vi "SqK_2017.vi"() -> ()   [LabVIEW 2014]
uses:
  <vilib>/vision/Image Controls.llb/IMAQ Image.ctl
  <vilib>/Utility/sysdir.llb/System Directory Type.ctl
  <vilib>/Utility/file.llb/Read From Spreadsheet File (string).vi
  <vilib>/Utility/file.llb/Read From Spreadsheet File (I64).vi
panel:
  out "Video 2":T1(plugin-control)
  out "Boast 13":u8(slide) scale=0.0..54.0
  out "Lob 2":u8(slide) scale=0.0..54.0
  out "Drop 13":u8(slide) scale=0.0..54.0
  out "Boast 1":u8(slide) scale=0.0..54.0
  out "Lob 1":u8(slide) scale=0.0..54.0
  out "Drop 1":u8(slide) scale=0.0..54.0
  in  "Boolean":bool
  out "Min":dbl
  out "sec":dbl
  out "milsec":dbl
  in  "Ddrive":bool
  in  "ASWdrive":bool
  in  "DSWdrive":bool
  in  "SWADrive 12":bool
  in  "SWADrive 11":bool
  in  "SWADrive 10":bool
  in  "SWADrive 9":bool
  in  "SWDDrive 12":bool
  in  "SWDDrive 11":bool
  in  "SWDDrive 10":bool
  in  "SWDDrive 9":bool
  in  "DDrive 12":bool
  in  "DDrive 11":bool
  in  "DDrive 10":bool
  in  "DDrive 9":bool
  in  "DDrive 8":bool
  in  "DDrive 7":bool
  in  "DDrive 6":bool
  in  "DDrive 5":bool
  in  "DDrive":bool
  in  "DDrive 2":bool
  in  "DDrive 3":bool
  in  "DDrive 4":bool
  in  "SWDDrive 8":bool
  in  "SWDDrive 7":bool
  in  "SWDDrive 6":bool
  in  "SWDDrive 5":bool
  in  "SWDDrive":bool
  in  "SWDDrive 2":bool
  in  "SWDDrive 3":bool
  in  "SWDDrive 4":bool
  in  "SWADrive 8":bool
  in  "SWADrive 7":bool
  in  "SWADrive 6":bool
  in  "SWADrive 5":bool
  in  "SWADrive":bool
  in  "SWADrive 2":bool
  in  "SWADrive 3":bool
  in  "SWADrive 4":bool
  out "last saved data":i64[](array[numeric])
  out "Btn 10":string
  out "Btn 9":string
  out "Btn 8":string
  out "Btn 7":string
  out "Btn 6":string
  out "Player 2 data":i64[](array[numeric])
  out "player 1 data":i64[](array[numeric])
  out "both player data":i64[](array[numeric])
  out "Edited data":i64[][](array[numeric])
  out "Event After":i64[][](array[numeric])
  out "Event before":i64[][](array[numeric])
  out "result":i32[](array[numeric])
  out "EVENTS\nTO PLAY":i32[](array[numeric])
  out "Combined data":i64[][](array[numeric])
  out "Extra":i16
  out "Score change":bool[](array[boolean])
  out "last row":i32[](array[numeric])
  out "Player 1/2":i16
  out "Service":i16
  out "Cross":i16
  out "Straight":i16
  out "position":i16
  out "Main tab 2":T2(ring)
  in  "fast rewind":bool
  in  "START":bool
  out "frames to write":i64[][](array[numeric])
  in  "Data file":path caption="Data"
  in  "playback speed":dbl(slide)=1.0 min=0.25 max=1.5 step=0.25 scale=0.25..1.5
  in  "Main tab":enum32{"Coding", "Display"}(tab)
  in  "Player 2":string
  in  "Let":bool
  in  "Nolet1":bool
  in  "Nolet2":bool
  in  "Stroke1":bool
  in  "Stroke2":bool
  in  "Expected Winner1":bool
  in  "Expected Winner2":bool
  in  "Unexpected Winner1":bool
  in  "Unexpected Winner2":bool
  in  "Forced Error1":bool
  in  "Unforced Error1":bool
  in  "Forced Error2":bool
  in  "Unforced Error2":bool
  in  "Pause lag(s)":dbl=1.0 min=0.0 max=2.0 step=0.5 format="%#.1g"
  in  "Code lag(s)":dbl=1.0 min=0.0 max=5.0 step=0.5 format="%#.1g"
  in  "Link Errors":bool
  in  "Btn 1":string
  in  "Btn 2":string
  in  "Btn 3":string
  in  "Btn 4":string
  in  "Btn 5":string
  in  "Button 1":bool
  in  "Button 2":bool
  in  "Button 3":bool
  in  "Button 4":bool
  in  "Button 5":bool
  out "P2":i32
  out "P1":i32
  out "Player1/Player2":bool[](array[boolean])
  in  "Player2":bool
  in  "Player1":bool
  in  "Auto switch":bool
  in  "S6":bool
  in  "S5":bool
  in  "S4":bool
  in  "S3":bool
  in  "S2":bool
  in  "Service1":bool
  in  "Service2":bool
  in  "S1":bool
  in  "5 4":bool
  in  "5 3":bool
  in  "5 2":bool
  in  "5 1":bool
  in  "6 4":bool
  in  "6 3":bool
  in  "6 2":bool
  in  "6 1":bool
  in  "4 4":bool
  in  "4 3":bool
  in  "4 2":bool
  in  "4 1":bool
  in  "3 4":bool
  in  "3 3":bool
  in  "3 2":bool
  in  "3 1":bool
  in  "2 4":bool
  in  "2 3":bool
  in  "2 2":bool
  in  "2 1":bool
  in  "1 4":bool
  in  "1 3":bool
  in  "1 2":bool
  in  "1 1":bool
  in  "after 2":u8(slide)=2 scale=0.0..5.0
  in  "before 2":u8(slide)=2
  in  "Pause lag on":bool
  in  "Undo":bool
  in  "Player 1":string
  in  "ADrive 2":bool
  in  "ADrive":bool
  in  "Drop 2":bool
  in  "lob 2":bool
  in  "Boast 2":bool
  in  "Drop":bool
  in  "lob 13":bool
  in  "Boast":bool
  in  "Chop 2":bool
  in  "Chop":bool
  in  "Smash 2":bool
  in  "Smash":bool
  in  "ADrive 4":bool
  in  "ADrive 3":bool
  in  "Drop 4":bool
  in  "lob 4":bool
  in  "Boast 4":bool
  in  "Drop 3":bool
  in  "lob 3":bool
  in  "Boast 3":bool
  in  "Chop 4":bool
  in  "Chop 3":bool
  in  "Smash 4":bool
  in  "Smash 3":bool
  in  "ADrive 9":bool
  in  "ADrive 10":bool
  in  "Chop 9":bool
  in  "Chop 10":bool
  in  "Drop 9":bool
  in  "lob 9":bool
  in  "Drop 10":bool
  in  "lob 10":bool
  in  "Smash 9":bool
  in  "Smash 10":bool
  in  "Boast 9":bool
  in  "Boast 10":bool
  in  "ADrive 11":bool
  in  "ADrive 12":bool
  in  "Chop 11":bool
  in  "Chop 12":bool
  in  "Drop 11":bool
  in  "lob 11":bool
  in  "Drop 12":bool
  in  "lob 12":bool
  in  "Smash 11":bool
  in  "Smash 12":bool
  in  "Boast 11":bool
  in  "Boast 12":bool
  in  "Smash 8":bool
  in  "Smash 7":bool
  in  "Chop 8":bool
  in  "Chop 7":bool
  in  "Boast 7":bool
  in  "lob 8":bool
  in  "Drop 8":bool
  in  "lob 7":bool
  in  "Drop 7":bool
  in  "Boast 8":bool
  in  "ADrive 8":bool
  in  "ADrive 7":bool
  in  "Smash 6":bool
  in  "Smash 5":bool
  in  "Chop 6":bool
  in  "Chop 5":bool
  in  "Boast 5":bool
  in  "Boast 6":bool
  in  "lob 6":bool
  in  "Drop 6":bool
  in  "lob 5":bool
  in  "Drop 5":bool
  in  "ADrive 6":bool
  in  "ADrive 5":bool
  in  "set":u16(ring) items=["Game 1", "Game 2", "Game 3", "Game 4", "Game 5"]
  in  "Tab Control":T3(tab)
  out "1 9":string
  out "1 11":string
  out "1 12":string
  out "1 13":string
  out "1 8":string
  out "1 15":string
  out "1 16":string
  out "1 17":string
  out "1 18":string
  out "1 19":string
  out "1 20":string
  out "1 21":string
  out "1 23":string
  out "1 24":string
  out "1 25":string
  out "1 26":string
  out "1 27":string
  out "1 28":string
  out "1 29":string
  out "1 30":string
  out "1 31":string
  out "1 33":string
  out "1 34":string
  out "1 35":string
  out "1 36":string
  out "1 37":string
  out "1 38":string
  out "1 39":string
  out "1 40":string
  out "1 41":string
  out "1 43":string
  out "1 44":string
  out "1 45":string
  out "1 46":string
  out "1 47":string
  out "1 48":string
  out "1 49":string
  out "1 50":string
  out "1 51":string
  out "1 52":string
  out "1 53":string
  out "1 54":string
  out "1 55":string
  out "1 56":string
  out "1 57":string
  out "1 58":string
  out "1 59":string
  out "1 60":string
  out "Volley 1":string="0"
  out "Straight 1":string="0"
  out "Bounce 1":string="0"
  out "Cross 1":string="0"
  out "B-hand 1":string="0"
  out "F-hand 1":string="0"
  out "H-volley 1":string="0"
  in  "Fh":string="Forehand"
  in  "BH 3":string="Backhand"
  in  "Cross 5":string="Cross"
  in  "bounce":string="Bounce"
  in  "Straight 5":string="Straight"
  in  "volley":string="Volley"
  in  "H-volley":string="Half volley"
  out "H-volley 3":string="0"
  out "Volley 3":string="0"
  out "Straight 3":string="0"
  out "Bounce 3":string="0"
  out "Cross 3":string="0"
  out "B-hand 2":string="0"
  out "F-hand 2":string="0"
  in  "H-volley 2":string="Half volley"
  in  "volley 2":string="Volley"
  in  "Straight 6":string="Straight"
  in  "bounce 2":string="Bounce"
  in  "Cross 6":string="Cross"
  in  "BH 4":string="Backhand"
  in  "Fh 2":string="Forehand"
  out "UF err1 num":string="0"
  out "F err1 num":string="0"
  out "UNex win1 num":string="0"
  out "ex win1 num":string="0"
  in  "UNex win1":string="Unexpected winner"
  in  "ex win1":string="Expected winner"
  out "Stroke 3":string="0"
  in  "Stroke 1":string="Stroke"
  in  "UF err1":string="Unforced error"
  in  "F err1":string="Forced error"
  out "Let 3":string="0"
  out "No Let 1":string="0"
  in  "Let 1":string="Let "
  in  "No let 1":string="No let"
  out "UF err2 num":string="0"
  out "F err2 num":string="0"
  out "UNex win2 num":string="0"
  out "ex win2 num":string="0"
  in  "UF err2":string="Unforced error"
  in  "F err2":string="Forced error"
  in  "UNex win2":string="Unexpected winner"
  in  "ex win2":string="Expected winner"
  out "Stroke 4":string="0"
  out "Let 4":string="0"
  out "No Let 2":string="0"
  in  "Stroke 2":string="Stroke"
  in  "Let  5":string="Let"
  in  "No let 2":string="No let"
  out "Volley 4":u8(slide) scale=0.0..54.0
  out "Bounce 4":u8(slide) scale=0.0..54.0
  out "Cross 4":u8(slide) scale=0.0..54.0
  out "Straight 4":u8(slide) scale=0.0..54.0
  out "BH 1":u8(slide) scale=0.0..54.0
  out "FH 1":u8(slide) scale=0.0..54.0
  out "Drive 1":u8(slide) scale=0.0..54.0
  out "Player 1 shots numbers":string[](array[string])=["0", "0", "0", "0", "", " ", "0", "0", "", "0", "0", "", "0", "0"]
  in  "Player 1 shots":string[](array[string])=["Drive", "Drop", "Chop", "Lob", "Boast 2", "Boast 3", "Kill", "", "", "", "", "", "F-hand", "B-hand", "", "Straight", "Cross", "", "Bounce", "Volley", "H-volley"]
  out "Volley 2":u8(slide) scale=0.0..54.0
  out "Bounce 2":u8(slide) scale=0.0..54.0
  out "Cross 2":u8(slide) scale=0.0..54.0
  out "Straight 2":u8(slide) scale=0.0..54.0
  out "BH 2":u8(slide) scale=0.0..54.0
  out "FH 2":u8(slide) scale=0.0..54.0
  out "Drive 2":u8(slide) scale=0.0..54.0
  out "Player 2 shots numbers":string[](array[string])=["0", "0", "0", "0", "", " ", "0", "0", "", "0", "0", "", "0", "0"]
  in  "Player 2 shots":string[](array[string])=["Drive", "Drop", "Chop", "Lob", "Boast 2", "Boast 3", "Kill", "", "", "", "", "", "F-hand", "B-hand", "", "Straight", "Cross", "", "Bounce", "Volley", "H-volley"]
  in  "before n after":i32(slide) scale=-5.0..5.0
  in  "display\nselection":string(combo)="1"
  in  "Extract data":bool
  in  "Upload edited video":bool
  in  "1 10":bool
  in  "1 7":bool
  in  "1 6":bool
  in  "1 5":bool
  in  "2 10":bool
  in  "2 7":bool
  in  "2 6":bool
  in  "2 5":bool
  in  "3 9":bool
  in  "3 7":bool
  in  "3 6":bool
  in  "3 5":bool
  in  "4 9":bool
  in  "4 7":bool
  in  "4 6":bool
  in  "4 5":bool
  in  "Boast3":bool
  in  "Boast2":bool
  in  "Drop 14":bool
  in  "Chop 13":bool
  in  "Adrive":bool
  in  "Lob":bool
  in  "Smash 13":bool
  in  "FH":bool
  in  "BH":bool
  in  "ST":bool
  in  "CR":bool
  in  "Bounce":bool
  in  "Half Volley":bool
  in  "Volley":bool
  in  "before":u8(slide)=2
  in  "after":u8(slide)=2 scale=0.0..5.0
  in  "Combine":bool
  in  "Player2 2":bool
  in  "Player1 2":bool
  in  "S6 2":bool
  in  "S5 2":bool
  in  "S4 2":bool
  in  "S1 2":bool
  in  "Service2 2":bool
  in  "Service1 2":bool
  in  "S2 2":bool
  in  "S3 2":bool
  in  "Let 2":bool
  in  "Nolet2 2":bool
  in  "Nolet1 2":bool
  in  "Stroke2 2":bool
  in  "Stroke1 2":bool
  in  "Unforced Error2 2":bool
  in  "Forced Error2 2":bool
  in  "Unforced Error1 2":bool
  in  "Forced Error1 2":bool
  in  "Unexpected Winner2 2":bool
  in  "Unexpected Winner1 2":bool
  in  "Expected Winner2 2":bool
  in  "Expected Winner1 2":bool
  out "Video files to write":string[](array[string])
  in  "Video compress":bool=TRUE
  in  "Abort":bool
  in  "Write file":bool
  in  "Delete":bool[](array[boolean])
  out "Writing":u32(slide) scale=0.0..404.0
  in  "File name":string
  in  "Add to lib":bool
  in  "Video to write":path caption="Folder"
  in  "Examine code":bool
  in  "Update":bool
  in  "Reset":bool
  in  "Code number display":i32 min=1 max=1
  in  "Next":bool
  in  "Previous":bool
  in  "6 5":bool
  in  "6 6":bool
  in  "6 7":bool
  in  "6 8":bool
  in  "5 5":bool
  in  "5 6":bool
  in  "5 7":bool
  in  "5 8":bool
  in  "Button 7":bool
  in  "Button 8":bool
  in  "Button 9":bool
  in  "Button 10":bool
  in  "Button 6":bool
  in  "playback interval on":bool
  in  "clear all":bool
  in  "G5":bool
  in  "G4":bool
  in  "G1":bool
  in  "G2":bool
  in  "G3":bool
  in  "Load video":bool
  in  "Play":bool
  out "ful video frames":i64[](array[numeric])
  out "playback speed":dbl
  out "Number of Frames":u32
  out "framesPerSecond":u32
  out "Last Edit":bool[](array[boolean])
  out "frames 2 play":i64[](array[numeric])
  in  "stop":bool
  out "Video Frame":u32
  out "edited\nevents":i64[][](array[numeric])
  out "edited to play":i64[](array[numeric])
  out "frames edited":i64[](array[numeric])
  in  "fast forward":bool
  in  "Pause":bool
  out "coding":i64[][](array[numeric])
  in  "Progress...":u32(slide) min=400 max=47374 scale=-1.1..56740.0
  in  "Video file":path caption="Video"
  out "task":i32(slide) scale=0.0..300.0
  out "Video":T1(plugin-control)
  # "© 2016 National Sports Institute of Malaysia All Rights Reserved"
  # "Position"
  # "Bounce"
  # "Volley"
  # "Half volley"
  # "Forehand"
  # "Backhand"
  # "Backhand"
  # "Forehand"
  # "Backhand"
  # "Forehand"
  # "St"
  # "Cr"
  # "St"
  # "Cr"
  # "St"
  # "Cr"
  # "St"
  # "Cr"
  # "St"
  # "Cr"
  # "St"
  # "Cr"
  # "Drop"
  # "Chop"
  # "Lob"
  # "Boast"
  # "Kill"
  # "Drive"
  # "Lead and lag settings"
  # "Game"
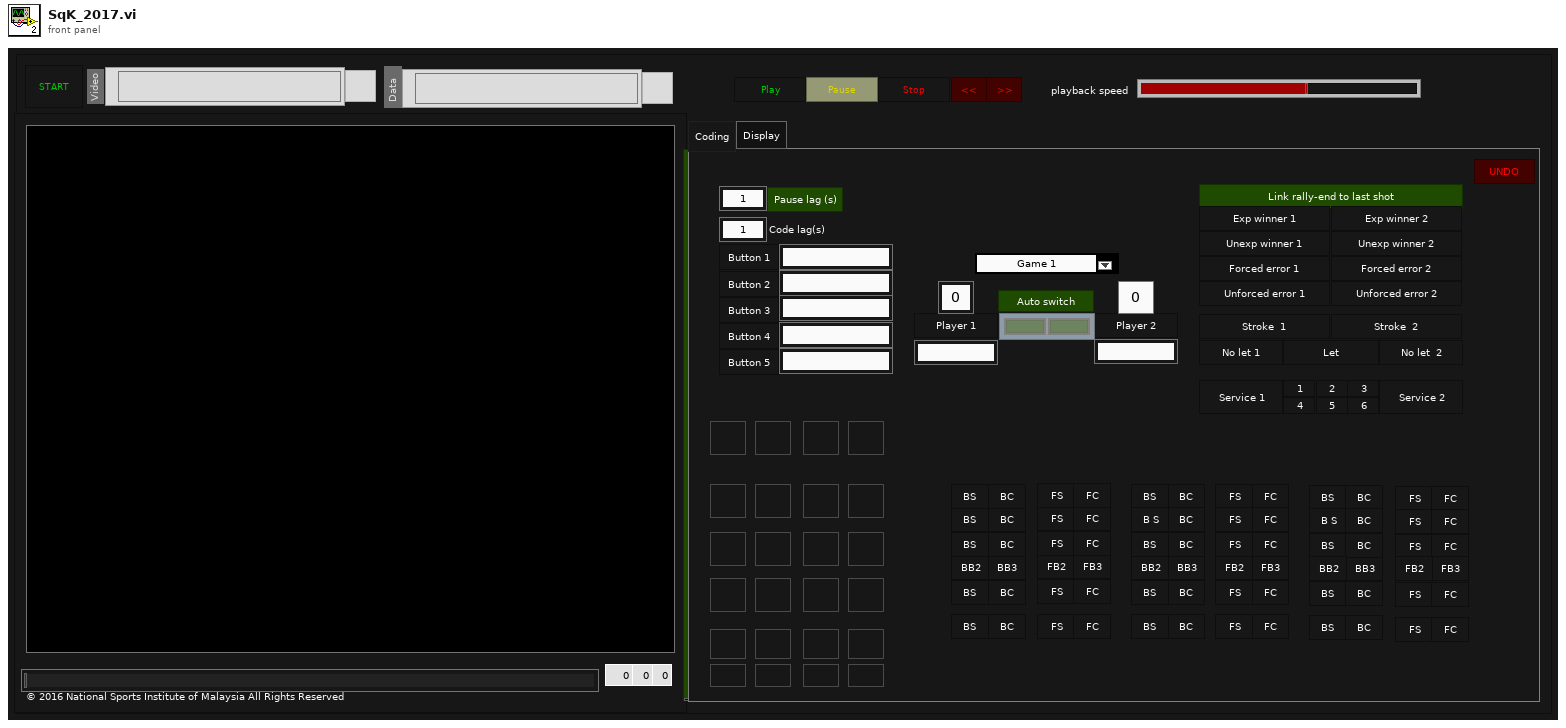
[diagram p1: front panel]
types:
  T1 = typedef "IMAQ Image.ctl" = refnum<image>
  T2 = enum32{"Coding", "Edit video", "Examine coding", "Display", "Update coding", "Edit coding"}
  T3 = enum32{"                                                                       click here to copy"}
  T4 = enum16{"open", "replace", "create", "open or create", "replace or create", "replace or create with confirmation"}
  T5 = enum8{"Enabled", "Disabled", "Disabled and Grayed Out"}
  T6 = enum32{"Coding", "Edit video", "Examine coding", "Display", "Update coding", "Edit coding", "Clear all"}
  T7 = typedef "System Directory Type.ctl" = i32
  T8 = typedef "Image Type" = u32
  T9 = typedef "AviRefnum.ctl" = refnum<k1>
  T10 = cluster{"width":u32, "height":u32, "framesPerSecond":u32, "compressionFilter":string, "hasData":bool}
  T11 = typedef "eventvkey.ctl" = enum16{"ASCII", "Enter", "Return", "Shift", "Ctrl", "Alt", "Cmd", "Opt", "Caps", "NumLock", "Clear", "Break", "Up", "Down", "Left", "Right", "Insert", "Delete", "Home", "End", "PageUp", "PageDown", "Escape", "Help", "Pause", "ScrollLock", "F1", "F2", "F3", "F4", "F5", "F6", "F7", "F8", "F9", "F10", "F11", "F12", "F13", "F14", "F15", "F16", "F17", "F18", "F19", "F20", "F21", "F22", "F23", "F24", "Play", "VolumeUp", "VolumeDown", "Mute", "Two Byte Char"}
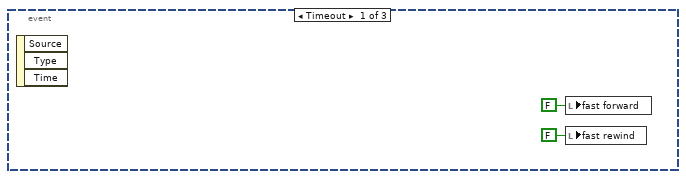
[diagram p2: hidden frame]
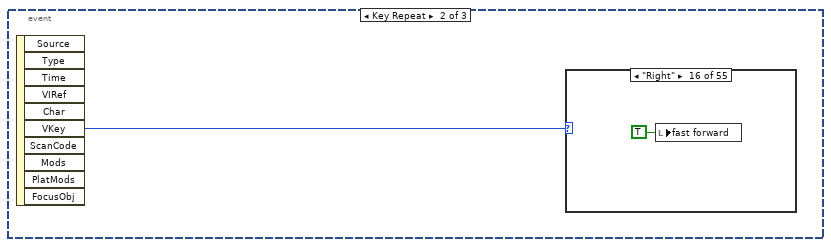
[diagram p3: hidden frame]
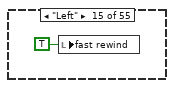
[diagram p18: hidden frame]
diagram:
  w1 = FALSE ("player2")
  n1 = while {
    stop <- FALSE stop-if-true
    n2 = flat-sequence {
      tunnel: [w43] -> w14
      tunnel: [w44] -> w15
      tunnel: w15 -> [w141]
      tunnel: w14 -> [w140]
      tunnel: [w140] -> w13
      tunnel: [w141] -> w12
      tunnel: w13 -> [w196]
      tunnel: w12 -> [w180]
      tunnel: [w169] -> w10
      tunnel: [w179] -> w9
      tunnel: [w178] -> w8
      tunnel: [w177] -> w2
      tunnel: [w176] -> w7
      frame #0 {
        w33 = T7 1 items=["User Home"=0, "User Desktop"=1, "User Documents"=2, "User Application Data"=3, "User Preferences"=4, "User Temporary"=5, "Public Documents"=6, "Public Application Data"=7, "Public Preferences"=8, "Public Cache"=13, "System Core Libraries"=9, "System Installed Libraries"=10, "Application Files"=11, "Boot Volume Root"=12] ("system directory type")
        w36 = T5."Enabled" ("Disabled")
        w38 = u32 0 ("Progress...")
        w35 = FALSE ("START")
        w34 = T5."Disabled and Grayed Out" ("Disabled")
        n3 = call <vilib>:"Get System Directory.vi"("system directory type"=w33) -> ("system directory"=w32:path)  [unwired: 10 in]
        n4 = property on="Video file" class="Path"("StartPath"=w32) -> ()  [unwired: 2 in, 2 out]
        n5 = property on="Video to write" class="Path"("StartPath"=w32) -> ()  [unwired: 2 in, 2 out]
        n6 = property on="Data file" class="Path"("StartPath"=w32) -> ()  [unwired: 2 in, 2 out]
        n7 = property on="Play" class="Bool (strict)"("DisabledEnum"=w34, "Value"=w35) -> ()  [unwired: 2 in, 2 out]
        n8 = property on="stop" class="Bool (strict)"("DisabledEnum"=w34, "Value"=w35) -> ()  [unwired: 2 in, 2 out]
        n9 = property on="Pause" class="Bool (strict)"("DisabledEnum"=w34, "Value"=w35) -> ()  [unwired: 2 in, 2 out]
        n10 = property on="fast forward" class="Bool (strict)"("DisabledEnum"=w34, "Value"=w35) -> ()  [unwired: 2 in, 2 out]
        n11 = property on="playback speed" class="Slide (strict)"("DisabledEnum"=w34, "Value"=1.0 ("playback speed")) -> ()  [unwired: 2 in, 2 out]
        n12 = property on="Main tab" class="TabCtl (strict)"("DisabledEnum"=w34, "Value"=enum32{"Coding", "Display"}."Coding" ("Main tab")) -> ()  [unwired: 2 in, 2 out]
        n13 = property on="Progress..." class="Slide (strict)"("DisabledEnum"=w34, "Value"=w38) -> ()  [unwired: 2 in, 2 out]
        n14 = property on="Video Frame" class="DigNum (strict)"("DisabledEnum"=w34, "Value"=w38) -> ()  [unwired: 2 in, 2 out]
        n15 = property on="Video" class="ImageControl"("DisabledEnum"=w34, "Value"=T1 refnum ("Video")) -> ()  [unwired: 2 in, 2 out]
        n16 = property on="START" class="Bool (strict)"("DisabledEnum"=w36, "Value"=w35) -> ()  [unwired: 2 in, 2 out]
        n17 = property on="Video file" class="Path"("DisabledEnum"=w36) -> ()  [unwired: 2 in, 2 out]
        n18 = property on="Data file" class="Path"("DisabledEnum"=w36) -> ()  [unwired: 2 in, 2 out]
        n19 = property on="fast rewind" class="Bool (strict)"("DisabledEnum"=w34, "Value"=w35) -> ()  [unwired: 2 in, 2 out]
      }
      frame #1 {
        n20 = while {
          tunnel: [w46] -> w44
          tunnel: [w45] -> w43
          stop <- w47 stop-if-true
          n21 = case shown="True" "START" {
            tunnel: [FALSE w52] -> w47
            tunnel: [w49 w55] -> w46
            tunnel: [w49 w54] -> w45
            frame False {
              w49 = path "" ("dup path")
              n22 = Wait (ms)(milliseconds to wait=u32 200) -> ()  [unwired: 1 out]
            }
            frame True {
              n23 = Path To String(path="Data file") -> (string=w64:string)
              n24 = Wait (ms)(milliseconds to wait=u32 200) -> ()  [unwired: 1 out]
              n25 = Empty String/Path?(string/path=w64) -> (empty?=w63:bool)
              n26 = case shown="False" w63 {
                tunnel: "Data file" -> [w85 w110]
                tunnel: [w84 FALSE] -> w61
                tunnel: [w83 w110] -> w54
                frame False {
                  n27 = Strip Path(path=w85) -> (stripped path=w90:path)  [unwired: 1 out]
                  n28 = Path To String(path=w90) -> (string=w89:string)
                  n29 = call <vilib>:"Get File Extension.vi"("file"=w85) -> ("filename without extension"=w92:string)  [unwired: 7 in, 3 out]
                  n30 = Concatenate Strings(w89, "\\" ("string"), w92, ".xls" ("string")) -> (w91:string)
                  n31 = String To Path(string=w91) -> (path=w86:path)
                  n32 = call <vilib>:"Check if File or Folder Exists.vi"("path"=w86) -> ("file or folder exists?"=w87:bool)  [unwired: 8 in, 2 out]
                  n33 = case shown="False" w87 {
                    selector: w87 -> [_ w109]
                    tunnel: w86 -> [w96 w108]
                    tunnel: [w95 w109] -> w84
                    tunnel: [w94 w108] -> w83
                    frame False {
                      n34 = Two Button Dialog(message="This data file does not exist.\nDo you wish to start a new project?", 1:"No" ("F button name (\"Cancel\")"), 2:"Yes" ("T button name (\"OK\")")) -> (T button?=w97:bool)
                      n35 = case shown="False" w97 {
                        selector: w97 -> [w102 w104]
                        tunnel: w96 -> [_ w103]
                        tunnel: [w102 w104] -> w95
                        tunnel: [path "" ("dup path") w103] -> w94
                        frame False {
                        }
                        frame True {
                          n36 = Open/Create/Replace File(file path (use dialog)=w103, operation (0:open)=T4."create") -> (refnum out=w105:refnum<file>, error out=w107:errorcluster)  [unwired: 4 in, 1 out]
                          n37 = Close File(refnum=w105, error in=w107) -> ()  [unwired: 2 out]
                        }
                      }
                    }
                    frame True {
                    }
                  }
                }
                frame True {
                  n38 = One Button Dialog(message="Please enter data file") -> ()  [unwired: 1 in, 1 out]
                }
              }
              n39 = Path To String(path="Video file") -> (string=w59:string)
              n40 = Empty String/Path?(string/path=w59) -> (empty?=w58:bool)
              n41 = case shown="True" w58 {
                selector: w58 -> [_ w82]
                tunnel: "Video file" -> [w69 w80]
                tunnel: [w66 w80] -> w55
                tunnel: [w65 w82] -> w56
                frame False {
                  n42 = call <vilib>:"Check if File or Folder Exists.vi"("path"=w69) -> ("file or folder exists?"=w73:bool, "dup path"=w67:path)  [unwired: 8 in, 1 out]
                  n43 = call <vilib>:"Get File Extension.vi"("file"=w69) -> ("lowercase file extension"=w70:string)  [unwired: 7 in, 3 out]
                  n44 = Not(x=w73) -> (.not. x?=w74:bool)
                  n45 = Not Equal?(x=w70, y="avi" ("lowercase file extension")) -> (x != y?=w72:bool)
                  n46 = Or(x=w74, y=w72) -> (x .or. y?=w68:bool)
                  n47 = case shown="True" w68 {
                    selector: w68 -> [w75 w77]
                    tunnel: w67 -> [w76 _]
                    tunnel: [w76 path "" ("dup path")] -> w66
                    tunnel: [w75 w77] -> w65
                    frame False {
                    }
                    frame True {
                      n48 = One Button Dialog(message="You have chosen an invalid video file for coding\n\nPossible reasons\n1)\tChosen video file format was not AVI\n2)\tChosen video file does not exist") -> ()  [unwired: 1 in, 1 out]
                    }
                  }
                }
                frame True {
                  n49 = One Button Dialog(message="Please enter video file") -> ()  [unwired: 1 in, 1 out]
                }
              }
              n50 = Not(x=w56) -> (.not. x?=w60:bool)
              n51 = local write "Video file"(w55) -> ()
              n52 = And(x=w60, y=w61) -> (x .and. y?=w52:bool)
              n53 = local write "Data file"(w54) -> ()
              n54 = local write "START"(w52) -> ()
            }
          }
        }
        n55 = local write "Boolean"(TRUE ("Boolean")) -> ()
        n56 = property on="Video 2" class="ImageControl"("Visible"=FALSE) -> ()  [unwired: 2 in, 2 out]
      }
      frame #2 {
        w120 = i64[] [] ("to write")
        w136 = 0 ("P1")
        w114 = FALSE ("4 6")
        w121 = TRUE ("4 6")
        w156 = FALSE ("4 6")
        w154 = TRUE ("Extract data")
        w122 = u8 2 ("before")
        w139 = T5."Disabled and Grayed Out" ("Disabled")
        w159 = u32 0 ("Progress...")
        w142 = FALSE ("START")
        w143 = T5."Enabled" ("Disabled")
        n57 = property on="Play" class="Bool (strict)"("DisabledEnum"=w143, "Value"=w142) -> ()  [unwired: 2 in, 2 out]
        n58 = property on="stop" class="Bool (strict)"("DisabledEnum"=w143, "Value"=w142) -> ()  [unwired: 2 in, 2 out]
        n59 = property on="Pause" class="Bool (strict)"("DisabledEnum"=w143, "Value"=w142) -> ()  [unwired: 2 in, 2 out]
        n60 = property on="fast forward" class="Bool (strict)"("DisabledEnum"=w143, "Value"=w142) -> ()  [unwired: 2 in, 2 out]
        n61 = property on="fast rewind" class="Bool (strict)"("DisabledEnum"=w143, "Value"=w142) -> ()  [unwired: 2 in, 2 out]
        n62 = property on="playback speed" class="Slide (strict)"("DisabledEnum"=w143, "Value"=1.0 ("playback speed")) -> ()  [unwired: 2 in, 2 out]
        n63 = property on="Main tab" class="TabCtl (strict)"("DisabledEnum"=w143, "Value"=enum32{"Coding", "Display"}."Coding" ("Main tab")) -> ()  [unwired: 2 in, 2 out]
        n64 = property on="Progress..." class="Slide (strict)"("DisabledEnum"=w143, "Value"=w159) -> ()  [unwired: 2 in, 2 out]
        n65 = property on="Video Frame" class="DigNum (strict)"("DisabledEnum"=w143, "Value"=w159) -> ()  [unwired: 2 in, 2 out]
        n66 = property on="Video" class="ImageControl"("DisabledEnum"=w143) -> ()  [unwired: 2 in, 2 out]
        n67 = property on="Video file" class="Path"("DisabledEnum"=w139) -> ()  [unwired: 2 in, 2 out]
        n68 = property on="Data file" class="Path"("DisabledEnum"=w139) -> ()  [unwired: 2 in, 2 out]
        n69 = property on="Code number display" class="DigNum (strict)"("DisabledEnum"=w139) -> ()  [unwired: 2 in, 2 out]
        n70 = property on="Next" class="Bool (strict)"("DisabledEnum"=w139) -> ()  [unwired: 2 in, 2 out]
        n71 = property on="Reset" class="Bool (strict)"("DisabledEnum"=w139) -> ()  [unwired: 2 in, 2 out]
        n72 = property on="Update" class="Bool (strict)"("DisabledEnum"=w139) -> ()  [unwired: 2 in, 2 out]
        n73 = property on="Previous" class="Bool (strict)"("DisabledEnum"=w139) -> ()  [unwired: 2 in, 2 out]
        n74 = local write "Pause lag(s)"(1.0 ("Pause lag(s)")) -> ()
        n75 = local write "Code lag(s)"(0.5 ("Code lag(s)")) -> ()
        n76 = local write "Link Errors"(TRUE ("Link Errors")) -> ()
        n77 = local write "Pause lag on"(w121) -> ()
        n78 = local write "playback interval on"(w121) -> ()
        n79 = local write "Auto switch"(w121) -> ()
        n80 = local write "Last Edit"(bool[] [FALSE, FALSE, FALSE, FALSE, FALSE, FALSE, FALSE, FALSE, FALSE, FALSE, FALSE, FALSE, FALSE, FALSE, FALSE, FALSE, FALSE, FALSE, FALSE, FALSE, FALSE, FALSE, FALSE, FALSE, FALSE, FALSE, FALSE, FALSE, FALSE, FALSE, FALSE, FALSE, FALSE, FALSE, FALSE, FALSE] ("Last Edit")) -> ()
        n81 = local write "File name"("" ("File name")) -> ()
        n82 = local write "Code number display"(1 ("Code number display")) -> ()
        n83 = local write "Delete"(bool[] [TRUE, TRUE, TRUE, TRUE, TRUE] ("Array 2")) -> ()
        n84 = local write "Video compress"(w154) -> ()
        n85 = local write "Extract data"(w154) -> ()
        n86 = local write "Upload edited video"(w156) -> ()
        n87 = local write "Add to lib"(w156) -> ()
        n88 = local write "Abort"(w156) -> ()
        n89 = local write "Write file"(w156) -> ()
        n90 = local write "Examine code"(w156) -> ()
        n91 = local write "Update"(w156) -> ()
        n92 = local write "Reset"(w156) -> ()
        n93 = local write "Previous"(w156) -> ()
        n94 = local write "Next"(w156) -> ()
        n95 = local write "before"(w122) -> ()
        n96 = local write "after"(w122) -> ()
        n97 = local write "before 2"(w122) -> ()
        n98 = local write "after 2"(w122) -> ()
        n99 = call-poly <vilib>:"Read From Spreadsheet File.vi"("file path (dialog if empty)"=w140) -> ("all rows"=w128:string[][])  [unwired: 6 in, 4 out]
        n100 = Index Array(array=w128, index (row)=3) -> (element=w130:string[])  [unwired: 1 in]
        n101 = Index Array(array=w130, index #1=71 ("index"), index #2=72 ("index"), index #3=73 ("index"), index #4=74 ("index"), index #5=75 ("index"), index #6=69 ("index"), index #7=70 ("index")) -> (element #1=w125:string, element #2=w126:string, element #3=w127:string, element #4=w124:string, element #5=w123:string, element #6=w116:string, element #7=w115:string)
        n102 = local write "display\nselection"("1" ("display\nselection")) -> ()
        n103 = local write "task"(300 ("task")) -> ()
        n104 = local write "Load video"(FALSE ("Pause")) -> ()
        n105 = local write "Video files to write"(string[] [] ("Video files to write")) -> ()
        n106 = local write "frames to write"(i64[][] [] ("to write")) -> ()
        n107 = local write "player 1 data"(w120) -> ()
        n108 = local write "both player data"(w120) -> ()
        n109 = local write "Player 2 data"(w120) -> ()
        n110 = local write "last saved data"(w120) -> ()
        n111 = local write "Btn 1"(w125) -> ()
        n112 = local write "Btn 2"(w126) -> ()
        n113 = local write "Btn 3"(w127) -> ()
        n114 = local write "Btn 4"(w124) -> ()
        n115 = local write "Btn 5"(w123) -> ()
        n116 = local write "Player 1"(w116) -> ()
        n117 = local write "Player 2"(w115) -> ()
        n118 = local write "P1"(w136) -> ()
        n119 = local write "P2"(w136) -> ()
        n120 = local write "Drop"(w114) -> ()
        n121 = local write "Drop 2"(w114) -> ()
        n122 = local write "Drop 3"(w114) -> ()
        n123 = local write "Drop 4"(w114) -> ()
        n124 = local write "Drop 5"(w114) -> ()
        n125 = local write "Drop 6"(w114) -> ()
        n126 = local write "Drop 7"(w114) -> ()
        n127 = local write "Drop 8"(w114) -> ()
        n128 = local write "Drop 9"(w114) -> ()
        n129 = local write "Drop 10"(w114) -> ()
        n130 = local write "Drop 11"(w114) -> ()
        n131 = local write "Drop 12"(w114) -> ()
        n132 = local write "Chop"(w114) -> ()
        n133 = local write "Chop 2"(w114) -> ()
        n134 = local write "Chop 3"(w114) -> ()
        n135 = local write "Chop 4"(w114) -> ()
        n136 = local write "Chop 5"(w114) -> ()
        n137 = local write "Chop 6"(w114) -> ()
        n138 = local write "Chop 7"(w114) -> ()
        n139 = local write "Chop 8"(w114) -> ()
        n140 = local write "Chop 9"(w114) -> ()
        n141 = local write "Chop 10"(w114) -> ()
        n142 = local write "Chop 11"(w114) -> ()
        n143 = local write "Chop 12"(w114) -> ()
        n144 = local write "Player2 2"(w114) -> ()
        n145 = local write "Player1 2"(w114) -> ()
        n146 = local write "Button 7"(w114) -> ()
        n147 = local write "Button 8"(w114) -> ()
        n148 = local write "Button 9"(w114) -> ()
        n149 = local write "Button 10"(w114) -> ()
        n150 = local write "Button 6"(w114) -> ()
        n151 = local write "S6 2"(w114) -> ()
        n152 = local write "S5 2"(w114) -> ()
        n153 = local write "S4 2"(w114) -> ()
        n154 = local write "S1 2"(w114) -> ()
        n155 = local write "Service2 2"(w114) -> ()
        n156 = local write "Service1 2"(w114) -> ()
        n157 = local write "S2 2"(w114) -> ()
        n158 = local write "S3 2"(w114) -> ()
        n159 = local write "lob 13"(w114) -> ()
        n160 = local write "lob 2"(w114) -> ()
        n161 = local write "lob 3"(w114) -> ()
        n162 = local write "lob 4"(w114) -> ()
        n163 = local write "lob 5"(w114) -> ()
        n164 = local write "lob 6"(w114) -> ()
        n165 = local write "lob 7"(w114) -> ()
        n166 = local write "lob 8"(w114) -> ()
        n167 = local write "lob 9"(w114) -> ()
        n168 = local write "lob 10"(w114) -> ()
        n169 = local write "lob 11"(w114) -> ()
        n170 = local write "lob 12"(w114) -> ()
        n171 = local write "Smash"(w114) -> ()
        n172 = local write "Smash 2"(w114) -> ()
        n173 = local write "Smash 3"(w114) -> ()
        n174 = local write "Smash 4"(w114) -> ()
        n175 = local write "Smash 5"(w114) -> ()
        n176 = local write "Smash 6"(w114) -> ()
        n177 = local write "Smash 7"(w114) -> ()
        n178 = local write "Smash 8"(w114) -> ()
        n179 = local write "Smash 9"(w114) -> ()
        n180 = local write "Smash 10"(w114) -> ()
        n181 = local write "Smash 11"(w114) -> ()
        n182 = local write "Smash 12"(w114) -> ()
        n183 = local write "4 5"(w114) -> ()
        n184 = local write "4 6"(w114) -> ()
        n185 = local write "4 7"(w114) -> ()
        n186 = local write "4 9"(w114) -> ()
        n187 = local write "3 5"(w114) -> ()
        n188 = local write "3 6"(w114) -> ()
        n189 = local write "3 7"(w114) -> ()
        n190 = local write "3 9"(w114) -> ()
        n191 = local write "2 5"(w114) -> ()
        n192 = local write "2 6"(w114) -> ()
        n193 = local write "2 7"(w114) -> ()
        n194 = local write "2 10"(w114) -> ()
        n195 = local write "1 5"(w114) -> ()
        n196 = local write "1 6"(w114) -> ()
        n197 = local write "1 7"(w114) -> ()
        n198 = local write "1 10"(w114) -> ()
        n199 = local write "6 5"(w114) -> ()
        n200 = local write "6 6"(w114) -> ()
        n201 = local write "6 7"(w114) -> ()
        n202 = local write "6 8"(w114) -> ()
        n203 = local write "5 5"(w114) -> ()
        n204 = local write "5 6"(w114) -> ()
        n205 = local write "5 7"(w114) -> ()
        n206 = local write "5 8"(w114) -> ()
        n207 = local write "Half Volley"(w114) -> ()
        n208 = local write "ADrive"(w114) -> ()
        n209 = local write "ADrive 2"(w114) -> ()
        n210 = local write "ADrive 3"(w114) -> ()
        n211 = local write "ADrive 4"(w114) -> ()
        n212 = local write "ADrive 5"(w114) -> ()
        n213 = local write "ADrive 6"(w114) -> ()
        n214 = local write "ADrive 7"(w114) -> ()
        n215 = local write "ADrive 8"(w114) -> ()
        n216 = local write "ADrive 9"(w114) -> ()
        n217 = local write "ADrive 10"(w114) -> ()
        n218 = local write "ADrive 11"(w114) -> ()
        n219 = local write "ADrive 12"(w114) -> ()
        n220 = local write "DDrive"(w114) -> ()
        n221 = local write "DDrive 2"(w114) -> ()
        n222 = local write "DDrive 3"(w114) -> ()
        n223 = local write "DDrive 4"(w114) -> ()
        n224 = local write "DDrive 5"(w114) -> ()
        n225 = local write "DDrive 6"(w114) -> ()
        n226 = local write "DDrive 7"(w114) -> ()
        n227 = local write "DDrive 8"(w114) -> ()
        n228 = local write "DDrive 9"(w114) -> ()
        n229 = local write "DDrive 10"(w114) -> ()
        n230 = local write "DDrive 11"(w114) -> ()
        n231 = local write "DDrive 12"(w114) -> ()
        n232 = local write "Smash 13"(w114) -> ()
        n233 = local write "Boast3"(w114) -> ()
        n234 = local write "DSWdrive"(w114) -> ()
        n235 = local write "Lob"(w114) -> ()
        n236 = local write "ASWdrive"(w114) -> ()
        n237 = local write "Adrive"(w114) -> ()
        n238 = local write "Ddrive"(w114) -> ()
        n239 = local write "Chop 13"(w114) -> ()
        n240 = local write "Drop 14"(w114) -> ()
        n241 = local write "Boast2"(w114) -> ()
        n242 = local write "FH"(w114) -> ()
        n243 = local write "BH"(w114) -> ()
        n244 = local write "ST"(w114) -> ()
        n245 = local write "CR"(w114) -> ()
        n246 = local write "Bounce"(w114) -> ()
        n247 = local write "Volley"(w114) -> ()
        n248 = local write "SWADrive"(w114) -> ()
        n249 = local write "SWADrive 2"(w114) -> ()
        n250 = local write "SWADrive 3"(w114) -> ()
        n251 = local write "SWADrive 4"(w114) -> ()
        n252 = local write "SWADrive 5"(w114) -> ()
        n253 = local write "SWADrive 6"(w114) -> ()
        n254 = local write "SWADrive 7"(w114) -> ()
        n255 = local write "SWADrive 8"(w114) -> ()
        n256 = local write "SWADrive 9"(w114) -> ()
        n257 = local write "SWADrive 10"(w114) -> ()
        n258 = local write "SWADrive 11"(w114) -> ()
        n259 = local write "SWADrive 12"(w114) -> ()
        n260 = local write "SWDDrive"(w114) -> ()
        n261 = local write "SWDDrive 2"(w114) -> ()
        n262 = local write "SWDDrive 3"(w114) -> ()
        n263 = local write "SWDDrive 4"(w114) -> ()
        n264 = local write "SWDDrive 5"(w114) -> ()
        n265 = local write "SWDDrive 6"(w114) -> ()
        n266 = local write "SWDDrive 7"(w114) -> ()
        n267 = local write "SWDDrive 8"(w114) -> ()
        n268 = local write "SWDDrive 9"(w114) -> ()
        n269 = local write "SWDDrive 10"(w114) -> ()
        n270 = local write "SWDDrive 11"(w114) -> ()
        n271 = local write "SWDDrive 12"(w114) -> ()
        n272 = local write "Let 2"(w114) -> ()
        n273 = local write "Nolet2 2"(w114) -> ()
        n274 = local write "Nolet1 2"(w114) -> ()
        n275 = local write "Stroke2 2"(w114) -> ()
        n276 = local write "Stroke1 2"(w114) -> ()
        n277 = local write "Unforced Error2 2"(w114) -> ()
        n278 = local write "Forced Error2 2"(w114) -> ()
        n279 = local write "Unforced Error1 2"(w114) -> ()
        n280 = local write "Forced Error1 2"(w114) -> ()
        n281 = local write "Unexpected Winner2 2"(w114) -> ()
        n282 = local write "Unexpected Winner1 2"(w114) -> ()
        n283 = local write "Expected Winner2 2"(w114) -> ()
        n284 = local write "Expected Winner1 2"(w114) -> ()
        n285 = local write "clear all"(w114) -> ()
        n286 = local write "G5"(w114) -> ()
        n287 = local write "G4"(w114) -> ()
        n288 = local write "G1"(w114) -> ()
        n289 = local write "G2"(w114) -> ()
        n290 = local write "G3"(w114) -> ()
        n291 = local write "Combine"(w114) -> ()
        n292 = local write "Undo"(w114) -> ()
        n293 = local write "Boast"(w114) -> ()
        n294 = local write "Boast 2"(w114) -> ()
        n295 = local write "Boast 3"(w114) -> ()
        n296 = local write "Boast 4"(w114) -> ()
        n297 = local write "Boast 5"(w114) -> ()
        n298 = local write "Boast 6"(w114) -> ()
        n299 = local write "Boast 7"(w114) -> ()
        n300 = local write "Boast 8"(w114) -> ()
        n301 = local write "Boast 9"(w114) -> ()
        n302 = local write "Boast 10"(w114) -> ()
        n303 = local write "Boast 11"(w114) -> ()
        n304 = local write "Boast 12"(w114) -> ()
        n305 = local write "4 4"(w114) -> ()
        n306 = local write "4 3"(w114) -> ()
        n307 = local write "4 2"(w114) -> ()
        n308 = local write "4 1"(w114) -> ()
        n309 = local write "3 4"(w114) -> ()
        n310 = local write "3 3"(w114) -> ()
        n311 = local write "3 2"(w114) -> ()
        n312 = local write "3 1"(w114) -> ()
        n313 = local write "2 4"(w114) -> ()
        n314 = local write "2 3"(w114) -> ()
        n315 = local write "2 2"(w114) -> ()
        n316 = local write "2 1"(w114) -> ()
        n317 = local write "1 4"(w114) -> ()
        n318 = local write "1 3"(w114) -> ()
        n319 = local write "1 2"(w114) -> ()
        n320 = local write "1 1"(w114) -> ()
        n321 = local write "5 4"(w114) -> ()
        n322 = local write "5 3"(w114) -> ()
        n323 = local write "5 2"(w114) -> ()
        n324 = local write "5 1"(w114) -> ()
        n325 = local write "6 4"(w114) -> ()
        n326 = local write "6 3"(w114) -> ()
        n327 = local write "6 2"(w114) -> ()
        n328 = local write "6 1"(w114) -> ()
        n329 = local write "before n after"(0 ("before n after")) -> ()
        n330 = local write "S6"(w114) -> ()
        n331 = local write "S5"(w114) -> ()
        n332 = local write "S4"(w114) -> ()
        n333 = local write "S1"(w114) -> ()
        n334 = local write "S2"(w114) -> ()
        n335 = local write "S3"(w114) -> ()
        n336 = local write "Let"(w114) -> ()
        n337 = local write "Unexpected Winner2"(w114) -> ()
        n338 = local write "Unexpected Winner1"(w114) -> ()
        n339 = local write "Expected Winner2"(w114) -> ()
        n340 = local write "Expected Winner1"(w114) -> ()
        n341 = local write "Forced Error2"(w114) -> ()
        n342 = local write "Forced Error1"(w114) -> ()
        n343 = local write "Service2"(w114) -> ()
        n344 = local write "Service1"(w114) -> ()
        n345 = local write "Nolet2"(w114) -> ()
        n346 = local write "Nolet1"(w114) -> ()
        n347 = local write "Stroke2"(w114) -> ()
        n348 = local write "Stroke1"(w114) -> ()
        n349 = local write "Unforced Error2"(w114) -> ()
        n350 = local write "Unforced Error1"(w114) -> ()
        n351 = local write "Button 5"(w114) -> ()
        n352 = local write "Button 4"(w114) -> ()
        n353 = local write "Button 3"(w114) -> ()
        n354 = local write "Button 2"(w114) -> ()
        n355 = local write "Button 1"(w114) -> ()
        "Score change" <- bool[] [FALSE, FALSE] ("Score change")
        "Player1/Player2" <- bool[] [TRUE, FALSE] ("Score change")
      }
      frame #3 {
        w182 = T8 4 items=["Grayscale (U8)", "Grayscale (I16)", "Grayscale (SGL)", "Complex (CSG)", "RGB (U32)", "HSL (U32)", "RGB (U64)"] ("Image Type")
        n356 = call-poly <vilib>:"Read From Spreadsheet File.vi"("file path (dialog if empty)"=w196) -> ("all rows"=w199:i64[][])  [unwired: 6 in, 4 out]
        n357 = Path to Array of Strings(0:w180) -> (2:w193:string[])  [unwired: 1 out]
        n358 = call "IMAQ AVI Open"("AVI Path"=w180) -> ("error out"=w184:errorcluster, "Avi Refnum"=w183:T9)  [unwired: 9 in]
        n359 = Delete From Array(array=w199, length=4, index (row)=0) -> (array with subset deleted=w169:i64[][])  [unwired: 1 in, 1 out]
        n360 = Delete From Array(array=w193) -> (array with subset deleted=w194:string[])  [unwired: 2 in, 1 out]
        n361 = call "IMAQ AVI Get Info"("error in (no error)"=w184, "Avi Refnum"=w183) -> ("error out"=w186:errorcluster, "Number of Frames"=w189:u32, "Avi Refnum (duplicate)"=w179:T9, "Frame Data"=w185:T10)  [unwired: 5 in, 1 out]
        "Number of Frames" <- w189
        n362 = Array of Strings to Path(0:w194) -> (2:w195:path)  [unwired: 1 in]
        n363 = Index Array(array=w169, index (col)=0 ("disabled index (col)")) -> (element=w201:i64[])  [unwired: 1 in]
        n364 = Decrement(x=w189) -> (x-1=w192:u32)
        n365 = local write "Video to write"(w195) -> ()
        n366 = Array Max & Min(array=w201) -> (max value=w200:i64, max index (indices)=w168:i32)  [unwired: 2 out]
        n367 = Subtract(x=w192, y=200.0) -> (x-y=w190:dbl)
        n368 = Unbundle By Name(w185) -> ("framesPerSecond"=→"framesPerSecond":u32)
        n369 = property on="Progress..." class="Slide (strict)"(error in=w186, "Scale.Maximum"=w192) -> (error out=w187:errorcluster)  [unwired: 1 in, 1 out]
        n370 = Index Array(array=w169, index (row)=w168) -> (element=w167:i64[])  [unwired: 1 in]
        n371 = local write "Progress..."(w200) -> ()
        n372 = Index Array(array=w169, index (col) #1=57 ("disabled index (col)"), index (col) #2=58 ("index (col)")) -> (element #1=w173:i64[], element #2=w172:i64[])  [unwired: 2 in]
        n373 = for {
          N: w190 -> [_]
          tunnel: [w208] -> w176 mode=indexing
          i -> [w208]
        }
        "ful video frames" <- w176
        n374 = Reverse 1D Array(array=w167) -> (reversed array=w164:i64[])
        n375 = Add Array Elements(numeric array=w173) -> (sum=w171:i64)
        n376 = Add Array Elements(numeric array=w172) -> (sum=w170:i64)
        n377 = Array Subset(array=w164, index=0, length=5) -> (w163:i64[])
        n378 = local write "P1"(w171) -> ()
        n379 = local write "P2"(w170) -> ()
        n380 = Reverse 1D Array(array=w163) -> (reversed array=w162:i64[])
        n381 = Array Max & Min(array=w162) -> (max index (indices)=w161:i32)  [unwired: 3 out]
        n382 = call "IMAQ Create"("Image Name"="Video", "Image Type"=w182, "error in (no error)"=w187) -> ("New Image"=w178:T1, "error out"=w177:errorcluster)  [unwired: 2 in]
        n383 = case shown="4" w161 {
          tunnel: [w203 w204 w205 w206 w207] -> w160
          frame 0, Default {
            w203 = u16 0 items=["Game 1", "Game 2", "Game 3", "Game 4", "Game 5"] ("set")
          }
          frame 1 {
            w204 = u16 1 items=["Game 1", "Game 2", "Game 3", "Game 4", "Game 5"] ("set")
          }
          frame 2 {
            w205 = u16 2 items=["Game 1", "Game 2", "Game 3", "Game 4", "Game 5"] ("set")
          }
          frame 3 {
            w206 = u16 3 items=["Game 1", "Game 2", "Game 3", "Game 4", "Game 5"] ("set")
          }
          frame 4 {
            w207 = u16 4 items=["Game 1", "Game 2", "Game 3", "Game 4", "Game 5"] ("set")
          }
        }
        n384 = local write "set"(w160) -> ()
      }
    }
    n385 = while {
      tunnel: w9 -> [w355]
      tunnel: w8 -> [w354]
      tunnel: w2 -> [w353]
      shift-right: [w348] -> _
      shift-left: w7 -> [w347]
      tunnel: [w332] -> w5
      stop <- w333 continue-if-true
      # "This loop is the video play loop"
      # "1000/playback speed    / frames per sec"
      n386 = while {
        stop <- w375 continue-if-true
        n387 = local read "START"() -> (w374:bool)
        n388 = And(x=w374, y="Pause") -> (x .and. y?=w375:bool)
      }
      n389 = Index Array(array=w347, index="Progress...") -> (element=w335:i64)
      n390 = Array Max & Min(array=w347) -> (max value=w351:i64, max index (indices)=w352:i32)  [unwired: 2 out]
      n391 = Increment(x=w335) -> (x+1=w336:i64)
      n392 = property on="Progress..." class="Slide (strict)"("Scale.Maximum"=w352) -> ()  [unwired: 2 in, 2 out]
      n393 = Greater Or Equal?(x=w336, y=w351) -> (x >= y?=w339:bool)
      n394 = while {
        stop <- w364 stop-if-true
        n395 = local read "START"() -> (w361:bool)
        n396 = Not(x=w361) -> (.not. x?=w360:bool)
        n397 = Compound Arithmetic op=OR(w360, "Play", "Load video", "stop") -> (w364:bool)
        n398 = case shown="False" "stop" {
          frame False {
          }
          frame True {
            w366 = FALSE ("Play")
            n399 = local write "stop"(w366) -> ()
            n400 = local write "Play"(w366) -> ()
          }
        }
      }
      n401 = Select(t=w351, s=w339, f=w335) -> (s? t:f=w316:i64)
      "Video Frame" <- w316
      n402 = call "IMAQ AVI Read Frame"("error in (no error)"=w353, "Frame Number"=w316, "Image"=w354, "Avi Refnum"=w355) -> ("Image Out"=w349:T1, "Avi Refnum (duplicate)"=w332:T9)  [unwired: 4 in, 2 out]
      n403 = case shown="False" "Boolean" {
        tunnel: w349 -> [w357 w359]
        frame False {
          n404 = property on="Video 2" class="ImageControl"("Visible"=TRUE) -> ()  [unwired: 2 in, 2 out]
          "Video 2" <- w357
        }
        frame True {
          n405 = property on="Video 2" class="ImageControl"("Visible"=FALSE) -> ()  [unwired: 2 in, 2 out]
          "Video" <- w359
        }
      }
      n406 = Or(x="fast forward", y="fast rewind") -> (x .or. y?=w330:bool)
      n407 = Increment(x="Progress...") -> (x+1=w331:u32)
      n408 = Select(t=1.0, s=w330, f="playback speed") -> (s? t:f=w342:dbl)
      n409 = Increment(x=w331) -> (x+1=w334:u32)
      n410 = local read "framesPerSecond"() -> (w317:u32)
      n411 = Select(t=w334, s="fast forward", f=w331) -> (s? t:f=w326:u32)
      n412 = Subtract(x="Progress...", y=2) -> (x-y=w327:u32)
      n413 = Divide(x=1000.0, y=w342) -> (x/y=w346:dbl)
      n414 = Divide(x=w346, y=w317) -> (x/y=w344:dbl)
      n415 = Select(t=w327, s="fast rewind", f=w326) -> (s? t:f=w325:u32)
      n416 = Round Toward -Infinity(1:w344) -> (0:w343:dbl)
      "playback speed" <- w343
      n417 = Quotient & Remainder(x=w316, y=w317) -> (x-y*floor(x/y)=w320:i64, floor(x/y)=w318:i64)
      n418 = Wait (ms)(milliseconds to wait=w343) -> ()  [unwired: 1 out]
      n419 = local read "Load video"() -> (w337:bool)
      n420 = Divide(x=w320, y=w317) -> (x/y=w321:dbl)
      n421 = Quotient & Remainder(x=w318, y=60.0) -> (x-y*floor(x/y)=→"sec":dbl, floor(x/y)=→"Min":dbl)
      n422 = Select(t="Progress...", s=w339, f=w325) -> (s? t:f=w338:u32)
      n423 = Multiply(x=100.0, y=w321) -> (x*y=→"milsec":dbl)
      n424 = case shown="False" w337 {
        tunnel: w347 -> [w367 _]
        tunnel: w338 -> [w368 _]
        tunnel: [w368 w369] -> w350
        tunnel: [w367 w372] -> w348
        frame False {
        }
        frame True {
          n425 = local read "frames 2 play"() -> (w372:i64[])
          n426 = Array Max & Min(array=w372) -> (max index (indices)=w371:i32)  [unwired: 3 out]
          n427 = property on="Progress..." class="Slide (strict)"("Scale.Maximum"=w371) -> ()  [unwired: 2 in, 2 out]
          n428 = local write "Load video"(FALSE ("Play")) -> ()
          n429 = local read "Progress..."() -> (w369:u32)
        }
      }
      n430 = local write "Progress..."(w350) -> ()
      n431 = local read "START"() -> (w333:bool)
    }
    n432 = while {
      shift-right: [w376] -> _
      shift-left: T2."Display" ("Main tab") -> [w377]
      tunnel: w9 -> [w389]
      shift-right: [w379] -> _
      shift-left: w10 -> [w392]
      tunnel: w7 -> [_]
      tunnel: w2 -> [_]
      stop <- w378 continue-if-true
      w382 = T2."Coding" ("Main tab")
      # "Moving to display tab"
      n433 = case shown="\"Display\"" w377 {
        tunnel: w392 -> [w578 w1536 w1888 w1900 w2268 w2304 w2459]
        tunnel: [w404 w1536 w1888 w1900 w2268 w2304 w2442] -> w379
        tunnel: [T2."Edit video" ("Main tab") w1515 T6."Display" ("Main tab") T2."Display" ("Main tab") T2."Edit coding" ("Main tab") w2305 T2."Edit video" ("Main tab")] -> w384
        tunnel: w389 -> [w576 _ _ _ _ _ _]
        frame "Coding", Default {
          n434 = local read "Drop"() -> (w574:bool)
          n435 = local read "Drop 2"() -> (w573:bool)
          n436 = local read "Drop 3"() -> (w572:bool)
          n437 = local read "Drop 4"() -> (w571:bool)
          n438 = local read "Drop 5"() -> (w570:bool)
          n439 = local read "Drop 6"() -> (w569:bool)
          n440 = local read "Drop 7"() -> (w568:bool)
          n441 = local read "Drop 8"() -> (w567:bool)
          n442 = local read "Drop 9"() -> (w566:bool)
          n443 = local read "Drop 10"() -> (w565:bool)
          n444 = local read "Drop 11"() -> (w564:bool)
          n445 = local read "Drop 12"() -> (w563:bool)
          n446 = local read "Chop"() -> (w562:bool)
          n447 = local read "Chop 2"() -> (w561:bool)
          n448 = local read "Chop 3"() -> (w560:bool)
          n449 = local read "Chop 4"() -> (w559:bool)
          n450 = local read "Chop 5"() -> (w558:bool)
          n451 = local read "Chop 6"() -> (w557:bool)
          n452 = local read "Chop 7"() -> (w556:bool)
          n453 = local read "Chop 8"() -> (w555:bool)
          n454 = local read "Chop 9"() -> (w554:bool)
          n455 = local read "Chop 10"() -> (w553:bool)
          n456 = local read "Chop 11"() -> (w552:bool)
          n457 = local read "Chop 12"() -> (w551:bool)
          n458 = local read "Let"() -> (w550:bool)
          n459 = local read "Unexpected Winner2"() -> (w541:bool)
          n460 = local read "Unexpected Winner1"() -> (w540:bool)
          n461 = local read "Expected Winner2"() -> (w539:bool)
          n462 = local read "Expected Winner1"() -> (w538:bool)
          n463 = local read "Forced Error2"() -> (w544:bool)
          n464 = local read "Forced Error1"() -> (w542:bool)
          n465 = local read "Nolet2"() -> (w549:bool)
          n466 = local read "Nolet1"() -> (w548:bool)
          n467 = local read "Stroke2"() -> (w547:bool)
          n468 = local read "Stroke1"() -> (w546:bool)
          n469 = local read "Unforced Error2"() -> (w545:bool)
          n470 = local read "Unforced Error1"() -> (w543:bool)
          n471 = Build Array(w574, w573, w572, w571, w570, w569, w568, w567, w566, w565, w564, w563, w562, w561, w560, w559, w558, w557, w556, w555, w554, w553, w552, w551, w550, w549, w548, w547, w546, w545, w544, w543, w542, w541, w540, w539, w538) -> (w428:bool[])
          n472 = local read "lob 13"() -> (w537:bool)
          n473 = local read "lob 2"() -> (w536:bool)
          n474 = local read "lob 3"() -> (w535:bool)
          n475 = local read "lob 4"() -> (w534:bool)
          n476 = local read "lob 5"() -> (w533:bool)
          n477 = local read "lob 6"() -> (w532:bool)
          n478 = local read "lob 7"() -> (w531:bool)
          n479 = local read "lob 8"() -> (w530:bool)
          n480 = local read "lob 9"() -> (w529:bool)
          n481 = local read "lob 10"() -> (w528:bool)
          n482 = local read "lob 11"() -> (w527:bool)
          n483 = local read "lob 12"() -> (w526:bool)
          n484 = local read "Smash"() -> (w525:bool)
          n485 = local read "Smash 2"() -> (w524:bool)
          n486 = local read "Smash 3"() -> (w523:bool)
          n487 = local read "Smash 4"() -> (w522:bool)
          n488 = local read "Smash 5"() -> (w521:bool)
          n489 = local read "Smash 6"() -> (w520:bool)
          n490 = local read "Smash 7"() -> (w519:bool)
          n491 = local read "Smash 8"() -> (w518:bool)
          n492 = local read "Smash 9"() -> (w517:bool)
          n493 = local read "Smash 10"() -> (w516:bool)
          n494 = local read "Smash 11"() -> (w515:bool)
          n495 = local read "Smash 12"() -> (w514:bool)
          n496 = local read "Boast"() -> (w513:bool)
          n497 = local read "Boast 2"() -> (w512:bool)
          n498 = local read "Boast 3"() -> (w511:bool)
          n499 = local read "Boast 4"() -> (w510:bool)
          n500 = local read "Boast 5"() -> (w509:bool)
          n501 = local read "Boast 6"() -> (w508:bool)
          n502 = local read "Boast 7"() -> (w507:bool)
          n503 = local read "Boast 8"() -> (w506:bool)
          n504 = local read "Boast 9"() -> (w505:bool)
          n505 = local read "Boast 10"() -> (w504:bool)
          n506 = local read "Boast 11"() -> (w503:bool)
          n507 = local read "Boast 12"() -> (w502:bool)
          n508 = Build Array(w537, w536, w535, w534, w533, w532, w531, w530, w529, w528, w527, w526, w525, w524, w523, w522, w521, w520, w519, w518, w517, w516, w515, w514, w513, w512, w511, w510, w509, w508, w507, w506, w505, w504, w503, w502) -> (w427:bool[])
          n509 = local read "Player2"() -> (w420:bool)
          n510 = local read "Player1"() -> (w421:bool)
          n511 = local read "Pause"() -> (w422:bool)
          n512 = local read "ADrive"() -> (w501:bool)
          n513 = local read "ADrive 2"() -> (w500:bool)
          n514 = local read "ADrive 3"() -> (w499:bool)
          n515 = local read "ADrive 4"() -> (w498:bool)
          n516 = local read "ADrive 5"() -> (w497:bool)
          n517 = local read "ADrive 6"() -> (w496:bool)
          n518 = local read "ADrive 7"() -> (w495:bool)
          n519 = local read "ADrive 8"() -> (w494:bool)
          n520 = local read "ADrive 9"() -> (w493:bool)
          n521 = local read "ADrive 10"() -> (w492:bool)
          n522 = local read "ADrive 11"() -> (w491:bool)
          n523 = local read "ADrive 12"() -> (w490:bool)
          n524 = local read "SWADrive"() -> (w489:bool)
          n525 = local read "SWADrive 2"() -> (w488:bool)
          n526 = local read "SWADrive 3"() -> (w487:bool)
          n527 = local read "SWADrive 4"() -> (w486:bool)
          n528 = local read "SWADrive 5"() -> (w485:bool)
          n529 = local read "SWADrive 6"() -> (w484:bool)
          n530 = local read "SWADrive 7"() -> (w483:bool)
          n531 = local read "SWADrive 8"() -> (w482:bool)
          n532 = local read "SWADrive 9"() -> (w481:bool)
          n533 = local read "SWADrive 10"() -> (w480:bool)
          n534 = local read "SWADrive 11"() -> (w479:bool)
          n535 = local read "SWADrive 12"() -> (w478:bool)
          n536 = local read "S6"() -> (w475:bool)
          n537 = local read "S5"() -> (w474:bool)
          n538 = local read "S4"() -> (w473:bool)
          n539 = local read "S1"() -> (w472:bool)
          n540 = local read "S2"() -> (w471:bool)
          n541 = local read "S3"() -> (w470:bool)
          n542 = local read "Service2"() -> (w477:bool)
          n543 = local read "Service1"() -> (w476:bool)
          n544 = Build Array(w501, w500, w499, w498, w497, w496, w495, w494, w493, w492, w491, w490, w489, w488, w487, w486, w485, w484, w483, w482, w481, w480, w479, w478, w477, w476, w475, w474, w473, w472, w471, w470, w422, w421, w420) -> (w426:bool[])
          n545 = local read "DDrive"() -> (w469:bool)
          n546 = local read "DDrive 2"() -> (w468:bool)
          n547 = local read "DDrive 3"() -> (w467:bool)
          n548 = local read "DDrive 4"() -> (w466:bool)
          n549 = local read "DDrive 5"() -> (w465:bool)
          n550 = local read "DDrive 6"() -> (w464:bool)
          n551 = local read "DDrive 7"() -> (w463:bool)
          n552 = local read "DDrive 8"() -> (w462:bool)
          n553 = local read "DDrive 9"() -> (w461:bool)
          n554 = local read "DDrive 10"() -> (w460:bool)
          n555 = local read "DDrive 11"() -> (w459:bool)
          n556 = local read "DDrive 12"() -> (w458:bool)
          n557 = local read "SWDDrive"() -> (w457:bool)
          n558 = local read "SWDDrive 2"() -> (w456:bool)
          n559 = local read "SWDDrive 3"() -> (w455:bool)
          n560 = local read "SWDDrive 4"() -> (w454:bool)
          n561 = local read "SWDDrive 5"() -> (w453:bool)
          n562 = local read "SWDDrive 6"() -> (w452:bool)
          n563 = local read "SWDDrive 7"() -> (w451:bool)
          n564 = local read "SWDDrive 8"() -> (w450:bool)
          n565 = local read "SWDDrive 9"() -> (w449:bool)
          n566 = local read "SWDDrive 10"() -> (w448:bool)
          n567 = local read "SWDDrive 11"() -> (w447:bool)
          n568 = local read "SWDDrive 12"() -> (w446:bool)
          n569 = local read "Button 5"() -> (w419:bool)
          n570 = local read "Button 4"() -> (w418:bool)
          n571 = local read "Button 3"() -> (w417:bool)
          n572 = local read "Button 2"() -> (w416:bool)
          n573 = local read "Button 1"() -> (w415:bool)
          n574 = Build Array(w469, w468, w467, w466, w465, w464, w463, w462, w461, w460, w459, w458, w457, w456, w455, w454, w453, w452, w451, w450, w449, w448, w447, w446) -> (w424:bool[])
          n575 = local read "4 4"() -> (w438:bool)
          n576 = local read "4 3"() -> (w439:bool)
          n577 = local read "4 2"() -> (w440:bool)
          n578 = local read "4 1"() -> (w441:bool)
          n579 = local read "3 4"() -> (w442:bool)
          n580 = local read "3 3"() -> (w443:bool)
          n581 = local read "3 2"() -> (w444:bool)
          n582 = local read "3 1"() -> (w445:bool)
          n583 = local read "2 4"() -> (w437:bool)
          n584 = local read "2 3"() -> (w436:bool)
          n585 = local read "2 2"() -> (w435:bool)
          n586 = local read "2 1"() -> (w434:bool)
          n587 = local read "1 4"() -> (w433:bool)
          n588 = local read "1 3"() -> (w432:bool)
          n589 = local read "1 2"() -> (w431:bool)
          n590 = local read "1 1"() -> (w430:bool)
          n591 = local read "5 4"() -> (w413:bool)
          n592 = local read "5 3"() -> (w412:bool)
          n593 = local read "5 2"() -> (w411:bool)
          n594 = local read "5 1"() -> (w410:bool)
          n595 = local read "6 4"() -> (w409:bool)
          n596 = local read "6 3"() -> (w408:bool)
          n597 = local read "6 2"() -> (w407:bool)
          n598 = local read "6 1"() -> (w406:bool)
          n599 = local read "Undo"() -> (w405:bool)
          n600 = Build Array(w419, w418, w417, w416, w415, w405) -> (w414:bool[])
          n601 = Build Array(w438, w439, w440, w441, w442, w443, w444, w445, w437, w436, w435, w434, w433, w432, w431, w430, w413, w412, w411, w410, w409, w408, w407, w406) -> (w425:bool[])
          n602 = local read "Video Frame"() -> (w575:u32)
          n603 = Build Array(w414, w424, w425, w426, w427, w428) -> (w429:bool[][])
          n604 = Or Array Elements(Boolean array=w429) -> (logical OR=w423:bool)
          n605 = case shown="True" w423 {
            tunnel: w575 -> [_ w758]
            tunnel: w578 -> [w579 w759]
            tunnel: [w579 w616] -> w404
            tunnel: w576 -> [_ w755]
            frame False {
            }
            frame True {
              w614 = "\r"
              w633 = 0 ("index")
              w586 = "\t"
              # "extra code buttons\n\nundo button / error button\n\nlink all (extra buttons) to linkshots logic"
              n606 = stacked-sequence {
                tunnel: w759 -> [w783 _ _ _ _ _ _ _ _ _ _ _ _ _ w1480 _]
                tunnel: [w783 _ _ _ _ _ _ _ _ _ _ _ _ _ _ _] -> w637
                tunnel: w758 -> [w789 _ _ _ _ _ _ _ _ _ _ _ _ _ _ _]
                tunnel: [w789 _ _ _ _ _ _ _ _ _ _ _ _ _ _ _] -> w640
                tunnel: w755 -> [w788 _ _ _ _ _ _ _ _ _ _ _ _ _ _ _]
                tunnel: [w785 _ _ _ _ _ _ _ _ _ _ _ _ _ _ _] -> w754
                tunnel: [_ _ "before 2" _ _ _ _ _ _ _ _ _ _ _ _ _] -> w753
                tunnel: [_ _ "after 2" _ _ _ _ _ _ _ _ _ _ _ _ _] -> w752
                tunnel: [_ _ w870 _ _ _ _ _ _ _ _ _ _ _ _ _] -> w751
                tunnel: [_ _ w869 _ _ _ _ _ _ _ _ _ _ _ _ _] -> w750
                tunnel: [_ _ w868 _ _ _ _ _ _ _ _ _ _ _ _ _] -> w749
                tunnel: [_ _ w867 _ _ _ _ _ _ _ _ _ _ _ _ _] -> w748
                tunnel: [_ _ w866 _ _ _ _ _ _ _ _ _ _ _ _ _] -> w747
                tunnel: [_ _ w865 _ _ _ _ _ _ _ _ _ _ _ _ _] -> w746
                tunnel: [_ _ w864 _ _ _ _ _ _ _ _ _ _ _ _ _] -> w745
                tunnel: [_ _ w863 _ _ _ _ _ _ _ _ _ _ _ _ _] -> w744
                tunnel: [_ _ w862 _ _ _ _ _ _ _ _ _ _ _ _ _] -> w743
                tunnel: [_ _ w861 _ _ _ _ _ _ _ _ _ _ _ _ _] -> w742
                tunnel: [_ _ w860 _ _ _ _ _ _ _ _ _ _ _ _ _] -> w741
                tunnel: [_ _ w859 _ _ _ _ _ _ _ _ _ _ _ _ _] -> w740
                tunnel: [_ _ w858 _ _ _ _ _ _ _ _ _ _ _ _ _] -> w739
                tunnel: [_ _ w857 _ _ _ _ _ _ _ _ _ _ _ _ _] -> w738
                tunnel: [_ _ w856 _ _ _ _ _ _ _ _ _ _ _ _ _] -> w737
                tunnel: [_ _ w855 _ _ _ _ _ _ _ _ _ _ _ _ _] -> w736
                tunnel: [_ _ w854 _ _ _ _ _ _ _ _ _ _ _ _ _] -> w735
                tunnel: [_ _ w853 _ _ _ _ _ _ _ _ _ _ _ _ _] -> w734
                tunnel: [_ _ w852 _ _ _ _ _ _ _ _ _ _ _ _ _] -> w733
                tunnel: [_ _ w851 _ _ _ _ _ _ _ _ _ _ _ _ _] -> w732
                tunnel: [_ _ w850 _ _ _ _ _ _ _ _ _ _ _ _ _] -> w731
                tunnel: [_ _ w849 _ _ _ _ _ _ _ _ _ _ _ _ _] -> w730
                tunnel: [_ _ w848 _ _ _ _ _ _ _ _ _ _ _ _ _] -> w729
                tunnel: [_ _ w847 _ _ _ _ _ _ _ _ _ _ _ _ _] -> w728
                tunnel: [_ _ _ w918 _ _ _ _ _ _ _ _ _ _ _ _] -> w727
                tunnel: [_ _ _ w917 _ _ _ _ _ _ _ _ _ _ _ _] -> w726
                tunnel: [_ _ _ w916 _ _ _ _ _ _ _ _ _ _ _ _] -> w725
                tunnel: [_ _ _ w915 _ _ _ _ _ _ _ _ _ _ _ _] -> w724
                tunnel: [_ _ _ _ w998 _ _ _ _ _ _ _ _ _ _ _] -> w723
                tunnel: [_ _ _ _ w997 _ _ _ _ _ _ _ _ _ _ _] -> w722
                tunnel: [_ _ _ _ w996 _ _ _ _ _ _ _ _ _ _ _] -> w721
                tunnel: [_ _ _ _ _ w1040 _ _ _ _ _ _ _ _ _ _] -> w720
                tunnel: [_ _ _ _ _ w1039 _ _ _ _ _ _ _ _ _ _] -> w719
                tunnel: [_ _ _ _ _ w1038 _ _ _ _ _ _ _ _ _ _] -> w718
                tunnel: [_ _ _ _ _ _ w1068 _ _ _ _ _ _ _ _ _] -> w717
                tunnel: [_ _ _ _ _ _ _ w1126 _ _ _ _ _ _ _ _] -> w716
                tunnel: [_ _ _ _ _ _ _ _ w1184 _ _ _ _ _ _ _] -> w715
                tunnel: [_ _ _ _ _ _ _ _ _ w1236 _ _ _ _ _ _] -> w714
                tunnel: [_ _ _ _ _ _ _ _ _ _ w1300 _ _ _ _ _] -> w713
                tunnel: [_ _ _ _ _ _ _ _ _ _ _ w1340 _ _ _ _] -> w712
                tunnel: [_ _ _ _ _ _ _ _ _ _ _ _ w1380 _ _ _] -> w711
                tunnel: [_ _ _ _ _ _ _ _ _ _ _ _ _ _ w1443 _] -> w710
                tunnel: [_ _ _ _ _ _ _ _ _ _ _ _ _ _ w1444 _] -> w709
                tunnel: [_ _ _ _ _ _ _ _ _ _ _ _ _ _ w1445 _] -> w708
                tunnel: [_ _ _ _ _ _ _ _ _ _ _ _ _ _ w1450 _] -> w707
                tunnel: [_ _ _ _ _ _ _ _ _ _ _ _ _ _ w1451 _] -> w706
                tunnel: [_ _ _ _ _ _ _ _ _ _ _ _ _ _ w1452 _] -> w705
                tunnel: [_ _ _ _ _ _ _ _ _ _ _ _ _ _ w1453 _] -> w704
                tunnel: [_ _ _ _ _ _ _ _ _ _ _ _ _ _ w1454 _] -> w703
                tunnel: [_ _ _ _ _ _ _ _ _ _ _ _ _ _ w1455 _] -> w702
                tunnel: [_ _ _ _ _ _ _ _ _ _ _ _ _ _ w1456 _] -> w701
                tunnel: [_ _ _ _ _ _ _ _ _ _ _ _ _ _ w1457 _] -> w700
                tunnel: [_ _ _ _ _ _ _ _ _ _ _ _ _ _ w1458 _] -> w699
                tunnel: [_ _ _ _ _ _ _ _ _ _ _ _ _ _ w1458 _] -> w698
                tunnel: [_ _ _ _ _ _ _ _ _ _ _ _ _ _ w1446 _] -> w697
                tunnel: [_ _ _ _ _ _ _ _ _ _ _ _ _ _ w1447 _] -> w696
                tunnel: [_ _ _ _ _ _ _ _ _ _ _ _ _ _ w1448 _] -> w695
                tunnel: [_ _ _ _ _ _ _ _ _ _ _ _ _ _ w1449 _] -> w694
                tunnel: [_ _ _ _ _ _ _ _ _ _ _ _ _ _ _ w1499] -> w669
                tunnel: [_ _ _ _ _ _ _ _ _ _ _ _ _ w1429 _ _] -> w664
                tunnel: [_ _ _ _ _ _ _ _ _ _ _ _ _ w1428 _ _] -> w663
                tunnel: [_ _ _ _ _ _ _ _ _ _ _ _ _ w1427 _ _] -> w662
                tunnel: [_ _ _ _ _ _ _ _ _ _ _ _ _ w1426 _ _] -> w661
                tunnel: [_ _ _ _ _ _ _ _ _ _ _ _ _ w1425 _ _] -> w660
                tunnel: [_ _ w834 _ _ _ _ _ _ _ _ _ _ _ _ _] -> w652
                tunnel: [_ _ _ _ _ _ _ _ _ _ _ _ _ w1424 _ _] -> w651
                tunnel: [_ _ _ _ _ _ _ _ _ _ _ _ _ w1423 _ _] -> w650
                tunnel: [_ _ _ _ _ _ _ _ _ _ _ _ _ w1422 _ _] -> w649
                tunnel: [_ _ _ _ _ _ _ _ _ _ _ _ _ w1421 _ _] -> w648
                tunnel: [_ _ _ _ _ _ _ _ _ _ _ _ _ w1420 _ _] -> w647
                tunnel: [_ _ w838 _ _ _ _ _ _ _ _ _ _ _ _ _] -> w646
                tunnel: [_ _ w837 _ _ _ _ _ _ _ _ _ _ _ _ _] -> w645
                tunnel: [_ _ w836 _ _ _ _ _ _ _ _ _ _ _ _ _] -> w644
                tunnel: [_ _ w835 _ _ _ _ _ _ _ _ _ _ _ _ _] -> w643
                tunnel: [_ _ _ w913 _ _ _ _ _ _ _ _ _ _ _ _] -> w584
                tunnel: [_ _ _ w912 _ _ _ _ _ _ _ _ _ _ _ _] -> w583
                tunnel: [_ _ _ w911 _ _ _ _ _ _ _ _ _ _ _ _] -> w582
                tunnel: [_ _ _ w910 _ _ _ _ _ _ _ _ _ _ _ _] -> w581
                tunnel: [_ _ _ w909 _ _ _ _ _ _ _ _ _ _ _ _] -> w580
                frame #0 {
                  n607 = local read "Pause"() -> (w784:bool)
                  n608 = And(x=w784, y="Pause lag on") -> (x .and. y?=w787:bool)
                  n609 = case shown="False" w784 {
                    frame False {
                      n610 = Tick Count (ms)() -> (millisecond timer value=w790:u32)
                      n611 = while {
                        tunnel: w790 -> [w802]
                        i -> [w793]
                        stop <- w800 stop-if-true
                        w796 = u32 25 ("milliseconds to wait")
                        n612 = Tick Count (ms)() -> (millisecond timer value=w803:u32)
                        n613 = Subtract(x=w803, y=w802) -> (x-y=w801:u32)
                        n614 = Multiply(x="Code lag(s)", y=1000) -> (x*y=w797:dbl)
                        n615 = Greater Or Equal?(x=w801, y=w797) -> (x >= y?=w800:bool)
                        n616 = Divide(x=w797, y=w796) -> (x/y=w795:dbl)
                        n617 = Divide(x=300.0, y=w795) -> (x/y=w792:dbl)
                        n618 = Multiply(x=w793, y=w792) -> (x*y=→"task":dbl)
                        n619 = Wait (ms)(milliseconds to wait=w796) -> ()  [unwired: 1 out]
                      }
                    }
                    frame True {
                    }
                  }
                  n620 = case shown="True" w787 {
                    tunnel: w789 -> [_ w807]
                    tunnel: w788 -> [_ w809]
                    tunnel: ["pauselag" ("Image Name") w805] -> w785
                    frame False {
                    }
                    frame True {
                      w810 = T8 4 items=["Grayscale (U8)", "Grayscale (I16)", "Grayscale (SGL)", "Complex (CSG)", "RGB (U32)", "HSL (U32)", "RGB (U64)"] ("Image Type")
                      n621 = local read "framesPerSecond"() -> (w816:u32)
                      n622 = local read "Number of Frames"() -> (w806:u32)
                      n623 = Increment(x=w807) -> (x+1=w808:u32)
                      n624 = Multiply(x="Pause lag(s)", y=w816) -> (x*y=w814:dbl)
                      n625 = call "IMAQ Create"("Image Name"="pauselag", "Image Type"=w810) -> ("New Image"=w805:T1, "error out"=w811:errorcluster)  [unwired: 3 in]
                      n626 = Round Toward +Infinity(x=w814) -> (ceil(x): smallest int >= x=w813:dbl)
                      n627 = for {
                        N: w813 -> [_]
                        tunnel: w808 -> [w823]
                        tunnel: w811 -> [w826]
                        tunnel: w805 -> [w825]
                        tunnel: w809 -> [w822]
                        tunnel: w806 -> [w820]
                        i -> [w824]
                        n628 = Add(x=w824, y=w823) -> (x+y=w819:u32)
                        n629 = local read "playback speed"() -> (w817:dbl)
                        n630 = Less Or Equal?(x=w820, y=w819) -> (x <= y?=w821:bool)
                        n631 = Select(t=w820, s=w821, f=w819) -> (s? t:f=w818:u32)
                        n632 = call "IMAQ AVI Read Frame"("error in (no error)"=w826, "Frame Number"=w818, "Image"=w825, "Avi Refnum"=w822) -> ("Image Out"=w827:T1)  [unwired: 4 in, 3 out]
                        n633 = local write "Video"(w827) -> ()
                        n634 = Wait (ms)(milliseconds to wait=w817) -> ()  [unwired: 1 out]
                      }
                    }
                  }
                }
                frame #1 {
                  w828 = i16 0 ("Service")
                  n635 = while {
                    stop <- w829 continue-if-true
                    n636 = local read "START"() -> (w830:bool)
                    n637 = local read "Pause"() -> (w831:bool)
                    n638 = And(x=w830, y=w831) -> (x .and. y?=w829:bool)
                  }
                  n639 = local write "Service"(w828) -> ()
                  n640 = local write "Cross"(w828) -> ()
                  n641 = local write "Straight"(w828) -> ()
                  n642 = local write "position"(w828) -> ()
                  n643 = local write "Player 1/2"(w828) -> ()
                  n644 = local write "Extra"(w828) -> ()
                }
                frame #2 {
                  n645 = local read "Service1"() -> (w878:bool)
                  n646 = local read "Service2"() -> (w880:bool)
                  n647 = Compound Arithmetic op=OR(w878, "Player1", w880, "Player2") -> (w877:bool)
                  n648 = Or(x="Player1", y="Player2") -> (x .or. y?=w883:bool)
                  n649 = case shown="True" w877 {
                    tunnel: w878 -> [_ w906]
                    tunnel: w880 -> [_ w905]
                    tunnel: "Player1" -> [_ w904]
                    tunnel: "Player2" -> [_ w903]
                    frame False {
                    }
                    frame True {
                      n650 = Or(x=w906, y=w904) -> (x .or. y?=w908:bool)
                      n651 = Or(x=w905, y=w903) -> (x .or. y?=w907:bool)
                      n652 = Build Array(w908, w907) -> (w902:bool[])
                      n653 = local write "Player1/Player2"(w902) -> ()
                    }
                  }
                  n654 = Boolean To (0,1)(Boolean=w883) -> (0, 1=→"Player 1/2":i16)
                  n655 = Boolean To (0,1)(Boolean="1 1") -> (0, 1=w870:i16)
                  n656 = Boolean To (0,1)(Boolean="1 2") -> (0, 1=w869:i16)
                  n657 = Boolean To (0,1)(Boolean="1 3") -> (0, 1=w868:i16)
                  n658 = Boolean To (0,1)(Boolean="1 4") -> (0, 1=w867:i16)
                  n659 = Boolean To (0,1)(Boolean="2 1") -> (0, 1=w866:i16)
                  n660 = Boolean To (0,1)(Boolean="2 2") -> (0, 1=w865:i16)
                  n661 = Boolean To (0,1)(Boolean="2 3") -> (0, 1=w864:i16)
                  n662 = Boolean To (0,1)(Boolean="2 4") -> (0, 1=w863:i16)
                  n663 = Boolean To (0,1)(Boolean="3 1") -> (0, 1=w862:i16)
                  n664 = Boolean To (0,1)(Boolean="3 2") -> (0, 1=w861:i16)
                  n665 = Boolean To (0,1)(Boolean="3 3") -> (0, 1=w860:i16)
                  n666 = Boolean To (0,1)(Boolean="3 4") -> (0, 1=w859:i16)
                  n667 = Boolean To (0,1)(Boolean="4 1") -> (0, 1=w858:i16)
                  n668 = Boolean To (0,1)(Boolean="4 2") -> (0, 1=w857:i16)
                  n669 = Boolean To (0,1)(Boolean="4 3") -> (0, 1=w856:i16)
                  n670 = Boolean To (0,1)(Boolean="4 4") -> (0, 1=w855:i16)
                  n671 = Boolean To (0,1)(Boolean="5 1") -> (0, 1=w854:i16)
                  n672 = Boolean To (0,1)(Boolean="5 2") -> (0, 1=w853:i16)
                  n673 = Boolean To (0,1)(Boolean="5 3") -> (0, 1=w852:i16)
                  n674 = Boolean To (0,1)(Boolean="5 4") -> (0, 1=w851:i16)
                  n675 = Boolean To (0,1)(Boolean="6 1") -> (0, 1=w850:i16)
                  n676 = Boolean To (0,1)(Boolean="6 2") -> (0, 1=w849:i16)
                  n677 = Boolean To (0,1)(Boolean="6 3") -> (0, 1=w848:i16)
                  n678 = Boolean To (0,1)(Boolean="6 4") -> (0, 1=w847:i16)
                  n679 = Compound Arithmetic op=OR("1 1", "1 2", "1 3", "1 4", "2 1", "2 2", "2 3", "2 4", "3 1", "3 2", "3 3", "3 4", "4 1", "4 2", "4 3", "4 4", "5 1", "5 2", "5 3", "5 4", "6 1", "6 2", "6 3", "6 4") -> (w901:bool)
                  n680 = Boolean To (0,1)(Boolean=w901) -> (0, 1=→"position":i16)
                  n681 = Boolean To (0,1)(Boolean="Button 1") -> (0, 1=w838:i16)
                  n682 = Boolean To (0,1)(Boolean="Button 2") -> (0, 1=w837:i16)
                  n683 = Boolean To (0,1)(Boolean="Button 3") -> (0, 1=w836:i16)
                  n684 = Boolean To (0,1)(Boolean="Button 4") -> (0, 1=w835:i16)
                  n685 = Boolean To (0,1)(Boolean="Button 5") -> (0, 1=w834:i16)
                  n686 = Compound Arithmetic op=OR(w838, w837, w836, w835, w834) -> (→"Extra":i16)
                }
                frame #3 {
                  n687 = Compound Arithmetic op=OR("ADrive", "ADrive 2", "ADrive 3", "ADrive 4", "ADrive 5", "ADrive 6", "ADrive 7", "ADrive 8", "ADrive 9", "ADrive 10", "ADrive 11", "ADrive 12") -> (w970:bool)
                  n688 = Compound Arithmetic op=OR("SWADrive", "SWADrive 2", "SWADrive 3", "SWADrive 4", "SWADrive 5", "SWADrive 6", "SWADrive 7", "SWADrive 8", "SWADrive 9", "SWADrive 10", "SWADrive 11", "SWADrive 12") -> (w931:bool)
                  n689 = Boolean To (0,1)(Boolean=w970) -> (0, 1=w918:i16)
                  n690 = Boolean To (0,1)(Boolean=w931) -> (0, 1=w916:i16)
                  n691 = Compound Arithmetic op=OR("DDrive", "DDrive 2", "DDrive 3", "DDrive 4", "DDrive 5", "DDrive 6", "DDrive 7", "DDrive 8", "DDrive 9", "DDrive 10", "DDrive 11", "DDrive 12") -> (w957:bool)
                  n692 = Compound Arithmetic op=OR("SWDDrive", "SWDDrive 2", "SWDDrive 3", "SWDDrive 4", "SWDDrive 5", "SWDDrive 6", "SWDDrive 7", "SWDDrive 8", "SWDDrive 9", "SWDDrive 10", "SWDDrive 11", "SWDDrive 12") -> (w944:bool)
                  n693 = Boolean To (0,1)(Boolean=w957) -> (0, 1=w917:i16)
                  n694 = Boolean To (0,1)(Boolean=w944) -> (0, 1=w915:i16)
                  n695 = case shown="4" "set" {
                    tunnel: [i16 1 ("Service") i16 0 ("Service") i16 0 ("Service") i16 0 ("Service") i16 0 ("Service")] -> w913
                    tunnel: [i16 0 ("Service") i16 1 ("Service") i16 0 ("Service") i16 0 ("Service") i16 0 ("Service")] -> w912
                    tunnel: [i16 0 ("Service") i16 0 ("Service") i16 1 ("Service") i16 0 ("Service") i16 0 ("Service")] -> w911
                    tunnel: [i16 0 ("Service") i16 0 ("Service") i16 0 ("Service") i16 1 ("Service") i16 0 ("Service")] -> w910
                    tunnel: [i16 0 ("Service") i16 0 ("Service") i16 0 ("Service") i16 0 ("Service") i16 1 ("Service")] -> w909
                    frame 0, Default {
                    }
                    frame 1 {
                    }
                    frame 2 {
                    }
                    frame 3 {
                    }
                    frame 4 {
                    }
                  }
                }
                frame #4 {
                  n696 = Compound Arithmetic op=OR("Chop", "Chop 2", "Chop 3", "Chop 4", "Chop 5", "Chop 6", "Chop 7", "Chop 8", "Chop 9", "Chop 10", "Chop 11", "Chop 12") -> (w1035:bool)
                  n697 = Boolean To (0,1)(Boolean=w1035) -> (0, 1=w997:i16)
                  n698 = Compound Arithmetic op=OR("lob 13", "lob 2", "lob 3", "lob 4", "lob 5", "lob 6", "lob 7", "lob 8", "lob 9", "lob 10", "lob 11", "lob 12") -> (w1036:bool)
                  n699 = Compound Arithmetic op=OR("Drop", "Drop 2", "Drop 3", "Drop 4", "Drop 5", "Drop 6", "Drop 7", "Drop 8", "Drop 9", "Drop 10", "Drop 11", "Drop 12") -> (w1037:bool)
                  n700 = Boolean To (0,1)(Boolean=w1037) -> (0, 1=w998:i16)
                  n701 = Boolean To (0,1)(Boolean=w1036) -> (0, 1=w996:i16)
                }
                frame #5 {
                  n702 = Compound Arithmetic op=OR("Boast 2", "Boast 4", "Boast 6", "Boast 8", "Boast 10", "Boast 12") -> (w1059:bool)
                  n703 = Boolean To (0,1)(Boolean=w1059) -> (0, 1=w1039:i16)
                  n704 = Compound Arithmetic op=OR("Smash", "Smash 2", "Smash 3", "Smash 4", "Smash 5", "Smash 6", "Smash 7", "Smash 8", "Smash 9", "Smash 10", "Smash 11", "Smash 12") -> (w1066:bool)
                  n705 = Compound Arithmetic op=OR("Boast", "Boast 3", "Boast 5", "Boast 7", "Boast 9", "Boast 11") -> (w1067:bool)
                  n706 = Boolean To (0,1)(Boolean=w1067) -> (0, 1=w1040:i16)
                  n707 = Boolean To (0,1)(Boolean=w1066) -> (0, 1=w1038:i16)
                }
                frame #6 {
                  # "forehand"
                  n708 = local read "Smash 10"() -> (w1102:bool)
                  n709 = local read "Chop 10"() -> (w1114:bool)
                  n710 = local read "Smash 2"() -> (w1106:bool)
                  n711 = local read "Smash 5"() -> (w1105:bool)
                  n712 = local read "Smash 6"() -> (w1104:bool)
                  n713 = local read "Smash 9"() -> (w1103:bool)
                  n714 = local read "Boast 10"() -> (w1096:bool)
                  n715 = local read "Drop 10"() -> (w1120:bool)
                  n716 = local read "Chop 2"() -> (w1118:bool)
                  n717 = local read "Chop 5"() -> (w1117:bool)
                  n718 = local read "Chop 6"() -> (w1116:bool)
                  n719 = local read "Chop 9"() -> (w1115:bool)
                  n720 = local read "Boast 2"() -> (w1100:bool)
                  n721 = local read "Boast 5"() -> (w1099:bool)
                  n722 = local read "Boast 6"() -> (w1098:bool)
                  n723 = local read "Boast 9"() -> (w1097:bool)
                  n724 = local read "Drop 2"() -> (w1124:bool)
                  n725 = local read "Drop 5"() -> (w1123:bool)
                  n726 = local read "Drop 6"() -> (w1122:bool)
                  n727 = local read "Drop 9"() -> (w1121:bool)
                  n728 = local read "Smash"() -> (w1107:bool)
                  n729 = local read "lob 10"() -> (w1108:bool)
                  n730 = local read "Chop"() -> (w1119:bool)
                  n731 = local read "Boast"() -> (w1101:bool)
                  n732 = local read "Drop"() -> (w1125:bool)
                  n733 = local read "lob 2"() -> (w1112:bool)
                  n734 = local read "lob 5"() -> (w1111:bool)
                  n735 = local read "lob 6"() -> (w1110:bool)
                  n736 = local read "lob 9"() -> (w1109:bool)
                  n737 = local read "lob 13"() -> (w1113:bool)
                  n738 = Compound Arithmetic op=OR(w1125, w1124, w1123, w1122, w1121, w1120, w1119, w1118, w1117, w1116, w1115, w1114, w1113, w1112, w1111, w1110, w1109, w1108, w1107, w1106, w1105, w1104, w1103, w1102, w1101, w1100, w1099, w1098, w1097, w1096) -> (w1069:bool)
                  n739 = local read "SWADrive 10"() -> (w1089:bool)
                  n740 = local read "SWDDrive 10"() -> (w1095:bool)
                  n741 = local read "SWADrive 2"() -> (w1085:bool)
                  n742 = local read "SWADrive 5"() -> (w1086:bool)
                  n743 = local read "SWADrive 6"() -> (w1087:bool)
                  n744 = local read "SWADrive 9"() -> (w1088:bool)
                  n745 = local read "SWDDrive 2"() -> (w1091:bool)
                  n746 = local read "SWDDrive 5"() -> (w1092:bool)
                  n747 = local read "SWDDrive 6"() -> (w1093:bool)
                  n748 = local read "SWDDrive 9"() -> (w1094:bool)
                  n749 = local read "SWADrive"() -> (w1084:bool)
                  n750 = local read "SWDDrive"() -> (w1090:bool)
                  n751 = local read "ADrive 10"() -> (w1077:bool)
                  n752 = local read "DDrive 10"() -> (w1083:bool)
                  n753 = local read "ADrive 2"() -> (w1073:bool)
                  n754 = local read "ADrive 5"() -> (w1074:bool)
                  n755 = local read "ADrive 6"() -> (w1075:bool)
                  n756 = local read "ADrive 9"() -> (w1076:bool)
                  n757 = local read "DDrive 2"() -> (w1079:bool)
                  n758 = local read "DDrive 5"() -> (w1080:bool)
                  n759 = local read "DDrive 6"() -> (w1081:bool)
                  n760 = local read "DDrive 9"() -> (w1082:bool)
                  n761 = local read "ADrive"() -> (w1072:bool)
                  n762 = local read "DDrive"() -> (w1078:bool)
                  n763 = Compound Arithmetic op=OR(w1072, w1073, w1074, w1075, w1076, w1077, w1078, w1079, w1080, w1081, w1082, w1083, w1084, w1085, w1086, w1087, w1088, w1089, w1090, w1091, w1092, w1093, w1094, w1095) -> (w1070:bool)
                  n764 = Or(x=w1069, y=w1070) -> (x .or. y?=w1071:bool)
                  n765 = Boolean To (0,1)(Boolean=w1071) -> (0, 1=w1068:i16)
                }
                frame #7 {
                  # "backhand"
                  n766 = local read "Smash 11"() -> (w1158:bool)
                  n767 = local read "Smash 12"() -> (w1157:bool)
                  n768 = local read "Chop 11"() -> (w1170:bool)
                  n769 = local read "Chop 12"() -> (w1169:bool)
                  n770 = local read "Smash 3"() -> (w1162:bool)
                  n771 = local read "Smash 4"() -> (w1161:bool)
                  n772 = local read "Smash 7"() -> (w1160:bool)
                  n773 = local read "Smash 8"() -> (w1159:bool)
                  n774 = local read "Boast 11"() -> (w1152:bool)
                  n775 = local read "Boast 12"() -> (w1151:bool)
                  n776 = local read "Drop 11"() -> (w1176:bool)
                  n777 = local read "Drop 12"() -> (w1175:bool)
                  n778 = local read "Chop 3"() -> (w1174:bool)
                  n779 = local read "Chop 4"() -> (w1173:bool)
                  n780 = local read "Chop 7"() -> (w1172:bool)
                  n781 = local read "Chop 8"() -> (w1171:bool)
                  n782 = local read "Boast 3"() -> (w1156:bool)
                  n783 = local read "Boast 4"() -> (w1155:bool)
                  n784 = local read "Boast 7"() -> (w1154:bool)
                  n785 = local read "Boast 8"() -> (w1153:bool)
                  n786 = local read "Drop 3"() -> (w1180:bool)
                  n787 = local read "Drop 4"() -> (w1179:bool)
                  n788 = local read "Drop 7"() -> (w1178:bool)
                  n789 = local read "Drop 8"() -> (w1177:bool)
                  n790 = local read "lob 11"() -> (w1164:bool)
                  n791 = local read "lob 12"() -> (w1163:bool)
                  n792 = local read "lob 3"() -> (w1168:bool)
                  n793 = local read "lob 4"() -> (w1167:bool)
                  n794 = local read "lob 7"() -> (w1166:bool)
                  n795 = local read "lob 8"() -> (w1165:bool)
                  n796 = Compound Arithmetic op=OR(w1180, w1179, w1178, w1177, w1176, w1175, w1174, w1173, w1172, w1171, w1170, w1169, w1168, w1167, w1166, w1165, w1164, w1163, w1162, w1161, w1160, w1159, w1158, w1157, w1156, w1155, w1154, w1153, w1152, w1151) -> (w1181:bool)
                  n797 = local read "SWADrive 11"() -> (w1134:bool)
                  n798 = local read "SWADrive 12"() -> (w1133:bool)
                  n799 = local read "SWDDrive 11"() -> (w1128:bool)
                  n800 = local read "SWDDrive 12"() -> (w1127:bool)
                  n801 = local read "SWADrive 3"() -> (w1138:bool)
                  n802 = local read "SWADrive 4"() -> (w1137:bool)
                  n803 = local read "SWADrive 7"() -> (w1136:bool)
                  n804 = local read "SWADrive 8"() -> (w1135:bool)
                  n805 = local read "SWDDrive 3"() -> (w1132:bool)
                  n806 = local read "SWDDrive 4"() -> (w1131:bool)
                  n807 = local read "SWDDrive 7"() -> (w1130:bool)
                  n808 = local read "SWDDrive 8"() -> (w1129:bool)
                  n809 = local read "ADrive 11"() -> (w1146:bool)
                  n810 = local read "ADrive 12"() -> (w1145:bool)
                  n811 = local read "DDrive 11"() -> (w1140:bool)
                  n812 = local read "DDrive 12"() -> (w1139:bool)
                  n813 = local read "ADrive 3"() -> (w1150:bool)
                  n814 = local read "ADrive 4"() -> (w1149:bool)
                  n815 = local read "ADrive 7"() -> (w1148:bool)
                  n816 = local read "ADrive 8"() -> (w1147:bool)
                  n817 = local read "DDrive 3"() -> (w1144:bool)
                  n818 = local read "DDrive 4"() -> (w1143:bool)
                  n819 = local read "DDrive 7"() -> (w1142:bool)
                  n820 = local read "DDrive 8"() -> (w1141:bool)
                  n821 = Compound Arithmetic op=OR(w1150, w1149, w1148, w1147, w1146, w1145, w1144, w1143, w1142, w1141, w1140, w1139, w1138, w1137, w1136, w1135, w1134, w1133, w1132, w1131, w1130, w1129, w1128, w1127) -> (w1182:bool)
                  n822 = Or(x=w1181, y=w1182) -> (x .or. y?=w1183:bool)
                  n823 = Boolean To (0,1)(Boolean=w1183) -> (0, 1=w1126:i16)
                }
                frame #8 {
                  # "straight"
                  n824 = local read "Smash 11"() -> (w1209:bool)
                  n825 = local read "Chop 11"() -> (w1221:bool)
                  n826 = local read "Smash 3"() -> (w1213:bool)
                  n827 = local read "Smash 5"() -> (w1212:bool)
                  n828 = local read "Smash 7"() -> (w1211:bool)
                  n829 = local read "Smash 9"() -> (w1210:bool)
                  n830 = local read "Drop 11"() -> (w1227:bool)
                  n831 = local read "Chop 3"() -> (w1225:bool)
                  n832 = local read "Chop 5"() -> (w1224:bool)
                  n833 = local read "Chop 7"() -> (w1223:bool)
                  n834 = local read "Chop 9"() -> (w1222:bool)
                  n835 = local read "Drop 3"() -> (w1231:bool)
                  n836 = local read "Drop 5"() -> (w1230:bool)
                  n837 = local read "Drop 7"() -> (w1229:bool)
                  n838 = local read "Drop 9"() -> (w1228:bool)
                  n839 = local read "Smash"() -> (w1214:bool)
                  n840 = local read "lob 11"() -> (w1215:bool)
                  n841 = local read "Chop"() -> (w1226:bool)
                  n842 = local read "Drop"() -> (w1232:bool)
                  n843 = local read "lob 3"() -> (w1219:bool)
                  n844 = local read "lob 5"() -> (w1218:bool)
                  n845 = local read "lob 7"() -> (w1217:bool)
                  n846 = local read "lob 9"() -> (w1216:bool)
                  n847 = local read "lob 13"() -> (w1220:bool)
                  n848 = Compound Arithmetic op=OR(w1232, w1231, w1230, w1229, w1228, w1227, w1226, w1225, w1224, w1223, w1222, w1221, w1220, w1219, w1218, w1217, w1216, w1215, w1214, w1213, w1212, w1211, w1210, w1209) -> (w1233:bool)
                  n849 = local read "SWADrive 11"() -> (w1191:bool)
                  n850 = local read "SWDDrive 11"() -> (w1185:bool)
                  n851 = local read "SWADrive 3"() -> (w1195:bool)
                  n852 = local read "SWADrive 5"() -> (w1194:bool)
                  n853 = local read "SWADrive 7"() -> (w1193:bool)
                  n854 = local read "SWADrive 9"() -> (w1192:bool)
                  n855 = local read "SWDDrive 3"() -> (w1189:bool)
                  n856 = local read "SWDDrive 5"() -> (w1188:bool)
                  n857 = local read "SWDDrive 7"() -> (w1187:bool)
                  n858 = local read "SWDDrive 9"() -> (w1186:bool)
                  n859 = local read "SWADrive"() -> (w1196:bool)
                  n860 = local read "SWDDrive"() -> (w1190:bool)
                  n861 = local read "ADrive 11"() -> (w1203:bool)
                  n862 = local read "DDrive 11"() -> (w1197:bool)
                  n863 = local read "ADrive 3"() -> (w1207:bool)
                  n864 = local read "ADrive 5"() -> (w1206:bool)
                  n865 = local read "ADrive 7"() -> (w1205:bool)
                  n866 = local read "ADrive 9"() -> (w1204:bool)
                  n867 = local read "DDrive 3"() -> (w1201:bool)
                  n868 = local read "DDrive 5"() -> (w1200:bool)
                  n869 = local read "DDrive 7"() -> (w1199:bool)
                  n870 = local read "DDrive 9"() -> (w1198:bool)
                  n871 = local read "ADrive"() -> (w1208:bool)
                  n872 = local read "DDrive"() -> (w1202:bool)
                  n873 = Compound Arithmetic op=OR(w1208, w1207, w1206, w1205, w1204, w1203, w1202, w1201, w1200, w1199, w1198, w1197, w1196, w1195, w1194, w1193, w1192, w1191, w1190, w1189, w1188, w1187, w1186, w1185) -> (w1234:bool)
                  n874 = Or(x=w1233, y=w1234) -> (x .or. y?=w1235:bool)
                  n875 = Boolean To (0,1)(Boolean=w1235) -> (0, 1=w1184:i16)
                  "Straight" <- w1184
                }
                frame #9 {
                  # "cross"
                  n876 = local read "Smash 10"() -> (w1275:bool)
                  n877 = local read "Smash 12"() -> (w1274:bool)
                  n878 = local read "Chop 10"() -> (w1287:bool)
                  n879 = local read "Chop 12"() -> (w1286:bool)
                  n880 = local read "Smash 2"() -> (w1279:bool)
                  n881 = local read "Smash 4"() -> (w1278:bool)
                  n882 = local read "Smash 6"() -> (w1277:bool)
                  n883 = local read "Smash 8"() -> (w1276:bool)
                  n884 = local read "Boast 10"() -> (w1264:bool)
                  n885 = local read "Boast 11"() -> (w1263:bool)
                  n886 = local read "Boast 12"() -> (w1262:bool)
                  n887 = local read "Drop 10"() -> (w1293:bool)
                  n888 = local read "Drop 12"() -> (w1292:bool)
                  n889 = local read "Chop 2"() -> (w1291:bool)
                  n890 = local read "Chop 4"() -> (w1290:bool)
                  n891 = local read "Chop 6"() -> (w1289:bool)
                  n892 = local read "Chop 8"() -> (w1288:bool)
                  n893 = local read "Boast 2"() -> (w1272:bool)
                  n894 = local read "Boast 3"() -> (w1271:bool)
                  n895 = local read "Boast 4"() -> (w1270:bool)
                  n896 = local read "Boast 5"() -> (w1269:bool)
                  n897 = local read "Boast 6"() -> (w1268:bool)
                  n898 = local read "Boast 7"() -> (w1267:bool)
                  n899 = local read "Boast 8"() -> (w1266:bool)
                  n900 = local read "Boast 9"() -> (w1265:bool)
                  n901 = local read "Drop 2"() -> (w1297:bool)
                  n902 = local read "Drop 4"() -> (w1296:bool)
                  n903 = local read "Drop 6"() -> (w1295:bool)
                  n904 = local read "Drop 8"() -> (w1294:bool)
                  n905 = local read "lob 10"() -> (w1281:bool)
                  n906 = local read "lob 12"() -> (w1280:bool)
                  n907 = local read "Boast"() -> (w1273:bool)
                  n908 = local read "lob 2"() -> (w1285:bool)
                  n909 = local read "lob 4"() -> (w1284:bool)
                  n910 = local read "lob 6"() -> (w1283:bool)
                  n911 = local read "lob 8"() -> (w1282:bool)
                  n912 = Compound Arithmetic op=OR(w1297, w1296, w1295, w1294, w1293, w1292, w1291, w1290, w1289, w1288, w1287, w1286, w1285, w1284, w1283, w1282, w1281, w1280, w1279, w1278, w1277, w1276, w1275, w1274, w1273, w1272, w1271, w1270, w1269, w1268, w1267, w1266, w1265, w1264, w1263, w1262) -> (w1237:bool)
                  n913 = local read "SWADrive 10"() -> (w1245:bool)
                  n914 = local read "SWADrive 12"() -> (w1244:bool)
                  n915 = local read "SWDDrive 10"() -> (w1239:bool)
                  n916 = local read "SWDDrive 12"() -> (w1238:bool)
                  n917 = local read "SWADrive 2"() -> (w1249:bool)
                  n918 = local read "SWADrive 4"() -> (w1248:bool)
                  n919 = local read "SWADrive 6"() -> (w1247:bool)
                  n920 = local read "SWADrive 8"() -> (w1246:bool)
                  n921 = local read "SWDDrive 2"() -> (w1243:bool)
                  n922 = local read "SWDDrive 4"() -> (w1242:bool)
                  n923 = local read "SWDDrive 6"() -> (w1241:bool)
                  n924 = local read "SWDDrive 8"() -> (w1240:bool)
                  n925 = local read "ADrive 10"() -> (w1257:bool)
                  n926 = local read "ADrive 12"() -> (w1256:bool)
                  n927 = local read "DDrive 10"() -> (w1251:bool)
                  n928 = local read "DDrive 12"() -> (w1250:bool)
                  n929 = local read "ADrive 2"() -> (w1261:bool)
                  n930 = local read "ADrive 4"() -> (w1260:bool)
                  n931 = local read "ADrive 6"() -> (w1259:bool)
                  n932 = local read "ADrive 8"() -> (w1258:bool)
                  n933 = local read "DDrive 2"() -> (w1255:bool)
                  n934 = local read "DDrive 4"() -> (w1254:bool)
                  n935 = local read "DDrive 6"() -> (w1253:bool)
                  n936 = local read "DDrive 8"() -> (w1252:bool)
                  n937 = Compound Arithmetic op=OR(w1261, w1260, w1259, w1258, w1257, w1256, w1255, w1254, w1253, w1252, w1251, w1250, w1249, w1248, w1247, w1246, w1245, w1244, w1243, w1242, w1241, w1240, w1239, w1238) -> (w1298:bool)
                  n938 = Or(x=w1237, y=w1298) -> (x .or. y?=w1299:bool)
                  n939 = Boolean To (0,1)(Boolean=w1299) -> (0, 1=w1236:i16)
                  "Cross" <- w1236
                }
                frame #10 {
                  # "bounce"
                  n940 = local read "Smash 2"() -> (w1307:bool)
                  n941 = local read "Smash 3"() -> (w1306:bool)
                  n942 = local read "Smash 4"() -> (w1305:bool)
                  n943 = local read "Chop 2"() -> (w1331:bool)
                  n944 = local read "Chop 3"() -> (w1330:bool)
                  n945 = local read "Chop 4"() -> (w1329:bool)
                  n946 = local read "Boast 2"() -> (w1303:bool)
                  n947 = local read "Boast 3"() -> (w1302:bool)
                  n948 = local read "Boast 4"() -> (w1301:bool)
                  n949 = local read "Drop 2"() -> (w1335:bool)
                  n950 = local read "Drop 3"() -> (w1334:bool)
                  n951 = local read "Drop 4"() -> (w1333:bool)
                  n952 = local read "Smash"() -> (w1308:bool)
                  n953 = local read "Chop"() -> (w1332:bool)
                  n954 = local read "Boast"() -> (w1304:bool)
                  n955 = local read "Drop"() -> (w1336:bool)
                  n956 = local read "lob 2"() -> (w1310:bool)
                  n957 = local read "lob 3"() -> (w1311:bool)
                  n958 = local read "lob 4"() -> (w1309:bool)
                  n959 = local read "lob 13"() -> (w1312:bool)
                  n960 = Compound Arithmetic op=OR(w1336, w1335, w1334, w1333, w1332, w1331, w1330, w1329, w1312, w1310, w1311, w1309, w1308, w1307, w1306, w1305, w1304, w1303, w1302, w1301) -> (w1337:bool)
                  n961 = local read "SWADrive 2"() -> (w1319:bool)
                  n962 = local read "SWADrive 3"() -> (w1318:bool)
                  n963 = local read "SWADrive 4"() -> (w1317:bool)
                  n964 = local read "SWDDrive 2"() -> (w1315:bool)
                  n965 = local read "SWDDrive 3"() -> (w1314:bool)
                  n966 = local read "SWDDrive 4"() -> (w1313:bool)
                  n967 = local read "SWADrive"() -> (w1320:bool)
                  n968 = local read "SWDDrive"() -> (w1316:bool)
                  n969 = local read "ADrive 2"() -> (w1327:bool)
                  n970 = local read "ADrive 3"() -> (w1326:bool)
                  n971 = local read "ADrive 4"() -> (w1325:bool)
                  n972 = local read "DDrive 2"() -> (w1323:bool)
                  n973 = local read "DDrive 3"() -> (w1322:bool)
                  n974 = local read "DDrive 4"() -> (w1321:bool)
                  n975 = local read "ADrive"() -> (w1328:bool)
                  n976 = local read "DDrive"() -> (w1324:bool)
                  n977 = Compound Arithmetic op=OR(w1328, w1327, w1326, w1325, w1324, w1323, w1322, w1321, w1320, w1319, w1318, w1317, w1316, w1315, w1314, w1313) -> (w1338:bool)
                  n978 = Or(x=w1337, y=w1338) -> (x .or. y?=w1339:bool)
                  n979 = Boolean To (0,1)(Boolean=w1339) -> (0, 1=w1300:i16)
                }
                frame #11 {
                  # "volley"
                  n980 = local read "Smash 5"() -> (w1364:bool)
                  n981 = local read "Smash 6"() -> (w1363:bool)
                  n982 = local read "Smash 7"() -> (w1362:bool)
                  n983 = local read "Smash 8"() -> (w1361:bool)
                  n984 = local read "Chop 5"() -> (w1372:bool)
                  n985 = local read "Chop 6"() -> (w1371:bool)
                  n986 = local read "Chop 7"() -> (w1370:bool)
                  n987 = local read "Chop 8"() -> (w1369:bool)
                  n988 = local read "Boast 5"() -> (w1360:bool)
                  n989 = local read "Boast 6"() -> (w1359:bool)
                  n990 = local read "Boast 7"() -> (w1358:bool)
                  n991 = local read "Boast 8"() -> (w1357:bool)
                  n992 = local read "Drop 5"() -> (w1376:bool)
                  n993 = local read "Drop 6"() -> (w1375:bool)
                  n994 = local read "Drop 7"() -> (w1374:bool)
                  n995 = local read "Drop 8"() -> (w1373:bool)
                  n996 = local read "lob 5"() -> (w1368:bool)
                  n997 = local read "lob 6"() -> (w1367:bool)
                  n998 = local read "lob 7"() -> (w1366:bool)
                  n999 = local read "lob 8"() -> (w1365:bool)
                  n1000 = Compound Arithmetic op=OR(w1376, w1375, w1374, w1373, w1372, w1371, w1370, w1369, w1368, w1367, w1366, w1365, w1364, w1363, w1362, w1361, w1360, w1359, w1358, w1357) -> (w1377:bool)
                  n1001 = local read "SWADrive 5"() -> (w1348:bool)
                  n1002 = local read "SWADrive 6"() -> (w1347:bool)
                  n1003 = local read "SWADrive 7"() -> (w1346:bool)
                  n1004 = local read "SWADrive 8"() -> (w1345:bool)
                  n1005 = local read "SWDDrive 5"() -> (w1344:bool)
                  n1006 = local read "SWDDrive 6"() -> (w1343:bool)
                  n1007 = local read "SWDDrive 7"() -> (w1342:bool)
                  n1008 = local read "SWDDrive 8"() -> (w1341:bool)
                  n1009 = local read "ADrive 5"() -> (w1356:bool)
                  n1010 = local read "ADrive 6"() -> (w1355:bool)
                  n1011 = local read "ADrive 7"() -> (w1354:bool)
                  n1012 = local read "ADrive 8"() -> (w1353:bool)
                  n1013 = local read "DDrive 5"() -> (w1352:bool)
                  n1014 = local read "DDrive 6"() -> (w1351:bool)
                  n1015 = local read "DDrive 7"() -> (w1350:bool)
                  n1016 = local read "DDrive 8"() -> (w1349:bool)
                  n1017 = Compound Arithmetic op=OR(w1356, w1355, w1354, w1353, w1352, w1351, w1350, w1349, w1348, w1347, w1346, w1345, w1344, w1343, w1342, w1341) -> (w1378:bool)
                  n1018 = Or(x=w1377, y=w1378) -> (x .or. y?=w1379:bool)
                  n1019 = Boolean To (0,1)(Boolean=w1379) -> (0, 1=w1340:i16)
                }
                frame #12 {
                  # "half volley"
                  n1020 = local read "Smash 10"() -> (w1403:bool)
                  n1021 = local read "Smash 11"() -> (w1402:bool)
                  n1022 = local read "Smash 12"() -> (w1401:bool)
                  n1023 = local read "Chop 10"() -> (w1411:bool)
                  n1024 = local read "Chop 11"() -> (w1410:bool)
                  n1025 = local read "Chop 12"() -> (w1409:bool)
                  n1026 = local read "Smash 9"() -> (w1404:bool)
                  n1027 = local read "Boast 10"() -> (w1399:bool)
                  n1028 = local read "Boast 11"() -> (w1398:bool)
                  n1029 = local read "Boast 12"() -> (w1397:bool)
                  n1030 = local read "Drop 10"() -> (w1415:bool)
                  n1031 = local read "Drop 11"() -> (w1414:bool)
                  n1032 = local read "Drop 12"() -> (w1413:bool)
                  n1033 = local read "Chop 9"() -> (w1412:bool)
                  n1034 = local read "Boast 9"() -> (w1400:bool)
                  n1035 = local read "Drop 9"() -> (w1416:bool)
                  n1036 = local read "lob 10"() -> (w1407:bool)
                  n1037 = local read "lob 11"() -> (w1406:bool)
                  n1038 = local read "lob 12"() -> (w1405:bool)
                  n1039 = local read "lob 9"() -> (w1408:bool)
                  n1040 = Compound Arithmetic op=OR(w1416, w1415, w1414, w1413, w1412, w1411, w1410, w1409, w1408, w1407, w1406, w1405, w1404, w1403, w1402, w1401, w1400, w1399, w1398, w1397) -> (w1417:bool)
                  n1041 = local read "SWADrive 10"() -> (w1387:bool)
                  n1042 = local read "SWADrive 11"() -> (w1386:bool)
                  n1043 = local read "SWADrive 12"() -> (w1385:bool)
                  n1044 = local read "SWDDrive 10"() -> (w1383:bool)
                  n1045 = local read "SWDDrive 11"() -> (w1382:bool)
                  n1046 = local read "SWDDrive 12"() -> (w1381:bool)
                  n1047 = local read "SWADrive 9"() -> (w1388:bool)
                  n1048 = local read "SWDDrive 9"() -> (w1384:bool)
                  n1049 = local read "ADrive 10"() -> (w1395:bool)
                  n1050 = local read "ADrive 11"() -> (w1394:bool)
                  n1051 = local read "ADrive 12"() -> (w1393:bool)
                  n1052 = local read "DDrive 10"() -> (w1391:bool)
                  n1053 = local read "DDrive 11"() -> (w1390:bool)
                  n1054 = local read "DDrive 12"() -> (w1389:bool)
                  n1055 = local read "ADrive 9"() -> (w1396:bool)
                  n1056 = local read "DDrive 9"() -> (w1392:bool)
                  n1057 = Compound Arithmetic op=OR(w1396, w1395, w1394, w1393, w1392, w1391, w1390, w1389, w1388, w1387, w1386, w1385, w1384, w1383, w1382, w1381) -> (w1418:bool)
                  n1058 = Or(x=w1417, y=w1418) -> (x .or. y?=w1419:bool)
                  n1059 = Boolean To (0,1)(Boolean=w1419) -> (0, 1=w1380:i16)
                }
                frame #13 {
                  n1060 = local read "Player1/Player2"() -> (w1430:bool[])
                  n1061 = Index Array(array=w1430) -> (element #1=w1431:bool, element #2=w1432:bool)  [unwired: 2 in]
                  n1062 = Boolean To (0,1)(Boolean=w1432) -> (0, 1=w1420:i16)
                  n1063 = Boolean To (0,1)(Boolean=w1431) -> (0, 1=w1421:i16)
                  n1064 = Compound Arithmetic op=OR("Service1", "Service2", "S1", "S2", "S3", "S4", "S5", "S6") -> (w1442:bool)
                  n1065 = Boolean To (0,1)(Boolean=w1442) -> (0, 1=→"Service":i16)
                  n1066 = Boolean To (0,1)(Boolean="Service1") -> (0, 1=w1429:i16)
                  n1067 = Boolean To (0,1)(Boolean="Service2") -> (0, 1=w1428:i16)
                  n1068 = Boolean To (0,1)(Boolean="S1") -> (0, 1=w1427:i16)
                  n1069 = Boolean To (0,1)(Boolean="S2") -> (0, 1=w1426:i16)
                  n1070 = Boolean To (0,1)(Boolean="S3") -> (0, 1=w1425:i16)
                  n1071 = Boolean To (0,1)(Boolean="S4") -> (0, 1=w1424:i16)
                  n1072 = Boolean To (0,1)(Boolean="S5") -> (0, 1=w1423:i16)
                  n1073 = Boolean To (0,1)(Boolean="S6") -> (0, 1=w1422:i16)
                }
                frame #14 {
                  w1458 = 0 ("disabled index (col)")
                  n1074 = Index Array(array=w1480, index (col) #1=51 ("disabled index (col)"), index (col) #2=52 ("index (col)"), index (col) #3=0 ("index (col)")) -> (element #1=w1469:i64[], element #2=w1468:i64[], element #3=w1471:i64[])  [unwired: 3 in]
                  n1075 = Or(x=w1469, y=w1468) -> (x .or. y?=w1476:i64[])
                  n1076 = Reverse 1D Array(array=w1476) -> (reversed array=w1475:i64[])
                  n1077 = Reverse 1D Array(array=w1471) -> (reversed array=w1473:i64[])
                  n1078 = Compound Arithmetic op=OR("Expected Winner1", "Unexpected Winner1", "Stroke1", "Forced Error2", "Unforced Error2", "Nolet2") -> (w1490:bool)
                  n1079 = Search 1D Array(1D array=w1475, element=i64 1) -> (index of element=w1472:i32)  [unwired: 1 in]
                  n1080 = Boolean To (0,1)(Boolean=w1490) -> (0, 1=w1456:i16)
                  n1081 = Compound Arithmetic op=OR("Expected Winner2", "Unexpected Winner2", "Stroke2", "Forced Error1", "Unforced Error1", "Nolet1") -> (w1489:bool)
                  n1082 = Boolean To (0,1)(Boolean="Expected Winner1") -> (0, 1=w1443:i16)
                  n1083 = Boolean To (0,1)(Boolean="Expected Winner2") -> (0, 1=w1444:i16)
                  n1084 = Boolean To (0,1)(Boolean="Unexpected Winner1") -> (0, 1=w1445:i16)
                  n1085 = Boolean To (0,1)(Boolean="Unexpected Winner2") -> (0, 1=w1446:i16)
                  n1086 = Boolean To (0,1)(Boolean="Stroke1") -> (0, 1=w1447:i16)
                  n1087 = Boolean To (0,1)(Boolean="Stroke2") -> (0, 1=w1448:i16)
                  n1088 = Boolean To (0,1)(Boolean="Forced Error1") -> (0, 1=w1449:i16)
                  n1089 = Boolean To (0,1)(Boolean="Forced Error2") -> (0, 1=w1450:i16)
                  n1090 = Boolean To (0,1)(Boolean="Unforced Error1") -> (0, 1=w1451:i16)
                  n1091 = Boolean To (0,1)(Boolean="Unforced Error2") -> (0, 1=w1452:i16)
                  n1092 = Boolean To (0,1)(Boolean="Nolet1") -> (0, 1=w1453:i16)
                  n1093 = Boolean To (0,1)(Boolean="Nolet2") -> (0, 1=w1454:i16)
                  n1094 = Boolean To (0,1)(Boolean="Let") -> (0, 1=w1455:i16)
                  n1095 = Index Array(array=w1473, index=w1472) -> (element=w1470:i64)
                  n1096 = Boolean To (0,1)(Boolean=w1489) -> (0, 1=w1457:i16)
                  n1097 = Search 1D Array(1D array=w1471, element=w1470) -> (index of element=w1467:i32)  [unwired: 1 in]
                  n1098 = Not Equal To 0?(x=w1456) -> (x != 0?=w1482:bool)
                  n1099 = Not Equal To 0?(x=w1457) -> (x != 0?=w1481:bool)
                  n1100 = Build Array(w1482, w1481) -> (w1459:bool[])
                  n1101 = Index Array(array=w1468, index=w1467) -> (element=w1463:i64)
                  n1102 = Index Array(array=w1469, index=w1467) -> (element=w1464:i64)
                  n1103 = Not Equal To 0?(x=w1464) -> (x != 0?=w1465:bool)
                  n1104 = Not Equal To 0?(x=w1463) -> (x != 0?=w1466:bool)
                  n1105 = Build Array(w1465, w1466) -> (w1460:bool[])
                  n1106 = Select(t=w1460, s="Let", f=w1459) -> (s? t:f=w1462:bool[])
                  n1107 = local write "Score change"(w1462) -> ()
                }
                frame #15 {
                  w1497 = FALSE ("4 6")
                  n1108 = local read "Service"() -> (w1506:i16)
                  n1109 = local read "Cross"() -> (w1505:i16)
                  n1110 = local read "Straight"() -> (w1504:i16)
                  n1111 = local read "position"() -> (w1503:i16)
                  n1112 = local read "Player 1/2"() -> (w1502:i16)
                  n1113 = local read "Extra"() -> (w1501:i16)
                  n1114 = local write "Drop"(w1497) -> ()
                  n1115 = local write "Drop 2"(w1497) -> ()
                  n1116 = local write "Drop 3"(w1497) -> ()
                  n1117 = local write "Drop 4"(w1497) -> ()
                  n1118 = local write "Drop 5"(w1497) -> ()
                  n1119 = local write "Drop 6"(w1497) -> ()
                  n1120 = local write "Drop 7"(w1497) -> ()
                  n1121 = local write "Drop 8"(w1497) -> ()
                  n1122 = local write "Drop 9"(w1497) -> ()
                  n1123 = local write "Drop 10"(w1497) -> ()
                  n1124 = local write "Drop 11"(w1497) -> ()
                  n1125 = local write "Drop 12"(w1497) -> ()
                  n1126 = local write "Chop"(w1497) -> ()
                  n1127 = local write "Chop 2"(w1497) -> ()
                  n1128 = local write "Chop 3"(w1497) -> ()
                  n1129 = local write "Chop 4"(w1497) -> ()
                  n1130 = local write "Chop 5"(w1497) -> ()
                  n1131 = local write "Chop 6"(w1497) -> ()
                  n1132 = local write "Chop 7"(w1497) -> ()
                  n1133 = local write "Chop 8"(w1497) -> ()
                  n1134 = local write "Chop 9"(w1497) -> ()
                  n1135 = local write "Chop 10"(w1497) -> ()
                  n1136 = local write "Chop 11"(w1497) -> ()
                  n1137 = local write "Chop 12"(w1497) -> ()
                  n1138 = Compound Arithmetic op=ADD(w1506, w1505, w1504, w1503, w1502, w1501) -> (w1500:i16)
                  n1139 = Equal To 0?(x=w1500) -> (x = 0?=w1499:bool)
                  n1140 = local write "lob 13"(w1497) -> ()
                  n1141 = local write "lob 2"(w1497) -> ()
                  n1142 = local write "lob 3"(w1497) -> ()
                  n1143 = local write "lob 4"(w1497) -> ()
                  n1144 = local write "lob 5"(w1497) -> ()
                  n1145 = local write "lob 6"(w1497) -> ()
                  n1146 = local write "lob 7"(w1497) -> ()
                  n1147 = local write "lob 8"(w1497) -> ()
                  n1148 = local write "lob 9"(w1497) -> ()
                  n1149 = local write "lob 10"(w1497) -> ()
                  n1150 = local write "lob 11"(w1497) -> ()
                  n1151 = local write "lob 12"(w1497) -> ()
                  n1152 = local write "Smash"(w1497) -> ()
                  n1153 = local write "Smash 2"(w1497) -> ()
                  n1154 = local write "Smash 3"(w1497) -> ()
                  n1155 = local write "Smash 4"(w1497) -> ()
                  n1156 = local write "Smash 5"(w1497) -> ()
                  n1157 = local write "Smash 6"(w1497) -> ()
                  n1158 = local write "Smash 7"(w1497) -> ()
                  n1159 = local write "Smash 8"(w1497) -> ()
                  n1160 = local write "Smash 9"(w1497) -> ()
                  n1161 = local write "Smash 10"(w1497) -> ()
                  n1162 = local write "Smash 11"(w1497) -> ()
                  n1163 = local write "Smash 12"(w1497) -> ()
                  n1164 = case shown="True" "Auto switch" {
                    tunnel: w1499 -> [_ w1507]
                    frame False {
                    }
                    frame True {
                      n1165 = local read "Player1/Player2"() -> (w1513:bool[])
                      n1166 = local read "Player1/Player2"() -> (w1514:bool[])
                      n1167 = Reverse 1D Array(array=w1513) -> (reversed array=w1512:bool[])
                      n1168 = Select(t=w1514, s=w1507, f=w1512) -> (s? t:f=w1508:bool[])
                      n1169 = local read "Score change"() -> (w1510:bool[])
                      n1170 = Or Array Elements(Boolean array=w1510) -> (logical OR=w1511:bool)
                      n1171 = Select(t=w1510, s=w1511, f=w1508) -> (s? t:f=w1509:bool[])
                      n1172 = local write "Player1/Player2"(w1509) -> ()
                    }
                  }
                  n1173 = local write "ADrive"(w1497) -> ()
                  n1174 = local write "ADrive 2"(w1497) -> ()
                  n1175 = local write "ADrive 3"(w1497) -> ()
                  n1176 = local write "ADrive 4"(w1497) -> ()
                  n1177 = local write "ADrive 5"(w1497) -> ()
                  n1178 = local write "ADrive 6"(w1497) -> ()
                  n1179 = local write "ADrive 7"(w1497) -> ()
                  n1180 = local write "ADrive 8"(w1497) -> ()
                  n1181 = local write "ADrive 9"(w1497) -> ()
                  n1182 = local write "ADrive 10"(w1497) -> ()
                  n1183 = local write "ADrive 11"(w1497) -> ()
                  n1184 = local write "ADrive 12"(w1497) -> ()
                  n1185 = local write "DDrive"(w1497) -> ()
                  n1186 = local write "DDrive 2"(w1497) -> ()
                  n1187 = local write "DDrive 3"(w1497) -> ()
                  n1188 = local write "DDrive 4"(w1497) -> ()
                  n1189 = local write "DDrive 5"(w1497) -> ()
                  n1190 = local write "DDrive 6"(w1497) -> ()
                  n1191 = local write "DDrive 7"(w1497) -> ()
                  n1192 = local write "DDrive 8"(w1497) -> ()
                  n1193 = local write "DDrive 9"(w1497) -> ()
                  n1194 = local write "DDrive 10"(w1497) -> ()
                  n1195 = local write "DDrive 11"(w1497) -> ()
                  n1196 = local write "DDrive 12"(w1497) -> ()
                  n1197 = local write "SWADrive"(w1497) -> ()
                  n1198 = local write "SWADrive 2"(w1497) -> ()
                  n1199 = local write "SWADrive 3"(w1497) -> ()
                  n1200 = local write "SWADrive 4"(w1497) -> ()
                  n1201 = local write "SWADrive 5"(w1497) -> ()
                  n1202 = local write "SWADrive 6"(w1497) -> ()
                  n1203 = local write "SWADrive 7"(w1497) -> ()
                  n1204 = local write "SWADrive 8"(w1497) -> ()
                  n1205 = local write "SWADrive 9"(w1497) -> ()
                  n1206 = local write "SWADrive 10"(w1497) -> ()
                  n1207 = local write "SWADrive 11"(w1497) -> ()
                  n1208 = local write "SWADrive 12"(w1497) -> ()
                  n1209 = local write "SWDDrive"(w1497) -> ()
                  n1210 = local write "SWDDrive 2"(w1497) -> ()
                  n1211 = local write "SWDDrive 3"(w1497) -> ()
                  n1212 = local write "SWDDrive 4"(w1497) -> ()
                  n1213 = local write "SWDDrive 5"(w1497) -> ()
                  n1214 = local write "SWDDrive 6"(w1497) -> ()
                  n1215 = local write "SWDDrive 7"(w1497) -> ()
                  n1216 = local write "SWDDrive 8"(w1497) -> ()
                  n1217 = local write "SWDDrive 9"(w1497) -> ()
                  n1218 = local write "SWDDrive 10"(w1497) -> ()
                  n1219 = local write "SWDDrive 11"(w1497) -> ()
                  n1220 = local write "SWDDrive 12"(w1497) -> ()
                  n1221 = local write "Boast"(w1497) -> ()
                  n1222 = local write "Boast 2"(w1497) -> ()
                  n1223 = local write "Boast 3"(w1497) -> ()
                  n1224 = local write "Boast 4"(w1497) -> ()
                  n1225 = local write "Boast 5"(w1497) -> ()
                  n1226 = local write "Boast 6"(w1497) -> ()
                  n1227 = local write "Boast 7"(w1497) -> ()
                  n1228 = local write "Boast 8"(w1497) -> ()
                  n1229 = local write "Boast 9"(w1497) -> ()
                  n1230 = local write "Boast 10"(w1497) -> ()
                  n1231 = local write "Boast 11"(w1497) -> ()
                  n1232 = local write "Boast 12"(w1497) -> ()
                  n1233 = local write "4 4"(w1497) -> ()
                  n1234 = local write "4 3"(w1497) -> ()
                  n1235 = local write "4 2"(w1497) -> ()
                  n1236 = local write "4 1"(w1497) -> ()
                  n1237 = local write "3 4"(w1497) -> ()
                  n1238 = local write "3 3"(w1497) -> ()
                  n1239 = local write "3 2"(w1497) -> ()
                  n1240 = local write "3 1"(w1497) -> ()
                  n1241 = local write "2 4"(w1497) -> ()
                  n1242 = local write "2 3"(w1497) -> ()
                  n1243 = local write "2 2"(w1497) -> ()
                  n1244 = local write "2 1"(w1497) -> ()
                  n1245 = local write "1 4"(w1497) -> ()
                  n1246 = local write "1 3"(w1497) -> ()
                  n1247 = local write "1 2"(w1497) -> ()
                  n1248 = local write "1 1"(w1497) -> ()
                  n1249 = local write "5 4"(w1497) -> ()
                  n1250 = local write "5 3"(w1497) -> ()
                  n1251 = local write "5 2"(w1497) -> ()
                  n1252 = local write "5 1"(w1497) -> ()
                  n1253 = local write "6 4"(w1497) -> ()
                  n1254 = local write "6 3"(w1497) -> ()
                  n1255 = local write "6 2"(w1497) -> ()
                  n1256 = local write "6 1"(w1497) -> ()
                  n1257 = local write "S6"(w1497) -> ()
                  n1258 = local write "S5"(w1497) -> ()
                  n1259 = local write "S4"(w1497) -> ()
                  n1260 = local write "S1"(w1497) -> ()
                  n1261 = local write "S2"(w1497) -> ()
                  n1262 = local write "S3"(w1497) -> ()
                  n1263 = local write "Let"(w1497) -> ()
                  n1264 = local write "Unexpected Winner2"(w1497) -> ()
                  n1265 = local write "Unexpected Winner1"(w1497) -> ()
                  n1266 = local write "Expected Winner2"(w1497) -> ()
                  n1267 = local write "Expected Winner1"(w1497) -> ()
                  n1268 = local write "Forced Error2"(w1497) -> ()
                  n1269 = local write "Forced Error1"(w1497) -> ()
                  n1270 = local write "Service2"(w1497) -> ()
                  n1271 = local write "Service1"(w1497) -> ()
                  n1272 = local write "Nolet2"(w1497) -> ()
                  n1273 = local write "Nolet1"(w1497) -> ()
                  n1274 = local write "Stroke2"(w1497) -> ()
                  n1275 = local write "Stroke1"(w1497) -> ()
                  n1276 = local write "Unforced Error2"(w1497) -> ()
                  n1277 = local write "Unforced Error1"(w1497) -> ()
                  n1278 = local write "Player1"(w1497) -> ()
                  n1279 = local write "Player2"(w1497) -> ()
                  n1280 = local write "Button 5"(w1497) -> ()
                  n1281 = local write "Button 4"(w1497) -> ()
                  n1282 = local write "Button 3"(w1497) -> ()
                  n1283 = local write "Button 2"(w1497) -> ()
                  n1284 = local write "Button 1"(w1497) -> ()
                }
              }
              n1285 = Build Array(w640, w753, w752, w751, w750, w749, w748, w747, w746, w745, w744, w743, w742, w741, w740, w739, w738, w737, w736, w735, w734, w733, w732, w731, w730, w729, w728, w727, w726, w725, w724, w723, w722, w721, w720, w719, w718, w717, w716, w715, w714, w713, w712, w711, w710, w709, w708, w697, w696, w695, w694, w707, w706, w705, w704, w703, w702, w701, w700, w699, w698, w664, w663, w662, w661, w660, w651, w650, w649, w648, w647, w646, w645, w644, w643, w652, w584, w583, w582, w581, w580) -> (w635:u32[])
              n1286 = call "IMAQ Dispose"("Image"=w754) -> ()  [unwired: 5 in, 1 out]
              n1287 = Index Array(array=w637, index (col)=0 ("disabled index (col)")) -> (element=w762:i64[])  [unwired: 1 in]
              n1288 = Delete From Array(array=w635, index=0) -> (array with subset deleted=w682:u32[])  [unwired: 1 in, 1 out]
              n1289 = for {
                tunnel: w762 -> [w780] mode=indexing
                tunnel: w640 -> [w781]
                tunnel: [w780] -> w760 mode=indexing if=w782
                stop <- w782 continue-if-true
                n1290 = Less Or Equal?(x=w780, y=w781) -> (x <= y?=w782:bool)
              }
              n1291 = Delete From Array(array=w682, length=2, index=68) -> (array with subset deleted=w623:u32[])  [unwired: 1 out]
              n1292 = Array Size(array=w760) -> (size(s)=w636:i32)
              n1293 = Delete From Array(array=w623, length=17, index=43) -> (deleted portion=w676:u32[], array with subset deleted=w680:u32[])
              n1294 = Delete From Array(array=w623, length=2, index=0) -> (array with subset deleted=w620:u32[])  [unwired: 1 out]
              n1295 = Decrement(x=w636) -> (x-1=w674:i32)
              n1296 = Array Max & Min(array=w680) -> (max value=w681:u32)  [unwired: 3 out]
              n1297 = Array Max & Min(array=w676) -> (max value=w683:u32)  [unwired: 3 out]
              n1298 = Equal To 0?(x=w681) -> ()  [unwired: 1 out]
              n1299 = Not Equal To 0?(x=w683) -> (x != 0?=w679:bool)
              n1300 = Index Array(array=w637, index (row)=w674) -> (element=w677:i64[])  [unwired: 1 in]
              n1301 = Array Max & Min(array=w620) -> (max value=w756:u32)  [unwired: 3 out]
              n1302 = Compound Arithmetic op=AND(w669, w679, "Link Errors") -> (w638:bool)
              n1303 = Decrement(x=w636) -> (x-1=w670:i32)
              n1304 = Replace Array Subset(array=w677, new element=w676, index=44) -> (w634:i64[])
              n1305 = Equal To 0?(x=w756) -> (x = 0?=w626:bool)
              n1306 = Index Array(array=w634, index=w633) -> (element=w632:i64)
              n1307 = Replace Array Subset(array=w637, new element=w634, index (row)=w670) -> (w673:i64[][])  [unwired: 1 in]
              n1308 = Insert Into Array(array=w637, index (row)=w636, new element=w635) -> (w672:i64[][])  [unwired: 1 in]
              n1309 = Index Array(array=w635, index=w633) -> (element=w631:u32)
              n1310 = local read "last saved data"() -> (w629:i64[])
              n1311 = Select(t=w673, s=w638, f=w672) -> (s? t:f=w671:i64[][])
              n1312 = Select(t=w632, s=w638, f=w631) -> (s? t:f=w624:i64)
              n1313 = Select(t=w637, s=w626, f=w671) -> (s? t:f=w639:i64[][])
              n1314 = Search 1D Array(1D array=w629, element=w624) -> (index of element=w628:i32)  [unwired: 1 in]
              n1315 = Greater Than 0?(x=w628) -> (x > 0?=w627:bool)
              n1316 = Insert Into Array(array=w629, new element=w624) -> (w630:i64[])  [unwired: 1 in]
              n1317 = Or(x=w627, y=w626) -> (x .or. y?=w625:bool)
              n1318 = Select(t=w629, s=w625, f=w630) -> (s? t:f=w618:i64[])
              n1319 = case shown="False" "Undo" {
                tunnel: w639 -> [w764 w766]
                tunnel: [w764 w765] -> w616
                tunnel: w618 -> [w763 w775]
                tunnel: [w763 w768] -> w619
                frame False {
                }
                frame True {
                  n1320 = Reverse 1D Array(array=w775) -> (reversed array=w774:i64[])
                  n1321 = Delete From Array(array=w774, index=0) -> (deleted portion=w770:i64, array with subset deleted=w769:i64[])  [unwired: 1 in]
                  n1322 = Reverse 1D Array(array=w769) -> (reversed array=w768:i64[])
                  n1323 = Index Array(array=w766, index (col)=0 ("disabled index (col)")) -> (element=w771:i64[])  [unwired: 1 in]
                  n1324 = Search 1D Array(1D array=w771, element=w770) -> (index of element=w767:i32)  [unwired: 1 in]
                  n1325 = local write "Undo"(FALSE ("Undo")) -> ()
                  n1326 = Delete From Array(array=w766, index (row)=w767) -> (array with subset deleted=w765:i64[][])  [unwired: 2 in, 1 out]
                }
              }
              "last saved data" <- w619
              n1327 = call <vilib>:"Trim Whitespace.vi"("string"="Player 1") -> ("trimmed string"=w598:string)  [unwired: 1 in]
              n1328 = call <vilib>:"Trim Whitespace.vi"("string"="Player 2") -> ("trimmed string"=w595:string)  [unwired: 1 in]
              n1329 = Empty String/Path?(string/path=w598) -> (empty?=w599:bool)
              n1330 = Empty String/Path?(string/path=w595) -> (empty?=w594:bool)
              n1331 = Select(t="Player 1", s=w599, f=w598) -> (s? t:f=w592:string)
              n1332 = Select(t="Player 2", s=w594, f=w595) -> (s? t:f=w591:string)
              n1333 = Concatenate Strings(w592, w586, w591, w586, "Btn 1", w586, "Btn 2", w586, "Btn 3", w586, "Btn 4", w586, "Btn 5", w586, "Game1" ("t"), w586, "Game2" ("t"), w586, "Game3" ("t"), w586, "Game4" ("t"), w586, "Game5" ("t")) -> (w654:string)
              n1334 = for {
                tunnel: string[] ["frame number", "Lead", "Lag", "position 1", "position 2", "position 3", "position 4", "position 5", "position 6", "position 7", "position 8", "position 9", "position 10", "position 11", "position 12", "position 13", "position 14", "position 15", "position 16", "position 17", "position 18", "position 19", "position 20", "position 21", "position 22", "position 23", "position 24", "Drive A", "Drive D", "SW Drive A", "SW Drive D", "drop", "chop", "lob", "boast 2", "boast 3", "kill", "Forehand", "Backhand", "Straight", "Cross", "Bounce", "Half Volley", "Volley", "Expected winner 1", "Expected winner 2", "Unexpected winner 1", "Unexpected winner 2", "Stroke 1", "Stroke 2", "Forced error 1", "Forced error 2", "Unforced error 1", "Unforced error 2", "No let 1", "No let 2", "Let", "point1", "point2", "score1", "score2", "service1", "service2", "s1", "s2", "s3", "s4", "s5", "s6"] ("all rows") -> [w779] mode=indexing
                tunnel: [w777] -> w641 mode=indexing
                n1335 = Concatenate Strings(w779, "\t") -> (w777:string)
              }
              n1336 = local read "Video file"() -> (w611:path)
              n1337 = Index Array(array=w616, index (col)=0 ("disabled index (col)")) -> (element=w691:i64[])  [unwired: 1 in]
              n1338 = Index Array(array=w616, index (col) #1=57 ("disabled index (col)"), index (col) #2=58 ("index (col)")) -> (element #1=w603:i64[], element #2=w602:i64[])  [unwired: 2 in]
              n1339 = local read "Data file"() -> (w607:path)
              n1340 = Array Max & Min(array=w691) -> (max index (indices)=w692:i32)  [unwired: 3 out]
              n1341 = Add Array Elements(numeric array=w603) -> (sum=→"P1":i64)
              n1342 = Add Array Elements(numeric array=w602) -> (sum=→"P2":i64)
              n1343 = call <vilib>:"Get File Extension.vi"("file"=w611) -> ("filename without extension"=w613:string)  [unwired: 7 in, 3 out]
              n1344 = Open/Create/Replace File(file path (use dialog)=w607, operation (0:open)=T4."replace") -> (refnum out=w609:refnum<file>, error out=w608:errorcluster)  [unwired: 4 in, 1 out]
              n1345 = Index Array(array=w616, index (row)=w692) -> (element=→"last row":i64[])  [unwired: 1 in]
              n1346 = Concatenate Strings(w641, w654, "\r") -> (w665:string)
              n1347 = Array To Spreadsheet String(delimiter (Tab)="\t" ("delimiter (\\t)"), array=w616, 3:"%.3f" ("format (%.3f)")) -> (spreadsheet string=w668:string)
              n1348 = Concatenate Strings("avi file" ("string"), w614, w613, w614, w614, w665, w668) -> (w615:string)
              n1349 = Write to Text File(file (use dialog)=w609, text=w615, error in=w608) -> (refnum out=w606:refnum<file>, error out=w605:errorcluster)  [unwired: 1 in, 1 out]
              n1350 = Close File(refnum=w606, error in=w605) -> ()  [unwired: 2 out]
            }
          }
          "coding" <- w404
        }
        frame "Display" {
          n1351 = flat-sequence {
            tunnel: [w1573] -> w1539
            tunnel: w1536 -> [w1574]
            tunnel: w1539 -> [w1594]
            tunnel: [w1593] -> w1535
            tunnel: [w1592] -> w1533
            tunnel: [w1591] -> w1532
            tunnel: w1535 -> [w1689]
            tunnel: [w1689] -> w1534
            tunnel: w1533 -> [w1687]
            tunnel: w1532 -> [w1688]
            tunnel: [w1688] -> w1531
            tunnel: [w1687] -> w1530
            tunnel: [w1713] -> w1538
            tunnel: w1534 -> [w1714]
            tunnel: w1531 -> [w1713]
            tunnel: w1530 -> [w1712]
            tunnel: [w1712] -> w1529
            tunnel: [w1712] -> w1528
            tunnel: w1538 -> [w1768]
            tunnel: [w1768] -> w1537
            tunnel: w1529 -> [_]
            tunnel: w1528 -> [w1757]
            tunnel: [w1757] -> w1527
            tunnel: w1537 -> [w1781]
            tunnel: w1527 -> [w1778]
            frame #0 {
              n1352 = case shown="\"2\"" "display\nselection" {
                tunnel: [w1575 w1577] -> w1573
                tunnel: w1574 -> [w1575 _]
                tunnel: [w1575 w1576] -> _
                frame "1", Default {
                }
                frame "2" {
                  n1353 = local read "EVENTS\nTO PLAY"() -> (w1578:i32[])
                  n1354 = local read "Combined data"() -> (w1580:i64[][])
                  n1355 = for {
                    tunnel: w1580 -> [w1585]
                    tunnel: w1578 -> [w1586] mode=indexing
                    shift-right: [w1587] -> w1577
                    shift-left: i64[][] [] ("Combined data") -> [w1588]
                    i -> [w1582]
                    n1356 = Add(x=w1582, y="before n after") -> (x+y=w1581:i32)
                    n1357 = Index Array(array=w1585, index (row)=w1581) -> (element=w1590:i64[])  [unwired: 1 in]
                    n1358 = Not Equal To 0?(x=w1586) -> (x != 0?=w1584:bool)
                    n1359 = Insert Into Array(array=w1588, new element=w1590) -> (w1589:i64[][])  [unwired: 2 in]
                    n1360 = Select(t=w1589, s=w1584, f=w1588) -> (s? t:f=w1587:i64[][])
                  }
                  n1361 = local read "Edited data"() -> (w1576:i64[][])
                }
              }
            }
            frame #1 {
              w1603 = 64
              # "disreagard player on display option to be set here"
              # "ADD elements on one column to get the data"
              # "extract seperate data sets for player 1 and player 2"
              n1362 = Index Array(array=w1594, index (col)=69 ("index")) -> (element=w1596:i64[])  [unwired: 1 in]
              n1363 = Index Array(array=w1594, index (col)=70 ("index")) -> (element=w1599:i64[])  [unwired: 1 in]
              n1364 = for {
                tunnel: w1594 -> [w1632]
                tunnel: w1596 -> [w1634] mode=indexing
                shift-right: [w1627] -> w1601
                shift-left: i64[][] [] ("Combined data") -> [w1628]
                i -> [w1631]
                n1365 = Index Array(array=w1632, index (row)=w1631) -> (element=w1630:i64[])  [unwired: 1 in]
                n1366 = Not Equal To 0?(x=w1634) -> (x != 0?=w1633:bool)
                n1367 = Insert Into Array(array=w1628, new element=w1630) -> (w1629:i64[][])  [unwired: 2 in]
                n1368 = Select(t=w1629, s=w1633, f=w1628) -> (s? t:f=w1627:i64[][])
              }
              n1369 = for {
                tunnel: w1594 -> [w1624]
                tunnel: w1599 -> [w1626] mode=indexing
                shift-right: [w1619] -> w1602
                shift-left: i64[][] [] ("Combined data") -> [w1620]
                i -> [w1623]
                n1370 = Index Array(array=w1624, index (row)=w1623) -> (element=w1622:i64[])  [unwired: 1 in]
                n1371 = Not Equal To 0?(x=w1626) -> (x != 0?=w1625:bool)
                n1372 = Insert Into Array(array=w1620, new element=w1622) -> (w1621:i64[][])  [unwired: 2 in]
                n1373 = Select(t=w1621, s=w1625, f=w1620) -> (s? t:f=w1619:i64[][])
              }
              n1374 = for {
                N: w1603 -> [_]
                tunnel: w1602 -> [w1612]
                tunnel: [w1609] -> w1592 mode=indexing
                i -> [w1613]
                n1375 = Increment(x=w1613) -> (x+1=w1611:i32)
                n1376 = Index Array(array=w1612, index (col)=w1611) -> (element=w1610:i64[])  [unwired: 1 in]
                n1377 = Add Array Elements(numeric array=w1610) -> (sum=w1609:i64)
              }
              "Player 2 data" <- w1592
              n1378 = for {
                N: w1603 -> [_]
                tunnel: w1601 -> [w1617]
                tunnel: [w1614] -> w1591 mode=indexing
                i -> [w1618]
                n1379 = Increment(x=w1618) -> (x+1=w1616:i32)
                n1380 = Index Array(array=w1617, index (col)=w1616) -> (element=w1615:i64[])  [unwired: 1 in]
                n1381 = Add Array Elements(numeric array=w1615) -> (sum=w1614:i64)
              }
              "player 1 data" <- w1591
              n1382 = for {
                N: w1603 -> [_]
                tunnel: w1594 -> [w1607]
                tunnel: [w1604] -> w1593 mode=indexing
                i -> [w1608]
                n1383 = Increment(x=w1608) -> (x+1=w1606:i32)
                n1384 = Index Array(array=w1607, index (col)=w1606) -> (element=w1605:i64[])  [unwired: 1 in]
                n1385 = Add Array Elements(numeric array=w1605) -> (sum=w1604:i64)
              }
              "both player data" <- w1593
            }
            frame #2 {
              # "Position numbers"
              n1386 = Array Subset(array=w1688, index=2, length=26) -> (w1686:i64[])
              n1387 = for {
                tunnel: w1686 -> [w1703] mode=indexing
                tunnel: [w1699] -> w1685 mode=indexing
                n1388 = Equal To 0?(x=w1703) -> (x = 0?=w1701:bool)
                n1389 = Number To Decimal String(number=w1703) -> (decimal integer string=w1702:string)  [unwired: 1 in]
                n1390 = Select(t="", s=w1701, f=w1702) -> (s? t:f=w1699:string)
              }
              n1391 = Index Array(array=w1685) -> (element #1=→"1 60":string, element #2=→"1 59":string, element #3=→"1 58":string, element #4=→"1 57":string, element #5=→"1 56":string, element #6=→"1 55":string, element #7=→"1 54":string, element #8=→"1 53":string, element #9=→"1 52":string, element #10=→"1 51":string, element #11=→"1 50":string, element #12=→"1 49":string, element #13=→"1 48":string, element #14=→"1 47":string, element #15=→"1 46":string, element #16=→"1 45":string, element #17=→"1 44":string, element #18=→"1 43":string, element #19=→"1 41":string, element #20=→"1 40":string, element #21=→"1 39":string, element #22=→"1 38":string, element #23=→"1 37":string, element #24=→"1 36":string)  [unwired: 24 in]
              n1392 = Array Subset(array=w1687, index=2, length=26) -> (w1660:i64[])
              n1393 = for {
                tunnel: w1660 -> [w1698] mode=indexing
                tunnel: [w1694] -> w1659 mode=indexing
                n1394 = Equal To 0?(x=w1698) -> (x = 0?=w1696:bool)
                n1395 = Number To Decimal String(number=w1698) -> (decimal integer string=w1697:string)  [unwired: 1 in]
                n1396 = Select(t="", s=w1696, f=w1697) -> (s? t:f=w1694:string)
              }
              n1397 = Index Array(array=w1659) -> (element #1=→"1 9":string, element #2=→"1 11":string, element #3=→"1 12":string, element #4=→"1 13":string, element #5=→"1 8":string, element #6=→"1 15":string, element #7=→"1 16":string, element #8=→"1 17":string, element #9=→"1 18":string, element #10=→"1 19":string, element #11=→"1 20":string, element #12=→"1 21":string, element #13=→"1 23":string, element #14=→"1 24":string, element #15=→"1 25":string, element #16=→"1 26":string, element #17=→"1 27":string, element #18=→"1 28":string, element #19=→"1 29":string, element #20=→"1 30":string, element #21=→"1 31":string, element #22=→"1 33":string, element #23=→"1 34":string, element #24=→"1 35":string)  [unwired: 24 in]
            }
            frame #3 {
              # "winner error numbers"
              # "Shot numbers"
              n1398 = Array Subset(array=w1712, index=26, length=10) -> (w1731:i64[])
              n1399 = Index Array(array=w1712, index=55) -> (element=w1721:i64)
              n1400 = Index Array(array=w1713, index=55) -> (element=w1718:i64)
              n1401 = Array Subset(array=w1713, index=26, length=10) -> (w1732:i64[])
              n1402 = Number To Fractional String(number=w1731, precision (6)=i16 0) -> (F-format string=w1705:string[])  [unwired: 2 in]
              n1403 = Array Subset(array=w1714, index=43, length=12) -> (w1738:i64[])
              n1404 = Number To Fractional String(number=w1721, precision (6)=i16 0) -> (F-format string=→"Let 4":string)  [unwired: 2 in]
              n1405 = Number To Fractional String(number=w1732, precision (6)=i16 0) -> (F-format string=w1711:string[])  [unwired: 2 in]
              n1406 = Number To Fractional String(number=w1718, precision (6)=i16 0) -> (F-format string=→"Let 3":string)  [unwired: 2 in]
              n1407 = Number To Fractional String(number=w1738, precision (6)=i16 0) -> (F-format string=w1737:string[])  [unwired: 2 in]
              n1408 = Delete From Array(array=w1705, length=3, index=1) -> (array with subset deleted=→"Player 2 shots numbers":string[])  [unwired: 1 out]
              n1409 = Delete From Array(array=w1711, length=3, index=1) -> (array with subset deleted=→"Player 1 shots numbers":string[])  [unwired: 1 out]
              n1410 = Index Array(array=w1737) -> (element #1=→"ex win1 num":string, element #2=→"ex win2 num":string, element #3=→"UNex win1 num":string, element #4=→"UNex win2 num":string, element #5=→"Stroke 3":string, element #6=→"Stroke 4":string, element #7=→"F err1 num":string, element #8=→"F err2 num":string, element #9=→"UF err1 num":string, element #10=→"UF err2 num":string, element #11=→"No Let 1":string, element #12=→"No Let 2":string)  [unwired: 12 in]
            }
            frame #4 {
              n1411 = Array Subset(array=w1768, index=36, length=7) -> (w1770:i64[])
              n1412 = Array Subset(array=w1757, index=36, length=7) -> (w1761:i64[])
              n1413 = Number To Fractional String(number=w1770, precision (6)=i16 0) -> (F-format string=w1769:string[])  [unwired: 2 in]
              n1414 = Number To Fractional String(number=w1761, precision (6)=i16 0) -> (F-format string=w1762:string[])  [unwired: 2 in]
              n1415 = Index Array(array=w1769) -> (element #1=→"F-hand 1":string, element #2=→"B-hand 1":string, element #3=→"Straight 1":string, element #4=→"Cross 1":string, element #5=→"Bounce 1":string, element #6=→"H-volley 1":string, element #7=→"Volley 1":string)  [unwired: 7 in]
              n1416 = Index Array(array=w1762) -> (element #1=→"F-hand 2":string, element #2=→"B-hand 2":string, element #3=→"Straight 3":string, element #4=→"Cross 3":string, element #5=→"Bounce 3":string, element #6=→"H-volley 3":string, element #7=→"Volley 3":string)  [unwired: 7 in]
            }
            frame #5 {
              # "slider sclaes for graphical display"
              n1417 = Array Subset(array=w1781, index=26, length=10) -> (w1777:i64[])
              n1418 = Array Subset(array=w1778, index=26, length=10) -> (w1776:i64[])
              n1419 = Insert Into Array(array=w1777, new element=w1776) -> (w1775:i64[])  [unwired: 1 in]
              n1420 = Array Max & Min(array=w1776) -> (max value=w1785:i64)  [unwired: 3 out]
              n1421 = Equal To 0?(x=w1785) -> (x = 0?=w1784:bool)
              n1422 = Array Max & Min(array=w1775) -> (max value=w1789:i64)  [unwired: 3 out]
              n1423 = Select(t=1.0, s=w1784, f=w1785) -> ()  [unwired: 1 out]
              n1424 = Equal To 0?(x=w1789) -> (x = 0?=w1788:bool)
              n1425 = Select(t=1.0, s=w1788, f=w1789) -> (s? t:f=w1774:dbl)
              n1426 = property on="FH 2" class="Slide (strict)"("Scale.Maximum"=w1774) -> ()  [unwired: 2 in, 2 out]
              n1427 = property on="BH 2" class="Slide (strict)"("Scale.Maximum"=w1774) -> ()  [unwired: 2 in, 2 out]
              n1428 = property on="Straight 2" class="Slide (strict)"("Scale.Maximum"=w1774) -> ()  [unwired: 2 in, 2 out]
              n1429 = property on="Cross 2" class="Slide (strict)"("Scale.Maximum"=w1774) -> ()  [unwired: 2 in, 2 out]
              n1430 = property on="Bounce 2" class="Slide (strict)"("Scale.Maximum"=w1774) -> ()  [unwired: 2 in, 2 out]
              n1431 = property on="Volley 2" class="Slide (strict)"("Scale.Maximum"=w1774) -> ()  [unwired: 2 in, 2 out]
              n1432 = property on="Drive 2" class="Slide (strict)"("Scale.Maximum"=w1774) -> ()  [unwired: 2 in, 2 out]
              n1433 = property on="Drop 13" class="Slide (strict)"("Scale.Maximum"=w1774) -> ()  [unwired: 2 in, 2 out]
              n1434 = property on="Lob 2" class="Slide (strict)"("Scale.Maximum"=w1774) -> ()  [unwired: 2 in, 2 out]
              n1435 = property on="Boast 13" class="Slide (strict)"("Scale.Maximum"=w1774) -> ()  [unwired: 2 in, 2 out]
              n1436 = property on="Drive 1" class="Slide (strict)"("Scale.Maximum"=w1774) -> ()  [unwired: 2 in, 2 out]
              n1437 = property on="Drop 1" class="Slide (strict)"("Scale.Maximum"=w1774) -> ()  [unwired: 2 in, 2 out]
              n1438 = property on="Lob 1" class="Slide (strict)"("Scale.Maximum"=w1774) -> ()  [unwired: 2 in, 2 out]
              n1439 = property on="Boast 1" class="Slide (strict)"("Scale.Maximum"=w1774) -> ()  [unwired: 2 in, 2 out]
              n1440 = property on="FH 1" class="Slide (strict)"("Scale.Maximum"=w1774) -> ()  [unwired: 2 in, 2 out]
              n1441 = property on="BH 1" class="Slide (strict)"("Scale.Maximum"=w1774) -> ()  [unwired: 2 in, 2 out]
              n1442 = property on="Straight 4" class="Slide (strict)"("Scale.Maximum"=w1774) -> ()  [unwired: 2 in, 2 out]
              n1443 = property on="Cross 4" class="Slide (strict)"("Scale.Maximum"=w1774) -> ()  [unwired: 2 in, 2 out]
              n1444 = property on="Bounce 4" class="Slide (strict)"("Scale.Maximum"=w1774) -> ()  [unwired: 2 in, 2 out]
              n1445 = property on="Volley 4" class="Slide (strict)"("Scale.Maximum"=w1774) -> ()  [unwired: 2 in, 2 out]
              n1446 = Index Array(array=w1776) -> (element #1=→"Drive 2":i64, element #2=→"Drop 13":i64, element #3=→"Lob 2":i64, element #4=→"Boast 13":i64, element #5=→"FH 2":i64, element #6=→"BH 2":i64, element #7=→"Straight 2":i64, element #8=→"Cross 2":i64, element #9=→"Bounce 2":i64, element #10=→"Volley 2":i64)  [unwired: 10 in]
              n1447 = Index Array(array=w1777) -> (element #1=→"Drive 1":i64, element #2=→"Drop 1":i64, element #3=→"Lob 1":i64, element #4=→"Boast 1":i64, element #5=→"FH 1":i64, element #6=→"BH 1":i64, element #7=→"Straight 4":i64, element #8=→"Cross 4":i64, element #9=→"Bounce 4":i64, element #10=→"Volley 4":i64)  [unwired: 10 in]
            }
          }
          n1448 = property on="Video files to write" class="Arr (strict)"() -> ("Index Values"=w1522:u32[])  [unwired: 2 in, 2 out]
          n1449 = Index Array(array=w1522) -> (element=w1519:u32)  [unwired: 1 in]
          n1450 = And Array Elements(Boolean array="Delete") -> (logical AND=w1521:bool)
          n1451 = local read "Video files to write"() -> (w1523:string[])
          n1452 = local read "frames to write"() -> (w1524:i64[][])
          n1453 = case shown="False" w1521 {
            tunnel: "Delete" -> [w1555 _]
            tunnel: w1519 -> [w1553 _]
            frame False {
              n1454 = for {
                tunnel: w1555 -> [w1558] mode=indexing
                tunnel: [w1556] -> w1554
                i -> [w1556]
                stop <- w1557 stop-if-true
                n1455 = Not(x=w1558) -> (.not. x?=w1557:bool)
              }
              n1456 = local write "Delete"(bool[] [TRUE, TRUE, TRUE, TRUE, TRUE] ("Array 2")) -> ()
              n1457 = local read "Video files to write"() -> (w1550:string[])
              n1458 = local read "frames to write"() -> (w1548:i64[][])
              n1459 = Add(x=w1554, y=w1553) -> (x+y=w1547:u32)
              n1460 = Delete From Array(array=w1550, index=w1547) -> (array with subset deleted=w1552:string[])  [unwired: 1 in, 1 out]
              n1461 = Delete From Array(array=w1548, index (row)=w1547) -> (array with subset deleted=w1549:i64[][])  [unwired: 2 in, 1 out]
              n1462 = local write "frames to write"(w1549) -> ()
              n1463 = local write "Video files to write"(w1552) -> ()
            }
            frame True {
            }
          }
          n1464 = case shown="True" "Upload edited video" {
            frame False {
            }
            frame True {
              n1465 = flat-sequence {
                frame #0 {
                  n1466 = local read "frames edited"() -> (w1568:i64[])
                  n1467 = local write "Progress..."(u32 0 ("Progress...")) -> ()
                  n1468 = local write "frames 2 play"(w1568) -> ()
                }
                frame #1 {
                  w1570 = FALSE ("stop")
                  w1571 = TRUE ("Play")
                  n1469 = local write "Load video"(w1571) -> ()
                  n1470 = local write "Play"(w1571) -> ()
                  n1471 = local write "stop"(w1570) -> ()
                  n1472 = local write "Upload edited video"(w1570) -> ()
                  n1473 = local write "Pause"(w1570) -> ()
                }
              }
            }
          }
          n1474 = case shown="True" "Add to lib" {
            tunnel: w1524 -> [_ w1563]
            tunnel: w1523 -> [_ w1560]
            frame False {
            }
            frame True {
              n1475 = local read "frames edited"() -> (w1559:i64[])
              n1476 = local write "Add to lib"(FALSE ("Add to lib")) -> ()
              n1477 = Build Array("File name") -> (w1561:string[])
              n1478 = Build Array(w1559) -> (w1564:i64[][])
              n1479 = Insert Into Array(array=w1564, new element=w1563) -> (→"frames to write":i64[][])  [unwired: 2 in]
              n1480 = Insert Into Array(array=w1561, new element=w1560) -> (→"Video files to write":string[])  [unwired: 1 in]
            }
          }
          n1481 = Select(t=T2."Edit video" ("Main tab"), s="Extract data", f=T2."Display" ("Main tab")) -> (s? t:f=w1546:T2)
          n1482 = local write "Code number display"(1 ("Code number")) -> ()
          n1483 = Select(t=T2."Examine coding" ("Main tab"), s="Examine code", f=w1546) -> (s? t:f=w1516:T2)
          n1484 = Select(t=T6."Clear all" ("Main tab"), s="clear all", f=w1516) -> (s? t:f=w1515:T6)
        }
        frame "Clear all" {
          w1810 = FALSE ("player2")
          w1885 = bool[] [FALSE, FALSE, FALSE, FALSE, FALSE, FALSE, FALSE, FALSE, FALSE, FALSE, FALSE, FALSE, FALSE, FALSE, FALSE, FALSE, FALSE, FALSE, FALSE, FALSE, FALSE, FALSE, FALSE, FALSE, FALSE, FALSE, FALSE, FALSE, FALSE, FALSE, FALSE, FALSE, FALSE, FALSE, FALSE, FALSE, FALSE, FALSE, FALSE, FALSE, FALSE, FALSE, FALSE, FALSE, FALSE, FALSE, FALSE, FALSE, FALSE, FALSE, FALSE, FALSE, FALSE, FALSE, FALSE, FALSE, FALSE, FALSE, FALSE, FALSE, FALSE, FALSE, FALSE, FALSE, FALSE, FALSE, FALSE, FALSE, FALSE]  # Last Edit 2
          n1485 = Split 1D Array(array=w1885, index=24) -> (first subarray=w1835:bool[], second subarray=w1836:bool[])
          n1486 = Index Array(array=w1835) -> (element #1=w1834:bool, element #2=w1833:bool, element #3=w1832:bool, element #4=w1831:bool, element #5=w1830:bool, element #6=w1829:bool, element #7=w1828:bool, element #8=w1827:bool, element #9=w1826:bool, element #10=w1825:bool, element #11=w1824:bool, element #12=w1823:bool, element #13=w1822:bool, element #14=w1821:bool, element #15=w1820:bool, element #16=w1819:bool, element #17=w1818:bool, element #18=w1817:bool, element #19=w1816:bool, element #20=w1815:bool, element #21=w1814:bool, element #22=w1813:bool, element #23=w1812:bool, element #24=w1811:bool)  [unwired: 30 in, 6 out]
          n1487 = Split 1D Array(array=w1836, index=30) -> (first subarray=w1837:bool[], second subarray=w1838:bool[])
          n1488 = local write "1 10"(w1834) -> ()
          n1489 = local write "1 7"(w1833) -> ()
          n1490 = local write "1 6"(w1832) -> ()
          n1491 = local write "1 5"(w1831) -> ()
          n1492 = local write "2 10"(w1830) -> ()
          n1493 = local write "2 7"(w1829) -> ()
          n1494 = local write "2 6"(w1828) -> ()
          n1495 = local write "2 5"(w1827) -> ()
          n1496 = local write "3 9"(w1826) -> ()
          n1497 = local write "3 7"(w1825) -> ()
          n1498 = local write "3 6"(w1824) -> ()
          n1499 = local write "3 5"(w1823) -> ()
          n1500 = local write "4 9"(w1822) -> ()
          n1501 = local write "4 7"(w1821) -> ()
          n1502 = local write "4 6"(w1820) -> ()
          n1503 = local write "4 5"(w1819) -> ()
          n1504 = local write "5 8"(w1818) -> ()
          n1505 = local write "5 7"(w1817) -> ()
          n1506 = local write "5 6"(w1816) -> ()
          n1507 = local write "5 5"(w1815) -> ()
          n1508 = local write "6 8"(w1814) -> ()
          n1509 = local write "6 7"(w1813) -> ()
          n1510 = local write "6 6"(w1812) -> ()
          n1511 = local write "6 5"(w1811) -> ()
          n1512 = Index Array(array=w1837) -> (element #1=w1884:bool, element #2=w1883:bool, element #3=w1882:bool, element #4=w1881:bool, element #5=w1880:bool, element #6=w1879:bool, element #7=w1878:bool, element #8=w1877:bool, element #9=w1876:bool, element #10=w1875:bool, element #11=w1874:bool, element #12=w1873:bool, element #13=w1872:bool, element #14=w1871:bool, element #15=w1870:bool, element #16=w1869:bool, element #17=w1868:bool, element #18=w1867:bool, element #19=w1866:bool, element #20=w1865:bool, element #21=w1864:bool, element #22=w1863:bool, element #23=w1862:bool, element #24=w1861:bool, element #25=w1860:bool, element #26=w1859:bool, element #27=w1858:bool, element #28=w1857:bool, element #29=w1856:bool, element #30=w1855:bool)  [unwired: 30 in]
          n1513 = local write "Adrive"(w1884) -> ()
          n1514 = local write "Ddrive"(w1883) -> ()
          n1515 = local write "ASWdrive"(w1882) -> ()
          n1516 = local write "DSWdrive"(w1881) -> ()
          n1517 = local write "Drop 14"(w1880) -> ()
          n1518 = local write "Chop 13"(w1879) -> ()
          n1519 = local write "Lob"(w1878) -> ()
          n1520 = local write "Boast2"(w1877) -> ()
          n1521 = local write "Boast3"(w1876) -> ()
          n1522 = local write "Smash 13"(w1875) -> ()
          n1523 = local write "FH"(w1874) -> ()
          n1524 = local write "BH"(w1873) -> ()
          n1525 = local write "ST"(w1872) -> ()
          n1526 = local write "CR"(w1871) -> ()
          n1527 = local write "Bounce"(w1870) -> ()
          n1528 = local write "Half Volley"(w1869) -> ()
          n1529 = local write "Volley"(w1868) -> ()
          n1530 = local write "Expected Winner1 2"(w1867) -> ()
          n1531 = local write "Expected Winner2 2"(w1866) -> ()
          n1532 = local write "Unexpected Winner1 2"(w1865) -> ()
          n1533 = local write "Unexpected Winner2 2"(w1864) -> ()
          n1534 = local write "Stroke1 2"(w1863) -> ()
          n1535 = local write "Stroke2 2"(w1862) -> ()
          n1536 = local write "Forced Error1 2"(w1861) -> ()
          n1537 = local write "Forced Error2 2"(w1860) -> ()
          n1538 = local write "Unforced Error1 2"(w1859) -> ()
          n1539 = local write "Unforced Error2 2"(w1858) -> ()
          n1540 = local write "Nolet1 2"(w1857) -> ()
          n1541 = local write "Nolet2 2"(w1856) -> ()
          n1542 = local write "Let 2"(w1855) -> ()
          n1543 = local write "clear all"(FALSE ("clear all")) -> ()
          n1544 = Index Array(array=w1838) -> (element #1=w1854:bool, element #2=w1853:bool, element #3=w1852:bool, element #4=w1851:bool, element #5=w1850:bool, element #6=w1849:bool, element #7=w1848:bool, element #8=w1847:bool, element #9=w1846:bool, element #10=w1845:bool, element #11=w1844:bool, element #12=w1843:bool, element #13=w1842:bool, element #14=w1841:bool, element #15=w1840:bool)  [unwired: 15 in]
          n1545 = local write "Service1 2"(w1854) -> ()
          n1546 = local write "Service2 2"(w1853) -> ()
          n1547 = local write "S1 2"(w1852) -> ()
          n1548 = local write "S2 2"(w1851) -> ()
          n1549 = local write "S3 2"(w1850) -> ()
          n1550 = local write "S4 2"(w1849) -> ()
          n1551 = local write "S5 2"(w1848) -> ()
          n1552 = local write "S6 2"(w1847) -> ()
          n1553 = local write "Player1 2"(w1846) -> ()
          n1554 = local write "Player2 2"(w1845) -> ()
          n1555 = local write "Button 6"(w1844) -> ()
          n1556 = local write "Button 7"(w1843) -> ()
          n1557 = local write "Button 8"(w1842) -> ()
          n1558 = local write "Button 9"(w1841) -> ()
          n1559 = local write "Button 10"(w1840) -> ()
          n1560 = local write "G5"(w1810) -> ()
          n1561 = local write "G4"(w1810) -> ()
          n1562 = local write "G1"(w1810) -> ()
          n1563 = local write "G2"(w1810) -> ()
          n1564 = local write "G3"(w1810) -> ()
        }
        frame "Edit video" {
          w1913 = T5."Disabled and Grayed Out" ("Disabled")
          n1565 = local read "Btn 5"() -> (w1896:string)
          "Btn 10" <- w1896
          n1566 = local read "Btn 4"() -> (w1895:string)
          "Btn 9" <- w1895
          n1567 = local read "Btn 3"() -> (w1894:string)
          "Btn 8" <- w1894
          n1568 = local read "Btn 2"() -> (w1893:string)
          "Btn 7" <- w1893
          n1569 = local read "Btn 1"() -> (w1892:string)
          "Btn 6" <- w1892
          n1570 = local write "before n after"(0 ("before n after")) -> ()
          n1571 = property on="Button 10" class="Bool (strict)"("BoolText.Text"=w1896) -> ()  [unwired: 2 in, 2 out]
          n1572 = property on="Button 9" class="Bool (strict)"("BoolText.Text"=w1895) -> ()  [unwired: 2 in, 2 out]
          n1573 = property on="Button 8" class="Bool (strict)"("BoolText.Text"=w1894) -> ()  [unwired: 2 in, 2 out]
          n1574 = property on="Button 7" class="Bool (strict)"("BoolText.Text"=w1893) -> ()  [unwired: 2 in, 2 out]
          n1575 = property on="Button 6" class="Bool (strict)"("BoolText.Text"=w1892) -> ()  [unwired: 2 in, 2 out]
          n1576 = Array Size(array=w1900) -> (size(s)=w1901:i32[])
          n1577 = Index Array(array=w1901) -> (element #2=w1899:i32)  [unwired: 2 in, 1 out]
          n1578 = Initialize Array(i64 0 ("element"), w1899) -> (w1898:i64[])
          n1579 = local write "Extract data"(FALSE ("edit video")) -> ()
          n1580 = Build Array(w1898) -> (w1897:i64[][])
          n1581 = property on="Code number display" class="DigNum (strict)"("DisabledEnum"=w1913) -> ()  [unwired: 2 in, 2 out]
          n1582 = property on="Next" class="Bool (strict)"("DisabledEnum"=w1913) -> ()  [unwired: 2 in, 2 out]
          n1583 = property on="Reset" class="Bool (strict)"("DisabledEnum"=w1913) -> ()  [unwired: 2 in, 2 out]
          n1584 = property on="Update" class="Bool (strict)"("DisabledEnum"=w1913) -> ()  [unwired: 2 in, 2 out]
          n1585 = property on="Previous" class="Bool (strict)"("DisabledEnum"=w1913) -> ()  [unwired: 2 in, 2 out]
          n1586 = flat-sequence {
            tunnel: [w1934] -> w1903
            tunnel: [w1933] -> w1904
            tunnel: [w1932] -> w1905
            tunnel: [w1931] -> w1906
            tunnel: [w1930] -> w1907
            tunnel: [w1929] -> w1908
            tunnel: [w1928] -> w1909
            tunnel: [w1927] -> w1910
            tunnel: [w1918] -> w1911
            tunnel: [w1923] -> w1912
            tunnel: w1900 -> [w1922]
            tunnel: w1897 -> [w1921]
            tunnel: [w1916] -> w1891
            tunnel: w1912 -> [w1957]
            tunnel: w1911 -> [w2021]
            tunnel: w1910 -> [w2022]
            tunnel: w1909 -> [w1958]
            tunnel: w1908 -> [w2030]
            tunnel: w1907 -> [w2039]
            tunnel: w1906 -> [w2040]
            tunnel: w1905 -> [w2041]
            tunnel: w1904 -> [w2049]
            tunnel: w1903 -> [w2073]
            tunnel: w1891 -> [w1953]
            frame #0 {
              # "seperate sections of data"
              n1587 = Insert Into Array(array=w1921, new element=w1922) -> (w1917:i64[][])  [unwired: 2 in]
              "Combined data" <- w1917
              n1588 = Array Size(array=w1917) -> (size(s)=w1926:i32[])
              n1589 = Index Array(array=w1926) -> (element=w1925:i32)  [unwired: 1 in]
              n1590 = Initialize Array(i64 0 ("element"), w1925) -> (w1923:i64[])
              n1591 = Array Subset(array=w1917, index (col)=3 ("index"), length (col)=24 ("length")) -> (w1934:i64[][])  [unwired: 2 in]
              n1592 = Array Subset(array=w1917, index (col)=27 ("index"), length (col)=10 ("length")) -> (w1933:i64[][])  [unwired: 2 in]
              n1593 = Array Subset(array=w1917, index (col)=37 ("index"), length (col)=2 ("length")) -> (w1932:i64[][])  [unwired: 2 in]
              n1594 = Array Subset(array=w1917, index (col)=39 ("index"), length (col)=2 ("length")) -> (w1931:i64[][])  [unwired: 2 in]
              n1595 = Array Subset(array=w1917, index (col)=41 ("index"), length (col)=3 ("length")) -> (w1930:i64[][])  [unwired: 2 in]
              n1596 = Array Subset(array=w1917, index (col)=44 ("index"), length (col)=13 ("length")) -> (w1929:i64[][])  [unwired: 2 in]
              n1597 = Array Subset(array=w1917, index (col)=61 ("index"), length (col)=8 ("length")) -> (w1928:i64[][])  [unwired: 2 in]
              n1598 = Array Subset(array=w1917, index (col)=69 ("index"), length (col)=2 ("length")) -> (w1927:i64[][])  [unwired: 2 in]
              n1599 = Array Subset(array=w1917, index (col)=71 ("index"), length (col)=5 ("length")) -> (w1918:i64[][])  [unwired: 2 in]
              n1600 = Array Subset(array=w1917, index (col)=76 ("index"), length (col)=5 ("length")) -> (w1916:i64[][])  [unwired: 2 in]
            }
            frame #1 {
              w2103 = i64[][] [] ("Combined data")
              # "AND different sections of data"
              # "extract select events ONLY from full data"
              # "delete negative frames\nand frames past last frame of video"
              n1601 = Build Array("Adrive", "Ddrive", "ASWdrive", "DSWdrive", "Drop 14", "Chop 13", "Lob", "Boast2", "Boast3", "Smash 13") -> (w2001:bool[])
              n1602 = Build Array("1 10", "1 7", "1 6", "1 5", "2 10", "2 7", "2 6", "2 5", "3 9", "3 7", "3 6", "3 5", "4 9", "4 7", "4 6", "4 5", "5 8", "5 7", "5 6", "5 5", "6 8", "6 7", "6 6", "6 5") -> (w2002:bool[])
              n1603 = call "or multiple inputs.vi"("zero array in"=w1957, "input array in"=w2001, "file data in"=w2049) -> ("array out"=w2018:dbl[], "no input?"=w2003:bool)
              n1604 = call "or multiple inputs.vi"("zero array in"=w1957, "input array in"=w2002, "file data in"=w2073) -> ("array out"=w2016:dbl[], "no input?"=w2005:bool)
              n1605 = Build Array("Expected Winner1 2", "Expected Winner2 2", "Unexpected Winner1 2", "Unexpected Winner2 2", "Stroke1 2", "Stroke2 2", "Forced Error1 2", "Forced Error2 2", "Unforced Error1 2", "Unforced Error2 2", "Nolet1 2", "Nolet2 2", "Let 2") -> (w1997:bool[])
              n1606 = call "or multiple inputs.vi"("zero array in"=w1957, "input array in"=w1997, "file data in"=w2030) -> ("array out"=w2017:dbl[], "no input?"=w2004:bool)
              n1607 = Build Array("G1", "G2", "G3", "G4", "G5") -> (w1954:bool[])
              n1608 = Build Array("FH", "BH") -> (w2000:bool[])
              n1609 = Build Array("ST", "CR") -> (w1999:bool[])
              n1610 = Build Array("Bounce", "Half Volley", "Volley") -> (w1998:bool[])
              n1611 = Build Array("Player1 2", "Player2 2") -> (w1995:bool[])
              n1612 = Build Array("Button 6", "Button 7", "Button 8", "Button 9", "Button 10") -> (w1994:bool[])
              n1613 = Build Array("Service1 2", "Service2 2", "S1 2", "S2 2", "S3 2", "S4 2", "S5 2", "S6 2") -> (w1996:bool[])
              n1614 = call "or multiple inputs.vi"("zero array in"=w1957, "input array in"=w2000, "file data in"=w2041) -> ("array out"=w2020:dbl[], "no input?"=w2011:bool)
              n1615 = call "or multiple inputs.vi"("zero array in"=w1957, "input array in"=w1999, "file data in"=w2040) -> ("array out"=w2019:dbl[], "no input?"=w2010:bool)
              n1616 = call "or multiple inputs.vi"("zero array in"=w1957, "input array in"=w1998, "file data in"=w2039) -> ("array out"=w2012:dbl[], "no input?"=w2009:bool)
              n1617 = call "or multiple inputs.vi"("zero array in"=w1957, "input array in"=w1995, "file data in"=w2022) -> ("array out"=w2013:dbl[], "no input?"=w2008:bool)
              n1618 = call "or multiple inputs.vi"("zero array in"=w1957, "input array in"=w1994, "file data in"=w2021) -> ("array out"=w2014:dbl[], "no input?"=w2007:bool)
              n1619 = call "or multiple inputs.vi"("zero array in"=w1957, "input array in"=w1996, "file data in"=w1958) -> ("array out"=w2015:dbl[], "no input?"=w2006:bool)
              n1620 = call "or multiple inputs.vi"("zero array in"=w1957, "input array in"=w1954, "file data in"=w1953) -> ("array out"=w1955:dbl[], "no input?"=w1956:bool)
              n1621 = Compound Arithmetic op=AND(w2020, w2019, w2012, w2013, w2014, w2015, w2016, w2017, w2018, w1955) -> (w2092:i32[])
              "result" <- w2092
              n1622 = Compound Arithmetic op=AND(w2011, w2010, w2009, w2008, w2007, w2006, w2005, w2004, w2003, w1956) -> (w2090:bool)
              n1623 = Select(t=i32[] [] ("result"), s=w2090, f=w2092) -> (s? t:f=w2105:i32[])
              "EVENTS\nTO PLAY" <- w2105
              n1624 = local read "Combined data"() -> (w1985:i64[][])
              n1625 = Insert Into Array(array=w2002, new element #1=w2001, new element #2=w2000, new element #3=w1999, new element #4=w1998, new element #5=w1997, new element #6=w1996, new element #7=w1995, new element #8=w1994, new element #9=w1954) -> (w1993:bool[])  [unwired: 1 in]
              "Last Edit" <- w1993
              n1626 = for {
                tunnel: w1985 -> [w2134]
                tunnel: w2105 -> [w2143] mode=indexing
                shift-right: [w2144] -> w2102
                shift-left: w2103 -> [w2145]
                shift-right: [w2138] -> w2101
                shift-left: w2103 -> [w2139]
                shift-right: [w2131] -> w2100
                shift-left: w2103 -> [w2132]
                i -> [w2136]
                n1627 = Not Equal To 0?(x=w2143) -> (x != 0?=w2130:bool)
                n1628 = Increment(x=w2136) -> (x+1=w2135:i32)
                n1629 = Decrement(x=w2136) -> (x-1=w2142:i32)
                n1630 = Index Array(array=w2134, index (row)=w2136) -> (element=w2147:i64[])  [unwired: 1 in]
                n1631 = Index Array(array=w2134, index (row)=w2135) -> (element=w2137:i64[])  [unwired: 1 in]
                n1632 = Index Array(array=w2134, index (row)=w2142) -> (element=w2141:i64[])  [unwired: 1 in]
                n1633 = Insert Into Array(array=w2132, new element=w2137) -> (w2133:i64[][])  [unwired: 2 in]
                n1634 = Insert Into Array(array=w2145, new element=w2147) -> (w2146:i64[][])  [unwired: 2 in]
                n1635 = Insert Into Array(array=w2139, new element=w2141) -> (w2140:i64[][])  [unwired: 2 in]
                n1636 = Select(t=w2140, s=w2130, f=w2139) -> (s? t:f=w2138:i64[][])
                n1637 = Select(t=w2133, s=w2130, f=w2132) -> (s? t:f=w2131:i64[][])
                n1638 = Select(t=w2146, s=w2130, f=w2145) -> (s? t:f=w2144:i64[][])
              }
              "Edited data" <- w2102
              "Event After" <- w2100
              "Event before" <- w2101
              n1639 = Or Array Elements(Boolean array=w1993) -> (logical OR=w1984:bool)
              n1640 = Index Array(array=w2102, index (col) #1=0 ("disabled index (col)"), index (col) #2=1 ("disabled index (row)"), index (col) #3=2 ("disabled index (col)")) -> (element #1=w2111:i64[], element #2=w1969:i64[], element #3=w1968:i64[])  [unwired: 3 in]
              n1641 = local read "framesPerSecond"() -> (w1967:u32)
              n1642 = Empty Array?(array=w2111) -> (empty?=w1991:bool)
              n1643 = Build Array(w2111) -> (w2099:i64[][])
              n1644 = Array Size(array=w2111) -> (size(s)=w2112:i32)
              n1645 = Transpose 2D Array(2D array=w2099) -> (transposed array=→"edited\nevents":i64[][])
              n1646 = property on="Code number display" class="DigNum (strict)"("Maximum"=w2112, "Minimum"=1.0 ("Data Entry Limits:Minimum")) -> ()  [unwired: 2 in, 2 out]
              n1647 = And(x=w1991, y=w1984) -> (x .and. y?=w1992:bool)
              n1648 = for {
                tunnel: "after" -> [w2150]
                tunnel: w2111 -> [w2169] mode=indexing
                shift-right: [w2163] -> w1983
                shift-left: u32[] [] -> [w2165]
                tunnel: w1969 -> [w2153] mode=indexing
                tunnel: [w2149] -> _ mode=indexing
                tunnel: w1968 -> [w2149] mode=indexing
                tunnel: w1967 -> [w2155]
                tunnel: "before" -> [w2154]
                tunnel: "playback interval on" -> [w2148]
                n1649 = Select(t=w2154, s=w2148, f=w2153) -> (s? t:f=w2152:i64)
                n1650 = Select(t=w2150, s=w2148, f=w2149) -> (s? t:f=w2151:i64)
                n1651 = Multiply(x=w2155, y=w2152) -> (x*y=w2157:i64)
                n1652 = Multiply(x=w2155, y=w2151) -> (x*y=w2156:i64)
                n1653 = Array Max & Min(array=w2165) -> (max value=w2168:u32, max index (indices)=w2164:i32)  [unwired: 2 out]
                n1654 = Subtract(x=w2169, y=w2157) -> (x-y=w2167:i64)
                n1655 = Add(x=w2156, y=w2169) -> (x+y=w2166:i64)
                n1656 = Greater Or Equal?(x=w2168, y=w2167) -> (x >= y?=w2160:bool)
                n1657 = Build Array(w2167, w2166) -> (w2158:i64[])
                n1658 = Build Array(w2166) -> (w2162:i64[])
                n1659 = And(x="Combine", y=w2160) -> (x .and. y?=w2161:bool)
                n1660 = case shown="True" w2161 {
                  tunnel: w2165 -> [w2172 w2176]
                  tunnel: w2164 -> [_ w2175]
                  tunnel: w2162 -> [_ w2174]
                  tunnel: [w2171 w2173] -> w2163
                  tunnel: w2158 -> [w2170 _]
                  frame False {
                    n1661 = Insert Into Array(array=w2172, new element=w2170) -> (w2171:u32[])  [unwired: 1 in]
                  }
                  frame True {
                    n1662 = Replace Array Subset(array=w2176, new element=w2174, index=w2175) -> (w2173:u32[])
                  }
                }
              }
              n1663 = case shown="True" w1992 {
                frame False {
                  n1664 = for {
                    N: 300 -> [_]
                    i -> [w2179]
                    n1665 = Increment(x=w2179) -> (x+1=w2178:i32)
                    n1666 = local write "task"(w2178) -> ()
                    n1667 = Wait (ms)(milliseconds to wait=u32 1) -> ()  [unwired: 1 out]
                  }
                }
                frame True {
                  n1668 = One Button Dialog(message="INVALID EVENTS\n\nSelected event(s) or combination of events does not exist") -> ()  [unwired: 1 in, 1 out]
                }
              }
              n1669 = Delete From Array(array=w1985, length=1, index (col)=0 ("disabled index (col)")) -> (deleted portion=w1990:i64[][])  [unwired: 1 in, 1 out]
              n1670 = Array Max & Min(array=w1990) -> (max value=w1989:i64, min value=w1988:i64)  [unwired: 2 out]
              n1671 = Build Array(w1988, w1989) -> (w1981:i64[])
              n1672 = Select(t=w1983, s=w1984, f=w1981) -> (s? t:f=w1982:i64[])
              "edited to play" <- w1982
              n1673 = Array Size(array=w1982) -> (size(s)=w2094:i32)
              n1674 = Divide(x=w2094, y=2) -> (x/y=w2095:dbl)
              n1675 = for {
                N: w2095 -> [_]
                shift-right: [w2120] -> _
                shift-left: w1982 -> [w2122]
                shift-right: [w2115] -> w2093
                shift-left: i64[] [] ("edited\nto play 3") -> [w2116]
                n1676 = Split 1D Array(array=w2122, index=2) -> (first subarray=w2121:i64[], second subarray=w2120:i64[])
                n1677 = Index Array(array=w2121, index #1=1 ("index"), index #2=0 ("index")) -> (element #1=w2126:i64, element #2=w2119:i64)
                n1678 = Subtract(x=w2126, y=w2119) -> (x-y=w2118:i64)
                n1679 = Increment(x=w2118) -> (x+1=w2117:i64)
                n1680 = for {
                  N: w2117 -> [_]
                  tunnel: w2119 -> [w2129]
                  tunnel: [w2127] -> w2114 mode=indexing
                  tunnel: [w2127] -> _
                  i -> [w2128]
                  n1681 = Add(x=w2129, y=w2128) -> (x+y=w2127:i64)
                }
                n1682 = Insert Into Array(array=w2116, new element=w2114) -> (w2115:i64[])  [unwired: 1 in]
              }
              n1683 = local read "Number of Frames"() -> (w2108:u32)
              n1684 = Subtract(x=w2108, y=u32 2) -> (x-y=w2110:u32)
              n1685 = In Range and Coerce(upper limit=0, x=w2093, lower limit=w2110) -> (coerced(x)=→"frames edited" →"frames 2 play":i64[])  [unwired: 1 out]
            }
          }
        }
        frame "Examine coding" {
          w2264 = T5."Enabled" ("Disabled")
          n1686 = property on="Code number display" class="DigNum (strict)"("DisabledEnum"=w2264) -> ()  [unwired: 2 in, 2 out]
          n1687 = property on="Next" class="Bool (strict)"("DisabledEnum"=w2264) -> ()  [unwired: 2 in, 2 out]
          n1688 = property on="Reset" class="Bool (strict)"("DisabledEnum"=w2264) -> ()  [unwired: 2 in, 2 out]
          n1689 = property on="Update" class="Bool (strict)"("DisabledEnum"=w2264) -> ()  [unwired: 2 in, 2 out]
          n1690 = property on="Previous" class="Bool (strict)"("DisabledEnum"=w2264) -> ()  [unwired: 2 in, 2 out]
          n1691 = local read "edited\nevents"() -> (w2271:i64[][])
          n1692 = Decrement(x="Code number display") -> (x-1=w2265:i32)
          n1693 = flat-sequence {
            tunnel: "Code number display" -> [w2288]
            frame #0 {
              n1694 = local read "edited to play"() -> (w2287:i64[])
              n1695 = for {
                N: w2288 -> [_]
                shift-right: [w2293] -> _
                shift-left: w2287 -> [w2294]
                tunnel: [w2292] -> w2280
                n1696 = Split 1D Array(array=w2294, index=2) -> (first subarray=w2292:i64[], second subarray=w2293:i64[])
              }
              n1697 = Index Array(array=w2280, index #1=1 ("index"), index #2=0 ("index")) -> (element #1=w2286:i64, element #2=w2283:i64)
              n1698 = Subtract(x=w2286, y=w2283) -> (x-y=w2282:i64)
              n1699 = Increment(x=w2282) -> (x+1=w2281:i64)
              n1700 = for {
                N: w2281 -> [_]
                tunnel: w2283 -> [w2291]
                tunnel: [w2289] -> w2279 mode=indexing
                i -> [w2290]
                n1701 = Add(x=w2291, y=w2290) -> (x+y=w2289:i64)
              }
              n1702 = local write "Progress..."(u32 0 ("Progress...")) -> ()
              n1703 = local write "frames 2 play"(w2279) -> ()
            }
            frame #1 {
              w2296 = TRUE ("Play")
              w2297 = FALSE ("Next")
              n1704 = local write "Next"(w2297) -> ()
              n1705 = local write "Previous"(w2297) -> ()
              n1706 = local write "Reset"(w2297) -> ()
              n1707 = local write "stop"(w2297) -> ()
              n1708 = local write "Pause"(w2297) -> ()
              n1709 = local write "Load video"(w2296) -> ()
              n1710 = local write "Play"(w2296) -> ()
            }
          }
          n1711 = Index Array(array=w2271, index (row)=w2265, index (col)=0) -> (element=w2270:i64)
          n1712 = Index Array(array=w2268, index (col)=0 ("disabled index (col)")) -> (element=w2275:i64[])  [unwired: 1 in]
          n1713 = Search 1D Array(1D array=w2275, element=w2270) -> (index of element=w2274:i32)  [unwired: 1 in]
          n1714 = Index Array(array=w2268, index (row)=w2274) -> (element=w2273:i64[])  [unwired: 1 in]
          n1715 = Delete From Array(array=w2273, length=3, index=0) -> (array with subset deleted=w2272:i64[])  [unwired: 1 out]
          n1716 = for {
            tunnel: w2272 -> [w2302] mode=indexing
            tunnel: [w2298] -> w2187 mode=indexing
            n1717 = Equal To 0?(x=w2302) -> (x = 0?=w2301:bool)
            n1718 = Select(t=FALSE ("x = 0?"), s=w2301, f=TRUE) -> (s? t:f=w2298:bool)
          }
          n1719 = Split 1D Array(array=w2187, index=24) -> (first subarray=w2212:bool[], second subarray=w2213:bool[])
          n1720 = Index Array(array=w2212) -> (element #1=w2211:bool, element #2=w2210:bool, element #3=w2209:bool, element #4=w2208:bool, element #5=w2207:bool, element #6=w2206:bool, element #7=w2205:bool, element #8=w2204:bool, element #9=w2203:bool, element #10=w2202:bool, element #11=w2201:bool, element #12=w2200:bool, element #13=w2199:bool, element #14=w2198:bool, element #15=w2197:bool, element #16=w2196:bool, element #17=w2195:bool, element #18=w2194:bool, element #19=w2193:bool, element #20=w2192:bool, element #21=w2191:bool, element #22=w2190:bool, element #23=w2189:bool, element #24=w2188:bool)  [unwired: 30 in, 6 out]
          n1721 = Split 1D Array(array=w2213, index=34) -> (first subarray=w2214:bool[], second subarray=w2215:bool[])
          n1722 = local write "1 10"(w2211) -> ()
          n1723 = local write "1 7"(w2210) -> ()
          n1724 = local write "1 6"(w2209) -> ()
          n1725 = local write "1 5"(w2208) -> ()
          n1726 = local write "2 10"(w2207) -> ()
          n1727 = local write "2 7"(w2206) -> ()
          n1728 = local write "2 6"(w2205) -> ()
          n1729 = local write "2 5"(w2204) -> ()
          n1730 = local write "3 9"(w2203) -> ()
          n1731 = local write "3 7"(w2202) -> ()
          n1732 = local write "3 6"(w2201) -> ()
          n1733 = local write "3 5"(w2200) -> ()
          n1734 = local write "4 9"(w2199) -> ()
          n1735 = local write "4 7"(w2198) -> ()
          n1736 = local write "4 6"(w2197) -> ()
          n1737 = local write "4 5"(w2196) -> ()
          n1738 = local write "5 8"(w2195) -> ()
          n1739 = local write "5 7"(w2194) -> ()
          n1740 = local write "5 6"(w2193) -> ()
          n1741 = local write "5 5"(w2192) -> ()
          n1742 = local write "6 8"(w2191) -> ()
          n1743 = local write "6 7"(w2190) -> ()
          n1744 = local write "6 6"(w2189) -> ()
          n1745 = local write "6 5"(w2188) -> ()
          n1746 = Index Array(array=w2214) -> (element #1=w2261:bool, element #2=w2260:bool, element #3=w2259:bool, element #4=w2258:bool, element #5=w2257:bool, element #6=w2256:bool, element #7=w2255:bool, element #8=w2254:bool, element #9=w2253:bool, element #10=w2252:bool, element #11=w2251:bool, element #12=w2250:bool, element #13=w2249:bool, element #14=w2248:bool, element #15=w2247:bool, element #16=w2246:bool, element #17=w2245:bool, element #18=w2244:bool, element #19=w2243:bool, element #20=w2242:bool, element #21=w2241:bool, element #22=w2240:bool, element #23=w2239:bool, element #24=w2238:bool, element #25=w2237:bool, element #26=w2236:bool, element #27=w2235:bool, element #28=w2234:bool, element #29=w2233:bool, element #30=w2232:bool)  [unwired: 30 in]
          n1747 = local write "Adrive"(w2261) -> ()
          n1748 = local write "Ddrive"(w2260) -> ()
          n1749 = local write "ASWdrive"(w2259) -> ()
          n1750 = local write "DSWdrive"(w2258) -> ()
          n1751 = local write "Drop 14"(w2257) -> ()
          n1752 = local write "Chop 13"(w2256) -> ()
          n1753 = local write "Lob"(w2255) -> ()
          n1754 = local write "Boast2"(w2254) -> ()
          n1755 = local write "Boast3"(w2253) -> ()
          n1756 = local write "Smash 13"(w2252) -> ()
          n1757 = local write "FH"(w2251) -> ()
          n1758 = local write "BH"(w2250) -> ()
          n1759 = local write "ST"(w2249) -> ()
          n1760 = local write "CR"(w2248) -> ()
          n1761 = local write "Bounce"(w2247) -> ()
          n1762 = local write "Half Volley"(w2246) -> ()
          n1763 = local write "Volley"(w2245) -> ()
          n1764 = local write "Expected Winner1 2"(w2244) -> ()
          n1765 = local write "Expected Winner2 2"(w2243) -> ()
          n1766 = local write "Unexpected Winner1 2"(w2242) -> ()
          n1767 = local write "Unexpected Winner2 2"(w2241) -> ()
          n1768 = local write "Stroke1 2"(w2240) -> ()
          n1769 = local write "Stroke2 2"(w2239) -> ()
          n1770 = local write "Forced Error1 2"(w2238) -> ()
          n1771 = local write "Forced Error2 2"(w2237) -> ()
          n1772 = local write "Unforced Error1 2"(w2236) -> ()
          n1773 = local write "Unforced Error2 2"(w2235) -> ()
          n1774 = local write "Nolet1 2"(w2234) -> ()
          n1775 = local write "Nolet2 2"(w2233) -> ()
          n1776 = local write "Let 2"(w2232) -> ()
          n1777 = Index Array(array=w2215) -> (element #1=w2231:bool, element #2=w2230:bool, element #3=w2229:bool, element #4=w2228:bool, element #5=w2227:bool, element #6=w2226:bool, element #7=w2225:bool, element #8=w2224:bool, element #9=w2223:bool, element #10=w2222:bool, element #11=w2221:bool, element #12=w2220:bool, element #13=w2219:bool, element #14=w2218:bool, element #15=w2217:bool, element #16=w2186:bool, element #17=w2185:bool, element #18=w2184:bool, element #19=w2183:bool, element #20=w2182:bool)  [unwired: 20 in]
          n1778 = local write "Service1 2"(w2231) -> ()
          n1779 = local write "Service2 2"(w2230) -> ()
          n1780 = local write "S1 2"(w2229) -> ()
          n1781 = local write "S2 2"(w2228) -> ()
          n1782 = local write "S3 2"(w2227) -> ()
          n1783 = local write "S4 2"(w2226) -> ()
          n1784 = local write "S5 2"(w2225) -> ()
          n1785 = local write "S6 2"(w2224) -> ()
          n1786 = local write "Player1 2"(w2223) -> ()
          n1787 = local write "Player2 2"(w2222) -> ()
          n1788 = local write "Button 6"(w2221) -> ()
          n1789 = local write "Button 7"(w2220) -> ()
          n1790 = local write "Button 8"(w2219) -> ()
          n1791 = local write "Button 9"(w2218) -> ()
          n1792 = local write "Button 10"(w2217) -> ()
          n1793 = local write "G1"(w2186) -> ()
          n1794 = local write "G2"(w2185) -> ()
          n1795 = local write "G3"(w2184) -> ()
          n1796 = local write "G4"(w2183) -> ()
          n1797 = local write "G5"(w2182) -> ()
        }
        frame "Edit coding" {
          n1798 = local read "Examine code"() -> (w2303:bool)
          n1799 = case shown="True" w2303 {
            tunnel: [T2."Edit video" ("Main tab") w2391] -> w2305
            frame False {
              n1800 = local read "Last Edit"() -> (w2385:bool[])
              n1801 = Split 1D Array(array=w2385, index=24) -> (first subarray=w2335:bool[], second subarray=w2336:bool[])
              n1802 = Index Array(array=w2335) -> (element #1=w2334:bool, element #2=w2333:bool, element #3=w2332:bool, element #4=w2331:bool, element #5=w2330:bool, element #6=w2329:bool, element #7=w2328:bool, element #8=w2327:bool, element #9=w2326:bool, element #10=w2325:bool, element #11=w2324:bool, element #12=w2323:bool, element #13=w2322:bool, element #14=w2321:bool, element #15=w2320:bool, element #16=w2319:bool, element #17=w2318:bool, element #18=w2317:bool, element #19=w2316:bool, element #20=w2315:bool, element #21=w2314:bool, element #22=w2313:bool, element #23=w2312:bool, element #24=w2311:bool)  [unwired: 30 in, 6 out]
              n1803 = Split 1D Array(array=w2336, index=30) -> (first subarray=w2337:bool[], second subarray=w2338:bool[])
              n1804 = local write "1 10"(w2334) -> ()
              n1805 = local write "1 7"(w2333) -> ()
              n1806 = local write "1 6"(w2332) -> ()
              n1807 = local write "1 5"(w2331) -> ()
              n1808 = local write "2 10"(w2330) -> ()
              n1809 = local write "2 7"(w2329) -> ()
              n1810 = local write "2 6"(w2328) -> ()
              n1811 = local write "2 5"(w2327) -> ()
              n1812 = local write "3 9"(w2326) -> ()
              n1813 = local write "3 7"(w2325) -> ()
              n1814 = local write "3 6"(w2324) -> ()
              n1815 = local write "3 5"(w2323) -> ()
              n1816 = local write "4 9"(w2322) -> ()
              n1817 = local write "4 7"(w2321) -> ()
              n1818 = local write "4 6"(w2320) -> ()
              n1819 = local write "4 5"(w2319) -> ()
              n1820 = local write "5 8"(w2318) -> ()
              n1821 = local write "5 7"(w2317) -> ()
              n1822 = local write "5 6"(w2316) -> ()
              n1823 = local write "5 5"(w2315) -> ()
              n1824 = local write "6 8"(w2314) -> ()
              n1825 = local write "6 7"(w2313) -> ()
              n1826 = local write "6 6"(w2312) -> ()
              n1827 = local write "6 5"(w2311) -> ()
              n1828 = Index Array(array=w2337) -> (element #1=w2384:bool, element #2=w2383:bool, element #3=w2382:bool, element #4=w2381:bool, element #5=w2380:bool, element #6=w2379:bool, element #7=w2378:bool, element #8=w2377:bool, element #9=w2376:bool, element #10=w2375:bool, element #11=w2374:bool, element #12=w2373:bool, element #13=w2372:bool, element #14=w2371:bool, element #15=w2370:bool, element #16=w2369:bool, element #17=w2368:bool, element #18=w2367:bool, element #19=w2366:bool, element #20=w2365:bool, element #21=w2364:bool, element #22=w2363:bool, element #23=w2362:bool, element #24=w2361:bool, element #25=w2360:bool, element #26=w2359:bool, element #27=w2358:bool, element #28=w2357:bool, element #29=w2356:bool, element #30=w2355:bool)  [unwired: 30 in]
              n1829 = local write "Adrive"(w2384) -> ()
              n1830 = local write "Ddrive"(w2383) -> ()
              n1831 = local write "ASWdrive"(w2382) -> ()
              n1832 = local write "DSWdrive"(w2381) -> ()
              n1833 = local write "Drop 14"(w2380) -> ()
              n1834 = local write "Chop 13"(w2379) -> ()
              n1835 = local write "Lob"(w2378) -> ()
              n1836 = local write "Boast2"(w2377) -> ()
              n1837 = local write "Boast3"(w2376) -> ()
              n1838 = local write "Smash 13"(w2375) -> ()
              n1839 = local write "FH"(w2374) -> ()
              n1840 = local write "BH"(w2373) -> ()
              n1841 = local write "ST"(w2372) -> ()
              n1842 = local write "CR"(w2371) -> ()
              n1843 = local write "Bounce"(w2370) -> ()
              n1844 = local write "Half Volley"(w2369) -> ()
              n1845 = local write "Volley"(w2368) -> ()
              n1846 = local write "Expected Winner1 2"(w2367) -> ()
              n1847 = local write "Expected Winner2 2"(w2366) -> ()
              n1848 = local write "Unexpected Winner1 2"(w2365) -> ()
              n1849 = local write "Unexpected Winner2 2"(w2364) -> ()
              n1850 = local write "Stroke1 2"(w2363) -> ()
              n1851 = local write "Stroke2 2"(w2362) -> ()
              n1852 = local write "Forced Error1 2"(w2361) -> ()
              n1853 = local write "Forced Error2 2"(w2360) -> ()
              n1854 = local write "Unforced Error1 2"(w2359) -> ()
              n1855 = local write "Unforced Error2 2"(w2358) -> ()
              n1856 = local write "Nolet1 2"(w2357) -> ()
              n1857 = local write "Nolet2 2"(w2356) -> ()
              n1858 = local write "Let 2"(w2355) -> ()
              n1859 = Index Array(array=w2338) -> (element #1=w2354:bool, element #2=w2353:bool, element #3=w2352:bool, element #4=w2351:bool, element #5=w2350:bool, element #6=w2349:bool, element #7=w2348:bool, element #8=w2347:bool, element #9=w2346:bool, element #10=w2345:bool, element #11=w2344:bool, element #12=w2343:bool, element #13=w2342:bool, element #14=w2341:bool, element #15=w2340:bool, element #16=w2310:bool, element #17=w2309:bool, element #18=w2308:bool, element #19=w2307:bool, element #20=w2306:bool)  [unwired: 20 in]
              n1860 = local write "Upload edited video"(TRUE ("Upload edited video")) -> ()
              n1861 = local write "Service1 2"(w2354) -> ()
              n1862 = local write "Service2 2"(w2353) -> ()
              n1863 = local write "S1 2"(w2352) -> ()
              n1864 = local write "S2 2"(w2351) -> ()
              n1865 = local write "S3 2"(w2350) -> ()
              n1866 = local write "S4 2"(w2349) -> ()
              n1867 = local write "S5 2"(w2348) -> ()
              n1868 = local write "S6 2"(w2347) -> ()
              n1869 = local write "Player1 2"(w2346) -> ()
              n1870 = local write "Player2 2"(w2345) -> ()
              n1871 = local write "Button 6"(w2344) -> ()
              n1872 = local write "Button 7"(w2343) -> ()
              n1873 = local write "Button 8"(w2342) -> ()
              n1874 = local write "Button 9"(w2341) -> ()
              n1875 = local write "Button 10"(w2340) -> ()
              n1876 = local write "G1"(w2310) -> ()
              n1877 = local write "G2"(w2309) -> ()
              n1878 = local write "G3"(w2308) -> ()
              n1879 = local write "G4"(w2307) -> ()
              n1880 = local write "G5"(w2306) -> ()
            }
            frame True {
              n1881 = event shown="[0] Timeout" {
                selector: _ -> [_ _]
                dyn-events: _ -> [_ _]
                timeout: 25 -> [_ _]
                tunnel: [FALSE TRUE] -> w2389
                event Timeout {
                  n1882 = event-data() -> ()  [unwired: 1 in, 3 out]
                }
                event "Code number display": Value Change {
                  n1883 = event-data() -> ()  [unwired: 1 in, 3 out]
                }
              }
              n1884 = case shown="True" "Next" {
                frame False {
                }
                frame True {
                  n1885 = local read "edited\nevents"() -> (w2408:i64[][])
                  n1886 = local read "Code number display"() -> (w2404:i32)
                  n1887 = Index Array(array=w2408, index (col)=0 ("disabled index (col)")) -> (element=w2410:i64[])  [unwired: 1 in]
                  n1888 = Array Size(array=w2410) -> (size(s)=w2403:i32)
                  n1889 = Increment(x=w2404) -> (x+1=w2406:i32)
                  n1890 = Less Or Equal?(x=w2406, y=w2403) -> (x <= y?=w2407:bool)
                  n1891 = Select(t=w2406, s=w2407, f=w2403) -> (s? t:f=w2405:i32)
                  n1892 = local write "Code number display"(w2405) -> ()
                }
              }
              n1893 = case shown="True" "Previous" {
                frame False {
                }
                frame True {
                  n1894 = local read "Code number display"() -> (w2411:i32)
                  n1895 = Decrement(x=w2411) -> (x-1=w2414:i32)
                  n1896 = Greater Than 0?(x=w2414) -> (x > 0?=w2415:bool)
                  n1897 = Select(t=w2414, s=w2415, f=1) -> (s? t:f=w2412:i32)
                  n1898 = local write "Code number display"(w2412) -> ()
                }
              }
              n1899 = Compound Arithmetic op=OR(w2389, "Reset", "Previous", "Next") -> (w2397:bool)
              n1900 = Select(t=T2."Examine coding" ("Main tab"), s=w2397, f=T2."Edit coding" ("Main tab")) -> (s? t:f=w2392:T2)
              n1901 = Select(t=T2."Update coding" ("Main tab"), s="Update", f=w2392) -> (s? t:f=w2391:T2)
            }
          }
        }
        frame "Update coding" {
          w2417 = "\t"
          w2455 = "\r"
          n1902 = flat-sequence {
            tunnel: w2459 -> [w2557]
            tunnel: [w2554] -> w2458
            tunnel: w2458 -> [w2646]
            tunnel: [w2646] -> w2442
            frame #0 {
              w2503 = FALSE
              n1903 = local read "Service1 2"() -> (w2502:bool)
              n1904 = local read "Service2 2"() -> (w2501:bool)
              n1905 = local read "Button 10"() -> (w2488:bool)
              n1906 = local read "Player1 2"() -> (w2494:bool)
              n1907 = local read "Player2 2"() -> (w2493:bool)
              n1908 = local read "Button 6"() -> (w2492:bool)
              n1909 = local read "Button 7"() -> (w2491:bool)
              n1910 = local read "Button 8"() -> (w2490:bool)
              n1911 = local read "Button 9"() -> (w2489:bool)
              n1912 = local read "S1 2"() -> (w2500:bool)
              n1913 = local read "S2 2"() -> (w2499:bool)
              n1914 = local read "S3 2"() -> (w2498:bool)
              n1915 = local read "S4 2"() -> (w2497:bool)
              n1916 = local read "S5 2"() -> (w2496:bool)
              n1917 = local read "S6 2"() -> (w2495:bool)
              n1918 = local read "1 10"() -> (w2551:bool)
              n1919 = local read "2 10"() -> (w2547:bool)
              n1920 = local read "G1"() -> (w2468:bool)
              n1921 = local read "G2"() -> (w2467:bool)
              n1922 = local read "G3"() -> (w2466:bool)
              n1923 = local read "G4"() -> (w2465:bool)
              n1924 = local read "G5"() -> (w2464:bool)
              n1925 = local read "5 8"() -> (w2483:bool)
              n1926 = local read "5 7"() -> (w2482:bool)
              n1927 = local read "5 6"() -> (w2481:bool)
              n1928 = local read "5 5"() -> (w2480:bool)
              n1929 = local read "6 8"() -> (w2479:bool)
              n1930 = local read "6 7"() -> (w2478:bool)
              n1931 = local read "6 6"() -> (w2477:bool)
              n1932 = local read "6 5"() -> (w2476:bool)
              n1933 = local read "1 7"() -> (w2550:bool)
              n1934 = local read "1 6"() -> (w2549:bool)
              n1935 = local read "1 5"() -> (w2548:bool)
              n1936 = local read "2 7"() -> (w2546:bool)
              n1937 = local read "2 6"() -> (w2545:bool)
              n1938 = local read "2 5"() -> (w2544:bool)
              n1939 = local read "3 9"() -> (w2543:bool)
              n1940 = local read "3 7"() -> (w2542:bool)
              n1941 = local read "3 6"() -> (w2541:bool)
              n1942 = local read "3 5"() -> (w2540:bool)
              n1943 = local read "4 9"() -> (w2539:bool)
              n1944 = local read "4 7"() -> (w2538:bool)
              n1945 = local read "4 6"() -> (w2537:bool)
              n1946 = local read "4 5"() -> (w2536:bool)
              n1947 = Build Array(w2502, w2501, w2500, w2499, w2498, w2497, w2496, w2495, w2494, w2493, w2492, w2491, w2490, w2489, w2488, w2468, w2467, w2466, w2465, w2464) -> (w2485:bool[])
              n1948 = Build Array(w2551, w2550, w2549, w2548, w2547, w2546, w2545, w2544, w2543, w2542, w2541, w2540, w2539, w2538, w2537, w2536, w2483, w2482, w2481, w2480, w2479, w2478, w2477, w2476) -> (w2487:bool[])
              n1949 = local read "Unexpected Winner1 2"() -> (w2516:bool)
              n1950 = local read "Unexpected Winner2 2"() -> (w2509:bool)
              n1951 = local read "Expected Winner1 2"() -> (w2517:bool)
              n1952 = local read "Expected Winner2 2"() -> (w2510:bool)
              n1953 = local read "Unforced Error1 2"() -> (w2506:bool)
              n1954 = local read "Unforced Error2 2"() -> (w2513:bool)
              n1955 = local read "Forced Error1 2"() -> (w2507:bool)
              n1956 = local read "Forced Error2 2"() -> (w2514:bool)
              n1957 = local read "ASWdrive"() -> (w2533:bool)
              n1958 = local read "DSWdrive"() -> (w2532:bool)
              n1959 = local read "Smash 13"() -> (w2526:bool)
              n1960 = local read "Stroke1 2"() -> (w2515:bool)
              n1961 = local read "Stroke2 2"() -> (w2508:bool)
              n1962 = local read "Volley"() -> (w2519:bool)
              n1963 = local read "Chop 13"() -> (w2530:bool)
              n1964 = local read "Half Volley"() -> (w2520:bool)
              n1965 = local read "Nolet1 2"() -> (w2505:bool)
              n1966 = local read "Nolet2 2"() -> (w2512:bool)
              n1967 = local read "Drop 14"() -> (w2531:bool)
              n1968 = local read "Bounce"() -> (w2521:bool)
              n1969 = local read "Boast2"() -> (w2528:bool)
              n1970 = local read "Boast3"() -> (w2527:bool)
              n1971 = local read "Adrive"() -> (w2535:bool)
              n1972 = local read "Ddrive"() -> (w2534:bool)
              n1973 = local read "Let 2"() -> (w2518:bool)
              n1974 = local read "Lob"() -> (w2529:bool)
              n1975 = local read "BH"() -> (w2524:bool)
              n1976 = local read "FH"() -> (w2525:bool)
              n1977 = local read "CR"() -> (w2522:bool)
              n1978 = local read "ST"() -> (w2523:bool)
              n1979 = Compound Arithmetic op=OR(w2510, w2509, w2508, w2507, w2506, w2505) -> (w2504:bool)
              n1980 = Compound Arithmetic op=OR(w2517, w2516, w2515, w2514, w2513, w2512) -> (w2511:bool)
              n1981 = Build Array(w2535, w2534, w2533, w2532, w2531, w2530, w2529, w2528, w2527, w2526, w2525, w2524, w2523, w2522, w2521, w2520, w2519, w2517, w2510, w2516, w2509, w2515, w2508, w2507, w2514, w2506, w2513, w2505, w2512, w2518, w2511, w2504, w2503, w2503) -> (w2486:bool[])
              n1982 = Insert Into Array(array=w2487, new element #1=w2486, new element #2=w2485) -> (w2484:bool[])  [unwired: 1 in]
              n1983 = local read "Code number display"() -> (w2553:i32)
              n1984 = Boolean To (0,1)(Boolean=w2484) -> (0, 1=w2558:i16[])
              n1985 = local read "edited\nevents"() -> (w2559:i64[][])
              n1986 = Decrement(x=w2553) -> (x-1=w2552:i32)
              n1987 = Index Array(array=w2557, index (col)=0 ("disabled index (col)")) -> (element=w2562:i64[])  [unwired: 1 in]
              n1988 = Index Array(array=w2559, index (row)=w2552, index (col)=0) -> (element=w2561:i64)
              n1989 = Search 1D Array(1D array=w2562, element=w2561) -> (index of element=w2555:i32)  [unwired: 1 in]
              n1990 = Index Array(array=w2557, index (row)=w2555) -> (element=w2475:i64[])  [unwired: 1 in]
              n1991 = Delete From Array(array=w2475, index=0) -> ()  [unwired: 1 in, 2 out]
              n1992 = Index Array(array=w2475, index #1=0 ("index"), index #2=1 ("index"), index #3=2 ("index")) -> (element #1=w2474:i64, element #2=w2473:i64, element #3=w2472:i64)
              n1993 = Build Array (concatenate)(w2474, w2473, w2472, w2558) -> (w2556:i64[])
              n1994 = Replace Array Subset(array=w2557, new element=w2556, index (row)=w2555) -> (w2554:i64[][])  [unwired: 1 in]
            }
            frame #1 {
              n1995 = local read "Last Edit"() -> (w2644:bool[])
              n1996 = Split 1D Array(array=w2644, index=24) -> (first subarray=w2594:bool[], second subarray=w2595:bool[])
              n1997 = Index Array(array=w2594) -> (element #1=w2593:bool, element #2=w2592:bool, element #3=w2591:bool, element #4=w2590:bool, element #5=w2589:bool, element #6=w2588:bool, element #7=w2587:bool, element #8=w2586:bool, element #9=w2585:bool, element #10=w2584:bool, element #11=w2583:bool, element #12=w2582:bool, element #13=w2581:bool, element #14=w2580:bool, element #15=w2579:bool, element #16=w2578:bool, element #17=w2577:bool, element #18=w2576:bool, element #19=w2575:bool, element #20=w2574:bool, element #21=w2573:bool, element #22=w2572:bool, element #23=w2571:bool, element #24=w2570:bool)  [unwired: 30 in, 6 out]
              n1998 = Split 1D Array(array=w2595, index=30) -> (first subarray=w2596:bool[], second subarray=w2597:bool[])
              n1999 = local write "1 10"(w2593) -> ()
              n2000 = local write "1 7"(w2592) -> ()
              n2001 = local write "1 6"(w2591) -> ()
              n2002 = local write "1 5"(w2590) -> ()
              n2003 = local write "2 10"(w2589) -> ()
              n2004 = local write "2 7"(w2588) -> ()
              n2005 = local write "2 6"(w2587) -> ()
              n2006 = local write "2 5"(w2586) -> ()
              n2007 = local write "3 9"(w2585) -> ()
              n2008 = local write "3 7"(w2584) -> ()
              n2009 = local write "3 6"(w2583) -> ()
              n2010 = local write "3 5"(w2582) -> ()
              n2011 = local write "4 9"(w2581) -> ()
              n2012 = local write "4 7"(w2580) -> ()
              n2013 = local write "4 6"(w2579) -> ()
              n2014 = local write "4 5"(w2578) -> ()
              n2015 = local write "5 8"(w2577) -> ()
              n2016 = local write "5 7"(w2576) -> ()
              n2017 = local write "5 6"(w2575) -> ()
              n2018 = local write "5 5"(w2574) -> ()
              n2019 = local write "6 8"(w2573) -> ()
              n2020 = local write "6 7"(w2572) -> ()
              n2021 = local write "6 6"(w2571) -> ()
              n2022 = local write "6 5"(w2570) -> ()
              n2023 = Index Array(array=w2596) -> (element #1=w2643:bool, element #2=w2642:bool, element #3=w2641:bool, element #4=w2640:bool, element #5=w2639:bool, element #6=w2638:bool, element #7=w2637:bool, element #8=w2636:bool, element #9=w2635:bool, element #10=w2634:bool, element #11=w2633:bool, element #12=w2632:bool, element #13=w2631:bool, element #14=w2630:bool, element #15=w2629:bool, element #16=w2628:bool, element #17=w2627:bool, element #18=w2626:bool, element #19=w2625:bool, element #20=w2624:bool, element #21=w2623:bool, element #22=w2622:bool, element #23=w2621:bool, element #24=w2620:bool, element #25=w2619:bool, element #26=w2618:bool, element #27=w2617:bool, element #28=w2616:bool, element #29=w2615:bool, element #30=w2614:bool)  [unwired: 30 in]
              n2024 = local write "Adrive"(w2643) -> ()
              n2025 = local write "Ddrive"(w2642) -> ()
              n2026 = local write "ASWdrive"(w2641) -> ()
              n2027 = local write "DSWdrive"(w2640) -> ()
              n2028 = local write "Drop 14"(w2639) -> ()
              n2029 = local write "Chop 13"(w2638) -> ()
              n2030 = local write "Lob"(w2637) -> ()
              n2031 = local write "Boast2"(w2636) -> ()
              n2032 = local write "Boast3"(w2635) -> ()
              n2033 = local write "Smash 13"(w2634) -> ()
              n2034 = local write "FH"(w2633) -> ()
              n2035 = local write "BH"(w2632) -> ()
              n2036 = local write "ST"(w2631) -> ()
              n2037 = local write "CR"(w2630) -> ()
              n2038 = local write "Bounce"(w2629) -> ()
              n2039 = local write "Half Volley"(w2628) -> ()
              n2040 = local write "Volley"(w2627) -> ()
              n2041 = local write "Expected Winner1 2"(w2626) -> ()
              n2042 = local write "Expected Winner2 2"(w2625) -> ()
              n2043 = local write "Unexpected Winner1 2"(w2624) -> ()
              n2044 = local write "Unexpected Winner2 2"(w2623) -> ()
              n2045 = local write "Stroke1 2"(w2622) -> ()
              n2046 = local write "Stroke2 2"(w2621) -> ()
              n2047 = local write "Forced Error1 2"(w2620) -> ()
              n2048 = local write "Forced Error2 2"(w2619) -> ()
              n2049 = local write "Unforced Error1 2"(w2618) -> ()
              n2050 = local write "Unforced Error2 2"(w2617) -> ()
              n2051 = local write "Nolet1 2"(w2616) -> ()
              n2052 = local write "Nolet2 2"(w2615) -> ()
              n2053 = local write "Let 2"(w2614) -> ()
              n2054 = Index Array(array=w2597) -> (element #1=w2613:bool, element #2=w2612:bool, element #3=w2611:bool, element #4=w2610:bool, element #5=w2609:bool, element #6=w2608:bool, element #7=w2607:bool, element #8=w2606:bool, element #9=w2605:bool, element #10=w2604:bool, element #11=w2603:bool, element #12=w2602:bool, element #13=w2601:bool, element #14=w2600:bool, element #15=w2599:bool, element #16=w2569:bool, element #17=w2568:bool, element #18=w2567:bool, element #19=w2566:bool, element #20=w2565:bool)  [unwired: 20 in]
              n2055 = local write "Service1 2"(w2613) -> ()
              n2056 = local write "Service2 2"(w2612) -> ()
              n2057 = local write "S1 2"(w2611) -> ()
              n2058 = local write "S2 2"(w2610) -> ()
              n2059 = local write "S3 2"(w2609) -> ()
              n2060 = local write "S4 2"(w2608) -> ()
              n2061 = local write "S5 2"(w2607) -> ()
              n2062 = local write "S6 2"(w2606) -> ()
              n2063 = local write "Player1 2"(w2605) -> ()
              n2064 = local write "Player2 2"(w2604) -> ()
              n2065 = local write "Button 6"(w2603) -> ()
              n2066 = local write "Button 7"(w2602) -> ()
              n2067 = local write "Button 8"(w2601) -> ()
              n2068 = local write "Button 9"(w2600) -> ()
              n2069 = local write "Button 10"(w2599) -> ()
              n2070 = local write "G1"(w2569) -> ()
              n2071 = local write "G2"(w2568) -> ()
              n2072 = local write "G3"(w2567) -> ()
              n2073 = local write "G4"(w2566) -> ()
              n2074 = local write "G5"(w2565) -> ()
            }
          }
          n2075 = local read "Player 1"() -> (w2425:string)
          n2076 = local read "Player 2"() -> (w2424:string)
          n2077 = call <vilib>:"Trim Whitespace.vi"("string"=w2425) -> ("trimmed string"=w2427:string)  [unwired: 1 in]
          n2078 = call <vilib>:"Trim Whitespace.vi"("string"=w2424) -> ("trimmed string"=w2430:string)  [unwired: 1 in]
          n2079 = Empty String/Path?(string/path=w2427) -> (empty?=w2426:bool)
          n2080 = Empty String/Path?(string/path=w2430) -> (empty?=w2431:bool)
          n2081 = Select(t="Player 1", s=w2426, f=w2427) -> (s? t:f=w2423:string)
          n2082 = Select(t="Player 2", s=w2431, f=w2430) -> (s? t:f=w2422:string)
          n2083 = local read "Btn 10"() -> (w2435:string)
          n2084 = local read "Btn 6"() -> (w2437:string)
          n2085 = local read "Btn 9"() -> (w2436:string)
          n2086 = local read "Btn 7"() -> (w2438:string)
          n2087 = local read "Btn 8"() -> (w2439:string)
          n2088 = Concatenate Strings(w2423, w2417, w2422, w2417, w2437, w2417, w2438, w2417, w2439, w2417, w2436, w2417, w2435, w2417, "Game1" ("t"), w2417, "Game2" ("t"), w2417, "Game3" ("t"), w2417, "Game4" ("t"), w2417, "Game5" ("t")) -> (w2445:string)
          n2089 = for {
            tunnel: string[] ["frame number", "Lead", "Lag", "position 1", "position 2", "position 3", "position 4", "position 5", "position 6", "position 7", "position 8", "position 9", "position 10", "position 11", "position 12", "position 13", "position 14", "position 15", "position 16", "position 17", "position 18", "position 19", "position 20", "position 21", "position 22", "position 23", "position 24", "Drive A", "Drive D", "SW Drive A", "SW Drive D", "drop", "chop", "lob", "boast 2", "boast 3", "kill", "Forehand", "Backhand", "Straight", "Cross", "Bounce", "Half Volley", "Volley", "Expected winner 1", "Expected winner 2", "Unexpected winner 1", "Unexpected winner 2", "Stroke 1", "Stroke 2", "Forced error 1", "Forced error 2", "Unforced error 1", "Unforced error 2", "No let 1", "No let 2", "Let", "point1", "point2", "score1", "score2", "service1", "service2", "s1", "s2", "s3", "s4", "s5", "s6"] ("all rows") -> [w2463] mode=indexing
            tunnel: [w2461] -> w2443 mode=indexing
            n2090 = Concatenate Strings(w2463, "\t") -> (w2461:string)
          }
          n2091 = Concatenate Strings(w2443, w2445, "\r") -> (w2440:string)
          n2092 = Array To Spreadsheet String(delimiter (Tab)="\t" ("delimiter (\\t)"), array=w2442, 3:"%.3f" ("format (%.3f)")) -> (spreadsheet string=w2441:string)
          n2093 = local read "Video file"() -> (w2452:path)
          n2094 = local read "Data file"() -> (w2448:path)
          n2095 = call <vilib>:"Get File Extension.vi"("file"=w2452) -> ("filename without extension"=w2454:string)  [unwired: 7 in, 3 out]
          n2096 = Open/Create/Replace File(file path (use dialog)=w2448, operation (0:open)=T4."replace") -> (refnum out=w2450:refnum<file>, error out=w2449:errorcluster)  [unwired: 4 in, 1 out]
          n2097 = Concatenate Strings("avi file" ("string"), w2455, w2454, w2455, w2455, w2440, w2441) -> (w2456:string)
          n2098 = local write "Update"(FALSE ("Update")) -> ()
          n2099 = Write to Text File(file (use dialog)=w2450, text=w2456, error in=w2449) -> (refnum out=w2433:refnum<file>, error out=w2434:errorcluster)  [unwired: 1 in, 1 out]
          n2100 = Close File(refnum=w2433, error in=w2434) -> ()  [unwired: 2 out]
        }
      }
      n2101 = Equal?(x="Main tab", y=enum32{"Coding", "Display"}."Coding" ("Tab Control 3")) -> (x = y?=w387:bool)
      n2102 = Not Equal?(x=w377, y=w382) -> (x != y?=w386:bool)
      n2103 = Select(t=w382, s=w387, f=w384) -> (s? t:f=w376:T6)
      n2104 = And(x=w386, y=w387) -> (x .and. y?=w385:bool)
      n2105 = Equal?(x=w377, y=w382) -> (x = y?=w381:bool)
      n2106 = Equal?(x=w376, y=w384) -> (x = y?=w383:bool)
      n2107 = And(x=w383, y=w381) -> (x .and. y?=w380:bool)
      n2108 = case shown="True" w385 {
        tunnel: w379 -> [_ w396]
        frame False {
        }
        frame True {
          # "Moving back to coding tab"
          n2109 = flat-sequence {
            tunnel: w396 -> [w400]
            frame #0 {
              n2110 = local read "ful video frames"() -> (w401:i64[])
              n2111 = Index Array(array=w400, index (col)=0 ("disabled index (col)")) -> (element=w398:i64[])  [unwired: 1 in]
              n2112 = Array Max & Min(array=w398) -> (max value=w397:i64)  [unwired: 3 out]
              n2113 = local write "frames 2 play"(w401) -> ()
              n2114 = local write "Progress..."(w397) -> ()
            }
            frame #1 {
              w402 = FALSE ("Next")
              w403 = TRUE ("Play")
              n2115 = local write "stop"(w403) -> ()
              n2116 = local write "Load video"(w403) -> ()
              n2117 = local write "clear all"(w402) -> ()
              n2118 = local write "Pause"(w402) -> ()
              n2119 = local write "Update"(w402) -> ()
              n2120 = local write "Next"(w402) -> ()
              n2121 = local write "Previous"(w402) -> ()
              n2122 = local write "Reset"(w402) -> ()
              n2123 = local write "Extract data"(w402) -> ()
              n2124 = local write "Upload edited video"(w402) -> ()
              n2125 = local write "Examine code"(w402) -> ()
            }
          }
        }
      }
      n2126 = case shown="True" w380 {
        frame False {
        }
        frame True {
          n2127 = local write "Progress..."(u32 0 ("Progress...")) -> ()
          n2128 = local write "Pause"(FALSE ("Pause")) -> ()
          n2129 = local write "stop"(TRUE ("stop")) -> ()
        }
      }
      n2130 = local read "START"() -> (w378:bool)
      n2131 = Wait (ms)(milliseconds to wait=u32 200) -> ()  [unwired: 1 out]
      "Main tab 2" <- w377
    }
    n2132 = while {
      tunnel: w9 -> [w214]
      tunnel: w2 -> [_]
      tunnel: [w209] -> w6
      stop <- w209 continue-if-true
      # "This loop is for writing\nvideo to disk"
      n2133 = local read "Video files to write"() -> (w213:string[])
      n2134 = local read "frames to write"() -> (w211:i64[][])
      n2135 = case shown="False" "Write file" {
        tunnel: [FALSE FALSE] -> w216
        tunnel: w214 -> [_ w234]
        tunnel: w213 -> [_ w233]
        tunnel: "Video to write" -> [_ w232]
        tunnel: w211 -> [_ w231]
        tunnel: [u32 0 ("milliseconds to wait") u32 0 ("milliseconds to wait")] -> w210
        frame False {
          w218 = T5."Enabled" ("Disabled")
          n2136 = local read "Video files to write"() -> (w222:string[])
          n2137 = property on="Add to lib" class="Bool (strict)"("DisabledEnum"=w218) -> ()  [unwired: 2 in, 2 out]
          n2138 = property on="File name" class="Str"("DisabledEnum"=w218) -> ()  [unwired: 2 in, 2 out]
          n2139 = property on="Video to write" class="Path"("DisabledEnum"=w218) -> ()  [unwired: 2 in, 2 out]
          n2140 = property on="START" class="Bool (strict)"("DisabledEnum"=w218) -> ()  [unwired: 2 in, 2 out]
          n2141 = Empty Array?(array=w222) -> (empty?=w221:bool)
          n2142 = Select(t=T5."Disabled and Grayed Out" ("Disabled"), s=w221, f=w218) -> (s? t:f=w219:T5)
          n2143 = property on="Write file" class="Bool (strict)"("DisabledEnum"=w219) -> ()  [unwired: 2 in, 2 out]
          n2144 = local write "Abort"(FALSE ("Abort")) -> ()
        }
        frame True {
          w226 = T5."Disabled and Grayed Out" ("Disabled")
          n2145 = for {
            tunnel: w231 -> [w273] mode=indexing
            tunnel: w233 -> [w264] mode=indexing
            tunnel: w232 -> [w263]
            tunnel: w234 -> [w251]
            tunnel: [w245] -> w229
            tunnel: [w244] -> w228
            tunnel: [w242] -> w227
            i -> [w246]
            stop <- w243 stop-if-true
            w260 = T8 4 items=["Grayscale (U8)", "Grayscale (I16)", "Grayscale (SGL)", "Complex (CSG)", "RGB (U32)", "HSL (U32)", "RGB (U64)"] ("Image Type")
            n2146 = Path To String(path=w263) -> (string=w265:string)
            n2147 = for {
              tunnel: w273 -> [w311] mode=indexing
              tunnel: [w311] -> w250 mode=indexing if=w310
              n2148 = Not Equal To 0?(x=w311) -> (x != 0?=w310:bool)
            }
            n2149 = Concatenate Strings(w265, "\\" ("string"), w264) -> (w268:string)
            n2150 = Array Size(array=w250) -> (size(s)=w249:i32)
            n2151 = Decrement(x=w246) -> (x-1=w247:i32)
            n2152 = Not Equal To 0?(x=w246) -> (x != 0?=w248:bool)
            n2153 = call <vilib>:"Search and Replace Pattern.vi"("string"=w268, "regular expression (\"\")"=".avi" ("regular expression (\"\")")) -> ("result string"=w272:string)  [unwired: 3 in, 1 out]
            n2154 = case shown="True" w248 {
              tunnel: w247 -> [_ w283]
              frame False {
              }
              frame True {
                n2155 = local read "Video files to write"() -> (w287:string[])
                n2156 = local read "frames to write"() -> (w284:i64[][])
                n2157 = Delete From Array(array=w287, index=w283) -> (array with subset deleted=w286:string[])  [unwired: 1 in, 1 out]
                n2158 = Delete From Array(array=w284, index (row)=w283) -> (array with subset deleted=w285:i64[][])  [unwired: 2 in, 1 out]
                n2159 = local write "frames to write"(w285) -> ()
                n2160 = local write "Video files to write"(w286) -> ()
              }
            }
            n2161 = property on="Writing" class="Slide (strict)"("Scale.Maximum"=w249) -> ()  [unwired: 2 in, 2 out]
            n2162 = Concatenate Strings(w272, ".avi" ("string")) -> (w270:string)
            n2163 = String To Path(string=w270) -> (path=w271:path)
            n2164 = while {
              shift-right: [w291] -> _
              shift-left: w271 -> [w290]
              tunnel: w272 -> [w295]
              tunnel: [w290] -> w241
              i -> [w289]
              stop <- w297 continue-if-true
              n2165 = Increment(x=w289) -> (x+1=w288:i32)
              n2166 = call <vilib>:"Check if File or Folder Exists.vi"("path"=w290) -> ("file or folder exists?"=w297:bool)  [unwired: 8 in, 2 out]
              n2167 = Number To Decimal String(number=w288) -> (decimal integer string=w294:string)  [unwired: 1 in]
              n2168 = Concatenate Strings(w295, " (file path clash) - " ("string"), w294, ".avi" ("string")) -> (w292:string)
              n2169 = String To Path(string=w292) -> (path=w291:path)
            }
            n2170 = Select(t="Microsoft Video 1" ("Codec Name"), s="Video compress", f="" ("Codec Name")) -> (s? t:f=w238:string)
            n2171 = local read "framesPerSecond"() -> (w254:u32)
            n2172 = call "IMAQ AVI Create"("Compression Filter"=w238, "Frames Per Second"=w254, "AVI Path"=w241) -> ("error out"=w261:errorcluster, "Avi Refnum"=w255:T9)  [unwired: 7 in]
            n2173 = call "IMAQ Create"("Image Name"="write", "Image Type"=w260, "error in (no error)"=w261) -> ("New Image"=w259:T1, "error out"=w258:errorcluster)  [unwired: 2 in]
            n2174 = for {
              tunnel: w250 -> [w308] mode=indexing
              tunnel: w259 -> [w302]
              tunnel: w258 -> [w307]
              tunnel: [w305] -> w257
              tunnel: [w304] -> w256
              tunnel: w255 -> [w303]
              tunnel: [w302] -> w252
              tunnel: w251 -> [w301]
              tunnel: ["Abort"] -> w243
              i -> [w300]
              stop <- "Abort" stop-if-true
              n2175 = Increment(x=w300) -> (x+1=→"Writing":i32)
              n2176 = call "IMAQ AVI Read Frame"("error in (no error)"=w307, "Frame Number"=w308, "Image"=w302, "Avi Refnum"=w301) -> ("error out"=w309:errorcluster, "Image Out"=w306:T1)  [unwired: 4 in, 2 out]
              n2177 = call "IMAQ AVI Write Frame"("error in (no error)"=w309, "Image"=w306, "Avi Refnum"=w303) -> ("error out"=w304:errorcluster, "Avi Refnum (duplicate)"=w305:T9)  [unwired: 7 in]
            }
            n2178 = call "IMAQ AVI Close"("error in (no error)"=w256, "Avi Refnum"=w257) -> ("error out"=w253:errorcluster)  [unwired: 9 in]
            n2179 = call "IMAQ Dispose"("Image"=w252, "error in (no error)"=w253) -> ("error out"=w240:errorcluster)  [unwired: 4 in]
            n2180 = case shown="False" w243 {
              tunnel: [string[] [] ("Video files to write") w281] -> w245
              tunnel: [i64[][] [] ("to write") w280] -> w244
              tunnel: ["Writing Complete" ("message") "Writing aborted" ("message")] -> w242
              tunnel: w241 -> [_ w278]
              tunnel: w240 -> [_ w277]
              frame False {
              }
              frame True {
                n2181 = local read "Video files to write"() -> (w281:string[])
                n2182 = Delete(path (use dialog)=w278, error in=w277) -> ()  [unwired: 3 in, 3 out]
                n2183 = local read "frames to write"() -> (w280:i64[][])
                n2184 = local write "Abort"(FALSE ("Abort")) -> ()
              }
            }
          }
          n2185 = One Button Dialog(message=w227) -> ()  [unwired: 1 in, 1 out]
          n2186 = local write "Video files to write"(w229) -> ()
          n2187 = local write "frames to write"(w228) -> ()
          n2188 = property on="Add to lib" class="Bool (strict)"("DisabledEnum"=w226) -> ()  [unwired: 2 in, 2 out]
          n2189 = property on="File name" class="Str"("DisabledEnum"=w226) -> ()  [unwired: 2 in, 2 out]
          n2190 = property on="Video to write" class="Path"("DisabledEnum"=w226) -> ()  [unwired: 2 in, 2 out]
          n2191 = property on="START" class="Bool (strict)"("DisabledEnum"=w226) -> ()  [unwired: 2 in, 2 out]
        }
      }
      n2192 = local read "START"() -> (w209:bool)
      n2193 = local write "Write file"(w216) -> ()
      n2194 = local write "Writing"(w210) -> ()
      n2195 = Wait (ms)(milliseconds to wait=u32 200) -> ()  [unwired: 1 out]
    }
    n2196 = flat-sequence {
      tunnel: w6 -> [_]
      tunnel: w5 -> [w31]
      frame #0 {
        w27 = T8 4 items=["Grayscale (U8)", "Grayscale (I16)", "Grayscale (SGL)", "Complex (CSG)", "RGB (U32)", "HSL (U32)", "RGB (U64)"] ("Image Type")
        w28 = T8 4 items=["Grayscale (U8)", "Grayscale (I16)", "Grayscale (SGL)", "Complex (CSG)", "RGB (U32)", "HSL (U32)", "RGB (U64)"] ("Image Type")
        w30 = T8 4 items=["Grayscale (U8)", "Grayscale (I16)", "Grayscale (SGL)", "Complex (CSG)", "RGB (U32)", "HSL (U32)", "RGB (U64)"] ("Image Type")
        n2197 = call "IMAQ AVI Close"("Avi Refnum"=w31) -> ("error out"=w16:errorcluster)  [unwired: 10 in]
        n2198 = call "IMAQ Create"("Image Name"="Video", "Image Type"=w27, "error in (no error)"=w16) -> ("New Image"=w22:T1, "error out"=w25:errorcluster)  [unwired: 2 in]
        n2199 = call "IMAQ Create"("Image Name"="pauselag", "Image Type"=w30, "error in (no error)"=w25) -> ("New Image"=w21:T1, "error out"=w23:errorcluster)  [unwired: 2 in]
        n2200 = call "IMAQ Create"("Image Name"="write", "Image Type"=w28, "error in (no error)"=w23) -> ("New Image"=w20:T1, "error out"=w19:errorcluster)  [unwired: 2 in]
        n2201 = call "IMAQ Dispose"("Image"=w22, "error in (no error)"=w19) -> ("error out"=w18:errorcluster)  [unwired: 4 in]
        n2202 = call "IMAQ Dispose"("Image"=w21, "error in (no error)"=w18) -> ("error out"=w17:errorcluster)  [unwired: 4 in]
        n2203 = call "IMAQ Dispose"("Image"=w20, "error in (no error)"=w17) -> ()  [unwired: 4 in, 1 out]
      }
    }
    n2204 = Wait (ms)(milliseconds to wait=u32 100) -> ()  [unwired: 1 out]
  }
  n2205 = while {
    stop <- FALSE stop-if-true
    n2206 = event shown="[2] Key Down" {
      selector: _ -> [_ _ _]
      dyn-events: _ -> [_ _ _]
      timeout: 100 -> [_ _ _]
      event Timeout {
        n2207 = event-data() -> ()  [unwired: 1 in, 3 out]
        n2208 = local write "fast forward"(FALSE ("fast forward")) -> ()
        n2209 = local write "fast rewind"(FALSE ("fast rewind")) -> ()
      }
      event Key Repeat {
        n2210 = event-data() -> ("VKey"=w2651:T11)  [unwired: 1 in, 9 out]
        n2211 = case shown="\"Right\"" w2651 {
          frame "ASCII", Default {
          }
          frame "Enter" {
          }
          frame "Return" {
          }
          frame "Shift" {
          }
          frame "Ctrl" {
          }
          frame "Alt" {
          }
          frame "Cmd" {
          }
          frame "Opt" {
          }
          frame "Caps" {
          }
          frame "NumLock" {
          }
          frame "Clear" {
          }
          frame "Break" {
          }
          frame "Up" {
          }
          frame "Down" {
          }
          frame "Left" {
            n2212 = local write "fast rewind"(TRUE ("fast rewind")) -> ()
          }
          frame "Right" {
            n2213 = local write "fast forward"(TRUE ("fast forward")) -> ()
          }
          frame "Insert" {
          }
          frame "Delete" {
          }
          frame "Home" {
          }
          frame "End" {
          }
          frame "PageUp" {
          }
          frame "PageDown" {
          }
          frame "Escape" {
          }
          frame "Help" {
          }
          frame "Pause" {
          }
          frame "ScrollLock" {
          }
          frame "F1" {
          }
          frame "F2" {
          }
          frame "F3" {
          }
          frame "F4" {
          }
          frame "F5" {
          }
          frame "F6" {
          }
          frame "F7" {
          }
          frame "F8" {
          }
          frame "F9" {
          }
          frame "F10" {
          }
          frame "F11" {
          }
          frame "F12" {
          }
          frame "F13" {
          }
          frame "F14" {
          }
          frame "F15" {
          }
          frame "F16" {
          }
          frame "F17" {
          }
          frame "F18" {
          }
          frame "F19" {
          }
          frame "F20" {
          }
          frame "F21" {
          }
          frame "F22" {
          }
          frame "F23" {
          }
          frame "F24" {
          }
          frame "Play" {
          }
          frame "VolumeUp" {
          }
          frame "VolumeDown" {
          }
          frame "Mute" {
          }
          frame "Two Byte Char" {
          }
        }
      }
      event Key Down {
        n2214 = event-data() -> ("Char"=w2659:i16, "VKey"=w2667:T11)  [unwired: 1 in, 8 out]
        n2215 = property on="Video to write" class="Path"() -> ("Key Focus"=w2657:bool)  [unwired: 2 in, 2 out]
        n2216 = property on="Btn 2" class="Str"() -> ("Key Focus"=w2671:bool)  [unwired: 2 in, 2 out]
        n2217 = property on="Btn 3" class="Str"() -> ("Key Focus"=w2670:bool)  [unwired: 2 in, 2 out]
        n2218 = property on="Btn 4" class="Str"() -> ("Key Focus"=w2669:bool)  [unwired: 2 in, 2 out]
        n2219 = property on="Btn 5" class="Str"() -> ("Key Focus"=w2672:bool)  [unwired: 2 in, 2 out]
        n2220 = property on="Btn 1" class="Str"() -> ("Key Focus"=w2673:bool)  [unwired: 2 in, 2 out]
        n2221 = property on="File name" class="Str"() -> ("Key Focus"=w2656:bool)  [unwired: 2 in, 2 out]
        n2222 = property on="Player 2" class="Str"() -> ("Key Focus"=w2655:bool)  [unwired: 2 in, 2 out]
        n2223 = property on="Player 1" class="Str"() -> ("Key Focus"=w2654:bool)  [unwired: 2 in, 2 out]
        n2224 = Compound Arithmetic op=OR(w2654, w2655, w2671, w2670, w2669, w2672, w2673, w2657, w2656) -> (w2674:bool)
        n2225 = Not(x=w2674) -> (.not. x?=w2661:bool)
        n2226 = Equal?(x=i16 102, y=w2659) -> (x = y?=w2664:bool)
        n2227 = And(x=w2664, y=w2661) -> (x .and. y?=w2662:bool)
        n2228 = Equal?(x=i16 32, y=w2659) -> (x = y?=w2658:bool)
        n2229 = case shown="True" w2662 {
          frame False {
          }
          frame True {
            w2678 = "1" ("display\nselection")
            n2230 = local read "display\nselection"() -> (w2680:string)
            n2231 = Equal?(x=w2680, y=w2678) -> (x = y?=w2679:bool)
            n2232 = Select(t="2" ("display\nselection"), s=w2679, f=w2678) -> (s? t:f=w2676:string)
            n2233 = local write "display\nselection"(w2676) -> ()
          }
        }
        n2234 = Equal?(x=i16 100, y=w2659) -> (x = y?=w2665:bool)
        n2235 = And(x=w2658, y=w2661) -> (x .and. y?=w2668:bool)
        n2236 = And(x=w2665, y=w2661) -> (x .and. y?=w2660:bool)
        n2237 = case shown="\"Escape\"" w2667 {
          frame "ASCII", Default {
          }
          frame "Enter" {
          }
          frame "Return" {
          }
          frame "Shift" {
          }
          frame "Ctrl" {
          }
          frame "Alt" {
          }
          frame "Cmd" {
          }
          frame "Opt" {
          }
          frame "Caps" {
          }
          frame "NumLock" {
          }
          frame "Clear" {
          }
          frame "Break" {
          }
          frame "Up" {
          }
          frame "Down" {
          }
          frame "Left" {
          }
          frame "Right" {
          }
          frame "Insert" {
          }
          frame "Delete" {
          }
          frame "Home" {
          }
          frame "End" {
          }
          frame "PageUp" {
          }
          frame "PageDown" {
          }
          frame "Escape" {
            n2238 = local write "Undo"(TRUE ("Undo")) -> ()
          }
          frame "Help" {
          }
          frame "Pause" {
          }
          frame "ScrollLock" {
          }
          frame "F1" {
          }
          frame "F2" {
          }
          frame "F3" {
          }
          frame "F4" {
          }
          frame "F5" {
          }
          frame "F6" {
          }
          frame "F7" {
          }
          frame "F8" {
          }
          frame "F9" {
          }
          frame "F10" {
          }
          frame "F11" {
          }
          frame "F12" {
          }
          frame "F13" {
          }
          frame "F14" {
          }
          frame "F15" {
          }
          frame "F16" {
          }
          frame "F17" {
          }
          frame "F18" {
          }
          frame "F19" {
          }
          frame "F20" {
          }
          frame "F21" {
          }
          frame "F22" {
          }
          frame "F23" {
          }
          frame "F24" {
          }
          frame "Play" {
          }
          frame "VolumeUp" {
          }
          frame "VolumeDown" {
          }
          frame "Mute" {
          }
          frame "Two Byte Char" {
          }
        }
        n2239 = case shown="True" w2660 {
          frame False {
          }
          frame True {
            n2240 = property on="Tab Control" class="TabCtl (strict)"() -> ("Visible"=w2682:bool)  [unwired: 2 in, 2 out]
            n2241 = Not(x=w2682) -> (.not. x?=w2681:bool)
            n2242 = property on="Tab Control" class="TabCtl (strict)"("Visible"=w2681) -> ()  [unwired: 2 in, 2 out]
          }
        }
        n2243 = case shown="True" w2668 {
          frame False {
          }
          frame True {
            n2244 = local read "Pause"() -> (w2685:bool)
            n2245 = Not(x=w2685) -> (.not. x?=w2684:bool)
            n2246 = local write "Pause"(w2684) -> ()
          }
        }
      }
    }
  }
  n2247 = local write "G5"(w1) -> ()
  n2248 = local write "G4"(w1) -> ()
  n2249 = local write "G1"(w1) -> ()
  n2250 = local write "G2"(w1) -> ()
  n2251 = local write "G3"(w1) -> ()
